vi "EC_Applied_Motion_SXSYSZ_20120115.vi"() -> ()   [LabVIEW 2010]
uses:
  <vilib>/Utility/file.llb/Read From Spreadsheet File (I64).vi
  <vilib>/Utility/file.llb/Read From Spreadsheet File (string).vi
  <vilib>/Instr/_visa.llb/VISA Configure Serial Port (Instr).vi
  <vilib>/Utility/file.llb/Write To Spreadsheet File (I64).vi
  <vilib>/Utility/file.llb/Write To Spreadsheet File (string).vi
panel:
  out "R Velocity MVdeg/sec":dbl format="%.3f"
  out "R Position MV deg":dbl
  out "Z Velocity MV mm/sec":dbl format="%.3f"
  out "Z Position MV mm":dbl
  out "Y Velocity MV mm/sec":dbl format="%.3f"
  out "Y Position MV mm":dbl
  out "X Velocity MV mm/sec":dbl format="%.3f"
  out "X Position MV mm":dbl
  out "Presets":i32[][](array[numeric])
  in  "stop":bool
  in  "Tab Control 3":enum32{"Status", "Reset"}(tab)
  out "Y in Range":bool
  out "Y Scan":bool
  out "Y in Motion":bool
  out "Y Backlash corr":bool
  out "X  in Range":bool
  out "X Scan":bool
  out "X  in Motion":bool
  out "X Backlash corr":bool
  out "Z in Range":bool
  out "Z Scan":bool
  out "Z in Motion":bool
  out "Z Backlash corr":bool
  out "R in Range":bool
  out "R Scan":bool
  out "R in Motion":bool
  out "R Backlash corr":bool
  out "X Ready":bool
  out "Y Ready":bool
  out "Z Ready":bool
  out "R Ready":bool
  in  "Reset Y Position mm":dbl
  out "Reset Y Motor Steps":i32
  in  "Reset X Position mm":dbl
  out "Reset X Motor Steps":i32
  in  "Reset Z Position mm":dbl
  out "Reset Z Motor Steps":i32
  in  "Reset R Position deg":dbl
  out "Reset R Motor Steps":i32
  in  "Reset":bool
  in  "Tab Control 2":enum32{"mm", "step"}(tab)
  in  "X Scan Length SP mm":dbl
  in  "X Scan Velocity SP mm/sec":dbl
  in  "X Scan set":bool
  in  "Y Scan Length SP mm":dbl
  in  "Y Scan Velocity SP mm/sec":dbl
  in  "Y Scan set":bool
  in  "Z Scan Length SP mm":dbl
  in  "Z Scan Velocity SP mm/sec":dbl
  in  "Z Scan set":bool
  in  "R Scan Length SP deg":dbl
  in  "R Scan Velocity SP deg/sec":dbl
  in  "R Scan set":bool
  in  "X Scan Velocity SP steps/sec":i32=1 min=1 max=102400 step=1
  in  "X Scan Length SP steps":i32 min=-500000 max=500000 step=100
  out "X Scan length MV mm":dbl
  out "X Scan velocity MV mm/sec":dbl format="%#_6f"
  in  "Y Scan Velocity SP steps/sec":i32=1 min=1 max=102400 step=1
  in  "Y Scan Length SP steps":i32 min=-1000000 max=0 step=100
  out "Y Scan length MV mm":dbl
  out "Y Scan velocity MV mm/sec":dbl format="%#_6f"
  in  "Z Scan Velocity SP steps/sec":i32=1 min=1 max=102400 step=1
  in  "Z Scan Length SP steps":i32 min=-204724 max=102195276 step=100
  out "Z Scan length MV mm":dbl
  out "Z Scan velocity MV mm/sec":dbl format="%#_6f"
  in  "R Scan Velocity SP steps/sec":i32=1 min=1 max=102400 step=1
  in  "R Scan Length SP steps":i32 min=-6144000 max=0 step=100
  out "R Scan length MV deg":dbl
  out "R Scan velocity MV deg/sec":dbl format="%#_6f"
  out "atan Y/Z":dbl
  in  "Tab Control":enum32{"mm", "preset", "step"}(tab)
  in  "X Position SP mm":dbl
  in  "X Velocity SP mm/sec":dbl
  in  "X Move Set":bool
  in  "Y Move Set":bool
  in  "Y Position SP mm":dbl
  in  "Y Velocity SP mm/sec":dbl
  in  "Z Position SP mm":dbl
  in  "Z Velocity SP mm/sec":dbl
  in  "Z Move Set":bool
  in  "R Position SP deg":dbl
  in  "R Velocity SP deg/sec":dbl
  in  "R Move Set":bool
  in  "Add Button":bool
  in  "String":string
  in  "Delete Button":bool
  in  "Preset positions":i32(ring) items=["ZERO", "Default", "CDOSE", "QMS", "test", "test2", "test3"]
  in  "Set Button":bool
  in  "X Velocity SP step/sec":i32 min=1 max=50000
  in  "Y Velocity SP step/sec":i32 min=1 max=50000
  in  "Z Velocity SP step/sec":i32 min=1 max=5000
  in  "R Velocity SP step/sec":i32 min=1 max=10000
  in  "Y Step SP":i32=-20000 min=-800000 max=800000 step=500
  in  "X Step SP":i32=-20000 min=-750000 max=750000 step=500
  in  "Z Step SP":i32=-20000 min=0 max=102400000 step=500
  in  "R Step SP":i32=-20000 min=-6144000 max=0 step=500
  out "X Step PV":i32 max=2000
  out "Y Step PV":i32 max=2000
  out "Z Step PV":i32 max=2000
  out "R Step PV":i32 max=2000
  out "X Scan Duration":dbl
  out "Y Scan Duration":dbl
  out "Z Scan Duration":dbl
  out "R Scan Duration":dbl
  out "R Backlash steps/sec":i32
  out "R Backlash":i32
  out "R Holding Current %":i32
  out "R Run Current %":i32
  out "R offset deg":dbl
  out "R deg/rev":dbl
  out "R steps/rev":u32
  out "R velocity PV step/sec":i32
  out "R MINPOS":i32=-94296
  out "R MAXPOS":i32=-34296
  out "R COM PORT":refnum<visa-resource-name>="COM5"
  in  "R Scan OK":bool
  in  "R Go":bool
  out "R Position deg PV":dbl
  out "Z COM PORT":refnum<visa-resource-name>="COM5"
  out "Z Backlash steps/sec":i32
  out "Z Backlash":i32
  out "Z Holding Current %":i32
  out "Z Run Current %":i32
  out "Z offset mm":dbl
  out "Z mm/rev":dbl
  out "Z steps/rev":u32
  out "Z  velocity PV step/sec":i32
  out "Z MINPOS":i32=-94296
  out "Z MAXPOS":i32=-34296
  in  "Z Scan OK":bool
  in  "Z Go":bool
  out "Z Position mm PV":dbl
  out "X Position mm PV":dbl
  out "X velocity PV step/sec":i32
  in  "X Scan OK":bool
  in  "X Go":bool
  out "X Backlash steps/sec":i32
  out "X Backlash":i32
  out "X Holding Current %":i32
  out "X Run Current %":i32
  out "X offset mm":dbl
  out "X mm/rev":dbl
  out "X steps/rev":u32
  out "X MAXPOS":i32=-34296
  out "X MINPOS":i32=-94296
  out "X COM PORT":refnum<visa-resource-name>="COM5"
  out "Y Backlash steps/sec":i32
  out "Y Backlash":i32
  out "Y Holding Current %":i32
  out "Y Run Current %":i32
  in  "Scan Cancel":bool
  out "Y Position mm PV":dbl
  out "Y offset mm":dbl
  out "Y mm/rev":dbl
  out "Y steps/rev":u32
  out "Y velocity PV step/sec":i32
  in  "Y Scan OK":bool
  in  "Scan Go":bool
  in  "Stop":bool
  in  "Y Go":bool
  out "Y MINPOS":i32=-94296
  out "Y MAXPOS":i32=-34296
  out "Y COM PORT":refnum<visa-resource-name>="COM5"
  # "Current position"
  # "Goto position"
  # "RX"
  # "RX"
  # "RY"
  # "RY"
  # "RZ"
  # "RZ"
  # "RR"
  # "L"
  # "M"
  # "B"
  # "S"
  # "R"
  # "Preset position"
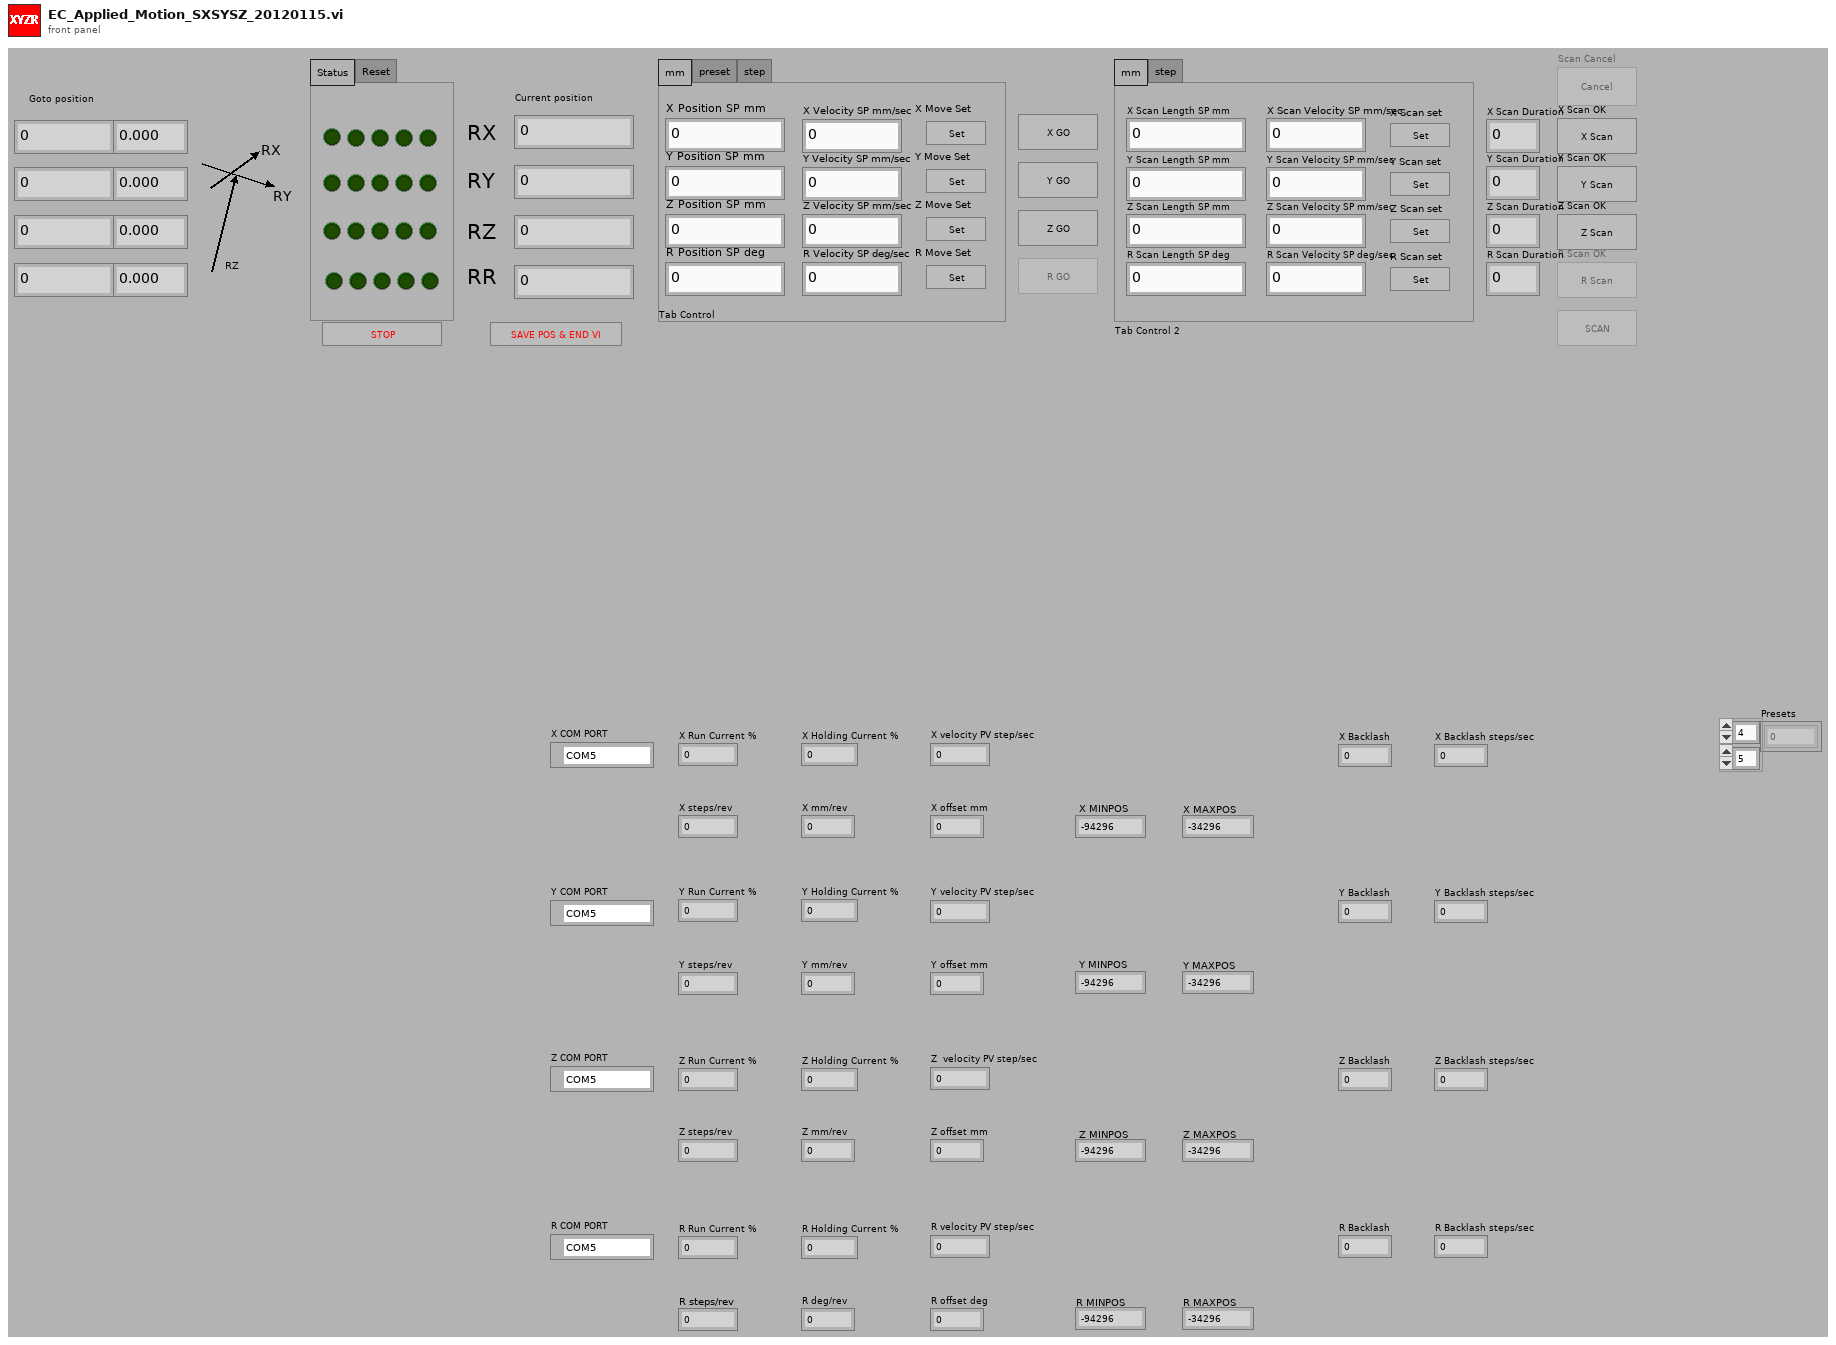
[diagram p1: front panel]
types:
  T1 = enum16{"Power-up Signature", "Accel Rate", "Accel Max", "Bit Rate", "Buffer Status", "Change Current", "Commence Jogging", "Change Jog Speed", "Continue", "Define Address", "Distance for FC,FM,FO,FY", "Decel Rate", "Distance or Position", "Define Limits", "Encoder Deadband", "Encoder Function", "Encoder Position", "Encoder Ratio", "Feed to Length with Speed Change", "Feed to Length", "Feed to Sensor with Mask Dist", "Feed to Length & Set Output", "Feed to Position", "Feed to Sensor", "Feed to Sensor w/safety", "Follow Handwheel", "Immediate Distance?", "Immediate Encoder?", "Immediate Low Output", "Immediate High Output", "Immediate Position?", "Input Status?", "Jog Accel/Decel", "Jog Disable", "Jog Enable", "Jog Speed", "Motor Disable", "Motor Enable", "Microstep Resolution", "Power up Current", "Power up Mode", "Pause", "Request Status", "Revision Level?", "Seek Home", "Stop Jogging", "Stop & Kill Buffer", "Set Output", "Set ABS Position", "Send String", "Stop", "Velocity for Speed Change", "Velocity Setting", "Wait for Input", "Wait Time"}
  T2 = enum8{"Enabled", "Disabled", "Disabled and Grayed Out"}
  T3 = cluster{"first row[0]":i64, "first row[1]":i64, "first row[2]":i64, "first row[3]":i64, "first row[4]":i64, "first row[5]":i64, "first row[6]":i64, "first row[7]":i64, "first row[8]":i64}
  T4 = cluster{"Value[0]":i32, "Value[1]":i32, "Value[2]":i32, "Value[3]":i32, "Value[4]":i32, "Value[5]":i32, "Value[6]":i32, "Value[7]":i32, "Value[8]":i32}
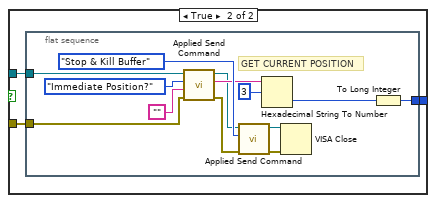
[diagram p2: hidden frame]
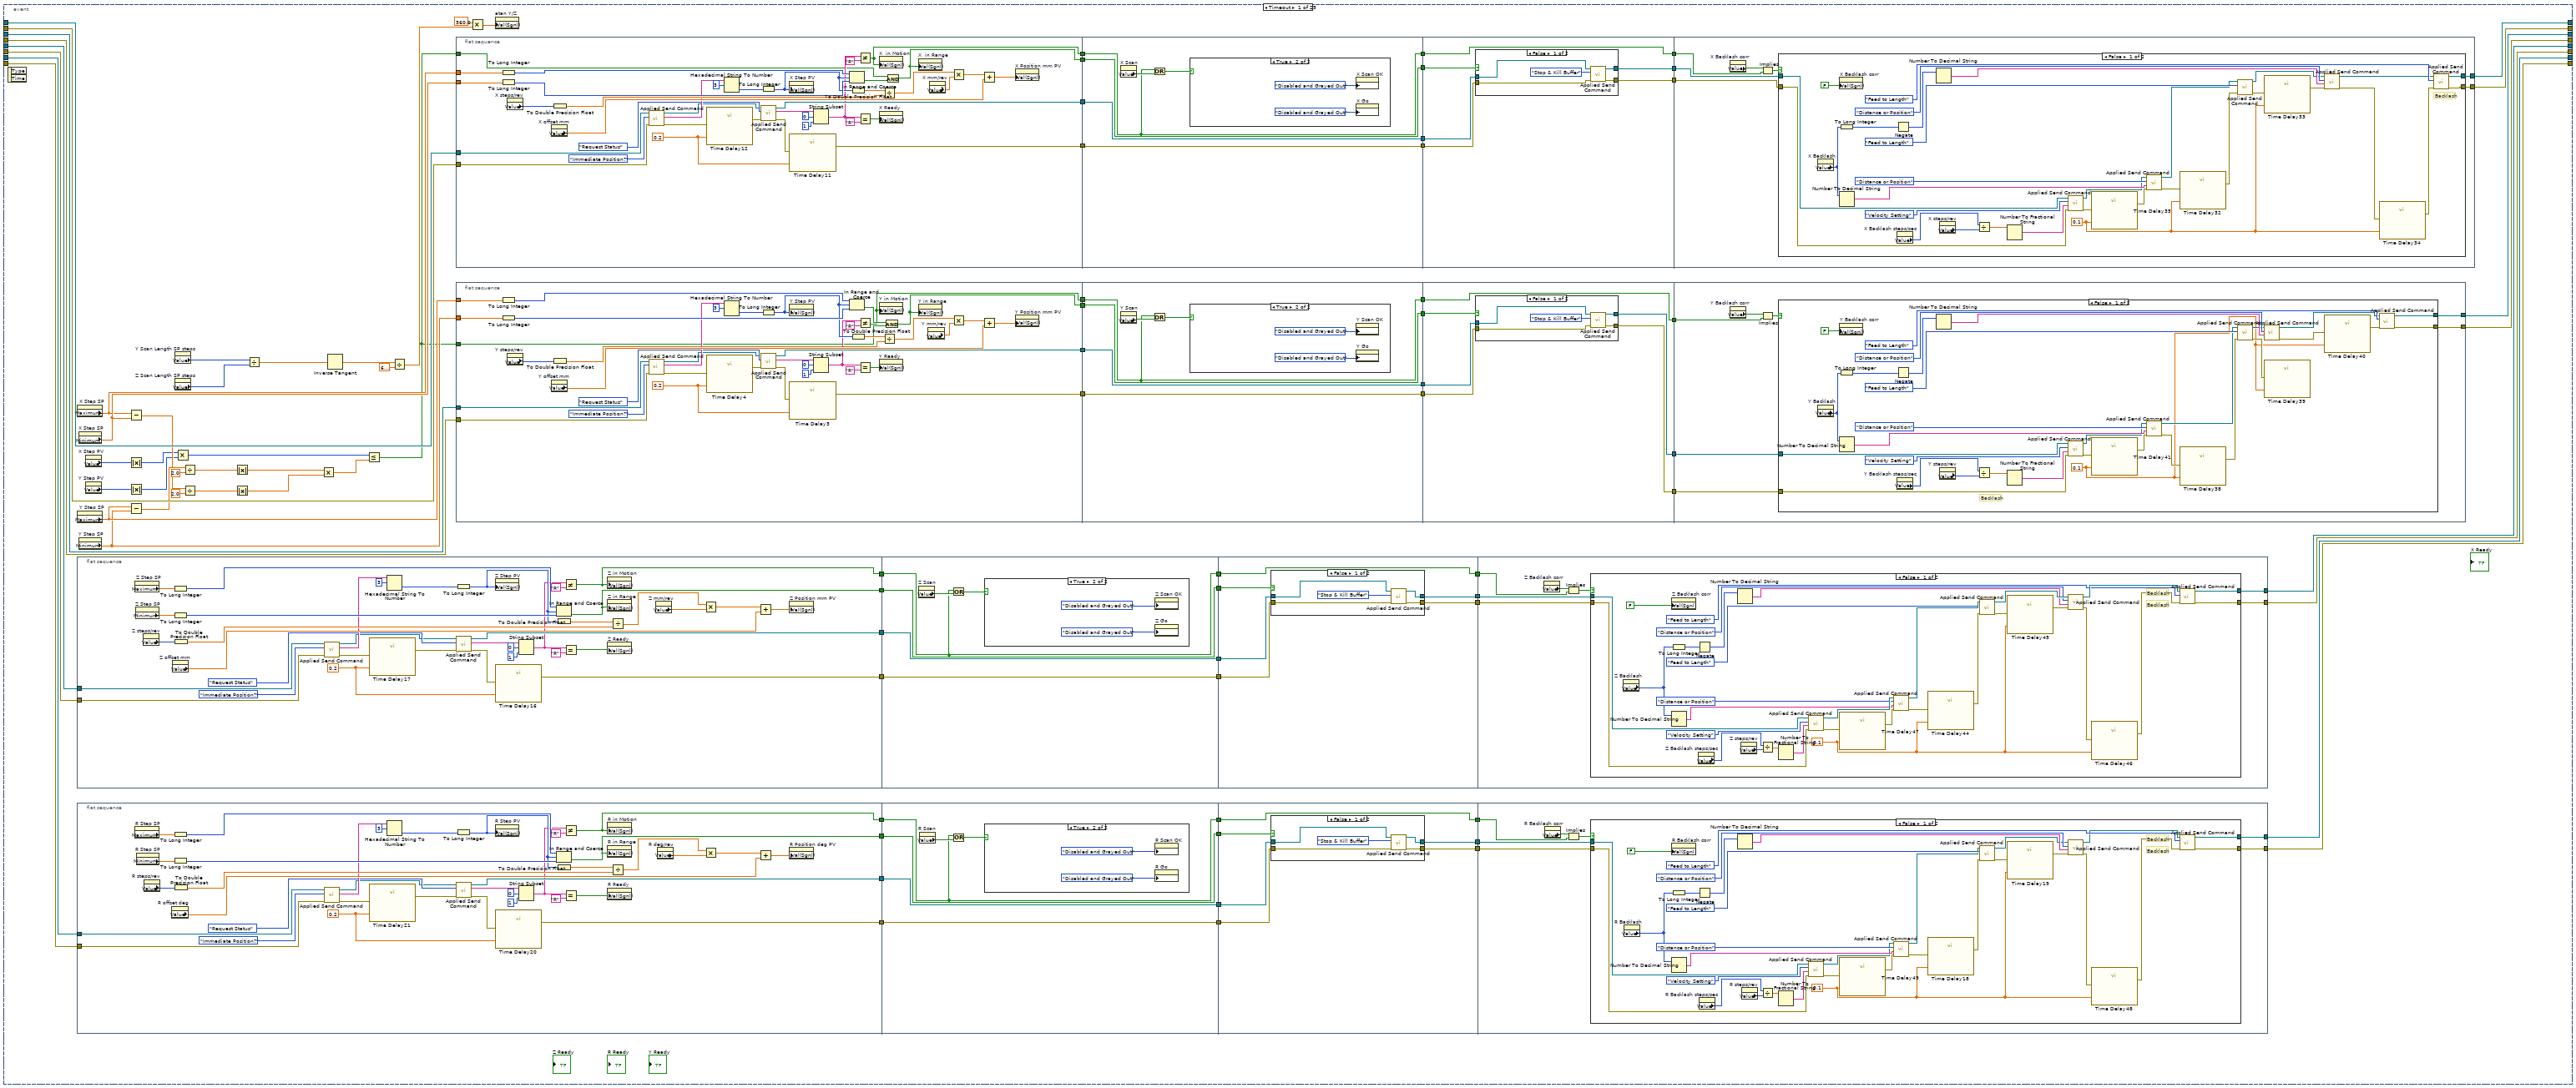
[diagram p6: hidden frame]
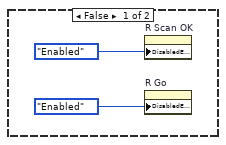
[diagram p7: hidden frame]
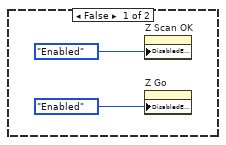
[diagram p10: hidden frame]
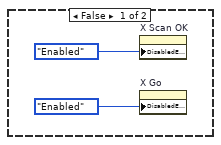
[diagram p13: hidden frame]
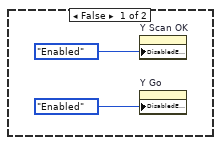
[diagram p16: hidden frame]
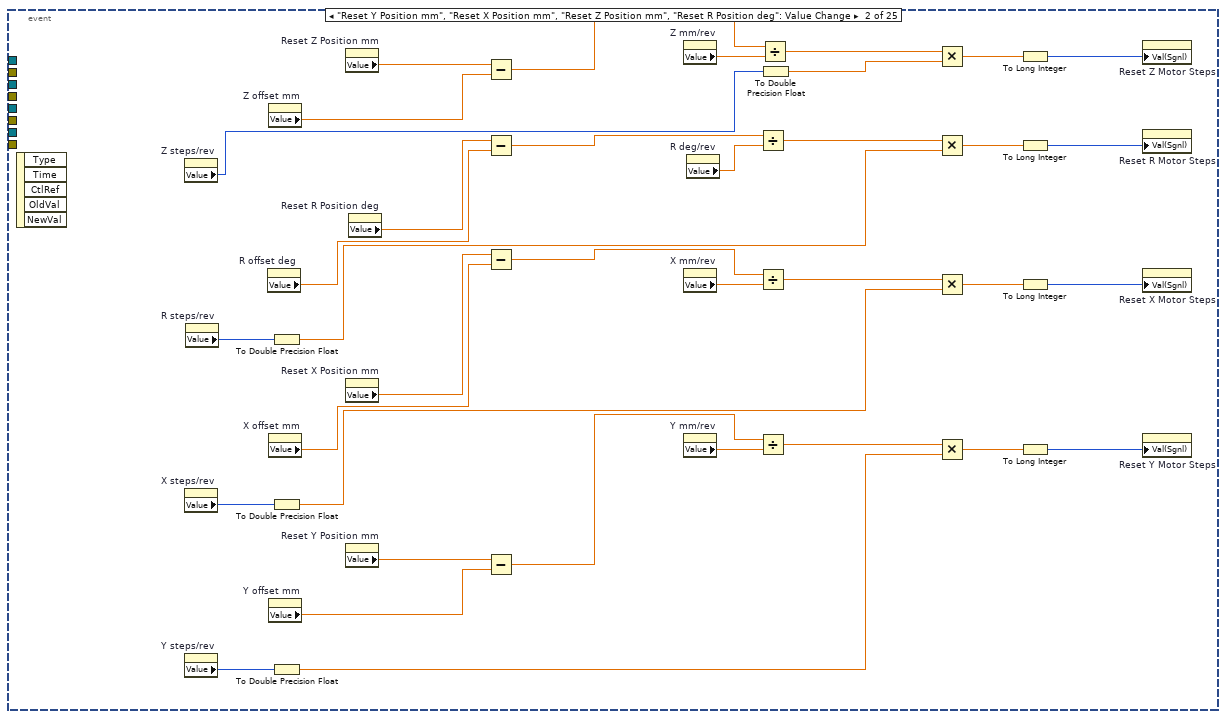
[diagram p19: hidden frame]
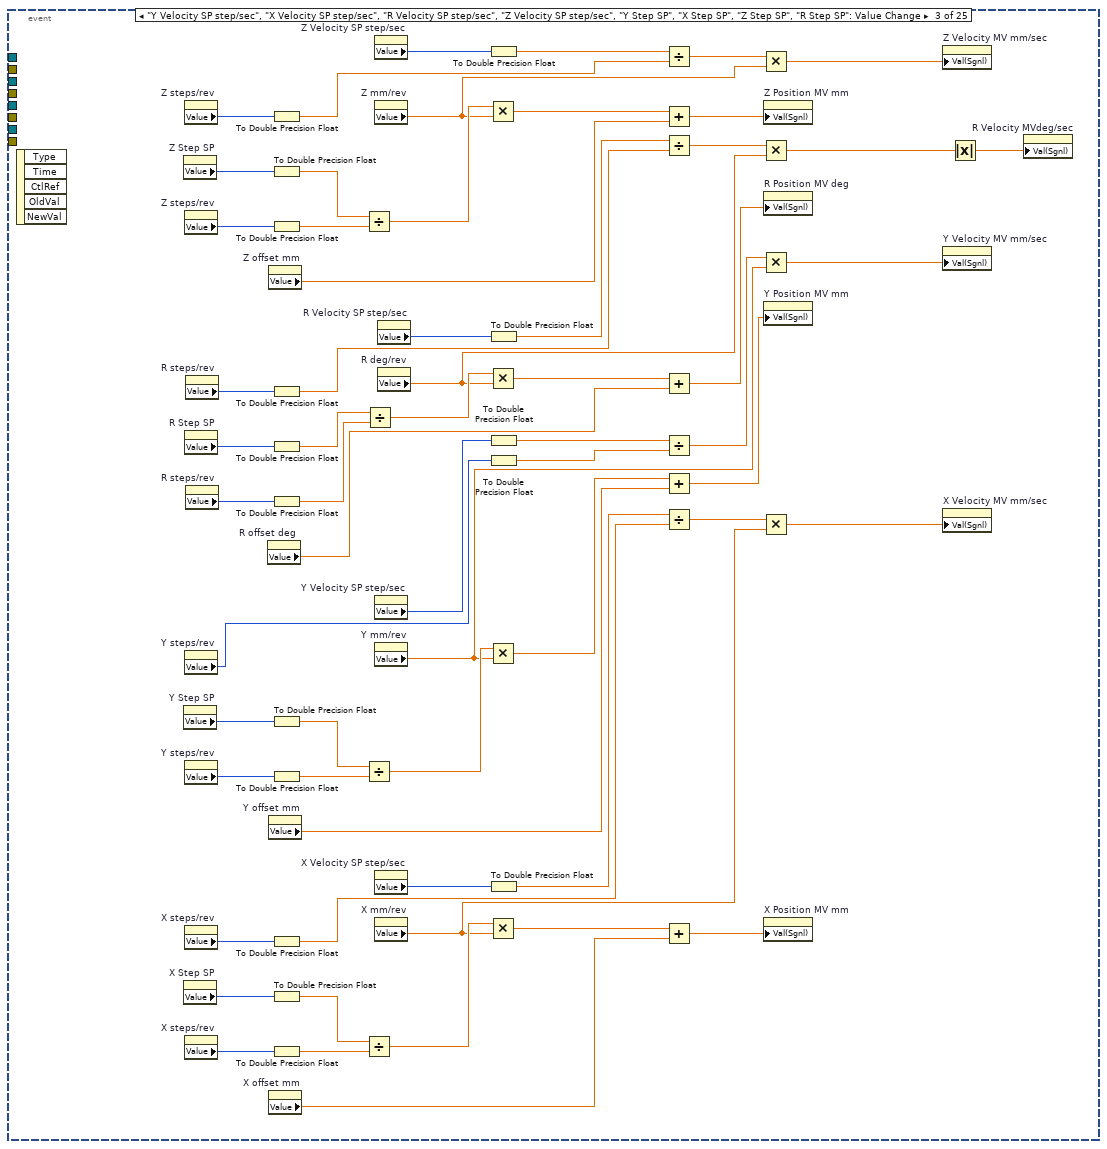
[diagram p20: hidden frame]
diagram:
  w25 = 0 ("dimension size")
  n1 = flat-sequence {
    tunnel: [w94] -> w11
    tunnel: [w93] -> w10
    tunnel: w11 -> [w108]
    tunnel: w10 -> [w107]
    tunnel: [w106] -> w9
    tunnel: [w105] -> w8
    tunnel: [w116] -> w65
    tunnel: [w115] -> w64
    tunnel: w9 -> [w118]
    tunnel: w8 -> [w117]
    tunnel: w65 -> [w133]
    tunnel: w64 -> [w132]
    tunnel: [w134] -> w63
    tunnel: [w135] -> w62
    tunnel: [w136] -> w7
    tunnel: [w147] -> w56
    tunnel: [w148] -> w57
    tunnel: w63 -> [w148]
    tunnel: w62 -> [w147]
    tunnel: w7 -> [w145]
    frame #0 {
      "Z Run Current %" <- 100 ("Z Run Current %")
      "Z Holding Current %" <- 50 ("Z Holding Current %")
    }
    frame #1 {
      "Z Backlash steps/sec" <- 1000 ("Z Backlash steps/sec")
      "Z Backlash" <- -5000 ("Z Backlash")
    }
    frame #2 {
      w84 = 2.54 ("Z mm/rev")
      w83 = u32 20000 ("step/rev")
      w85 = 5000 ("Value (Signaling)")
      n2 = property on="Z Scan Velocity SP mm/sec" class="DigNum (strict)"("Val(Sgnl)"=0.1 ("Value (Signaling)")) -> ()  [unwired: 2 in, 2 out]
      n3 = property on="Z Velocity SP step/sec" class="DigNum (strict)"("Val(Sgnl)"=w85) -> ()  [unwired: 2 in, 2 out]
      n4 = property on="Z Velocity SP step/sec" class="DigNum (strict)"("Minimum"=1.0 ("Data Entry Limits:Minimum")) -> ()  [unwired: 2 in, 2 out]
      n5 = To Double Precision Float(number=w85) -> (double precision float=w89:dbl)
      n6 = To Double Precision Float(number=w83) -> (double precision float=w88:dbl)
      n7 = property on="Z Velocity SP step/sec" class="DigNum (strict)"("Maximum"=w89) -> ()  [unwired: 2 in, 2 out]
      n8 = Divide(x=w89, y=w88) -> (x/y=w86:dbl)
      n9 = Multiply(x=w86, y=w84) -> (x*y=w87:dbl)
      n10 = property on="Z Velocity SP mm/sec" class="DigNum (strict)"("Val(Sgnl)"=w87) -> ()  [unwired: 2 in, 2 out]
      "Z mm/rev" <- w84
      "Z steps/rev" <- w83
    }
    frame #3 {
      w91 = 0 ("lower limit")
      w90 = 102400000 ("upper limit")
      n11 = property on="Z Step SP" class="DigNum (strict)"("Minimum"=w91) -> ()  [unwired: 2 in, 2 out]
      n12 = property on="Z Step SP" class="DigNum (strict)"("Maximum"=w90) -> ()  [unwired: 2 in, 2 out]
      "Z offset mm" <- 0.0 ("Z offset mm")
      "Z MINPOS" <- w91
      "Z MAXPOS" <- w90
    }
    frame #4 {
      w101 = refnum<visa-resource-name> "COM15" ("COM PORT")
      w99 = u16 0 items=["None", "XON/XOFF", "RTS/CTS", "XON/XOFF & RTS/CTS", "DTR/DSR", "XON/XOFF & DTR/DSR"] ("flow control (0:none)")
      w98 = u16 10 items=["1.0"=10, "1.5"=15, "2.0"=20] ("stop bits (10: 1 bit)")
      # "Stop bits"
      n13 = call-poly "VISA Configure Serial Port"("VISA resource name"=w101, "timeout (10sec)"=u32 10000, "baud rate (9600)"=u32 9600, "data bits (8)"=u16 8, "parity (0:none)"=enum16{"None", "Odd", "Even", "Mark", "Space"}."None", "stop bits (10: 1 bit)"=w98, "flow control (0:none)"=w99) -> ("VISA resource name out"=w94:refnum<visa-resource-name>, "error out"=w93:errorcluster)  [unwired: 7 in]
      "Z COM PORT" <- w101
    }
    frame #5 {
      # "Run Current %"
      n14 = property on="Z Run Current %" class="DigNum (strict)"() -> ("Value"=w109:i32)  [unwired: 2 in, 2 out]
      n15 = Divide(x=w109, y=100) -> (x/y=w110:dbl)
      n16 = Multiply(x=w110, y=3.5) -> (x*y=w104:dbl)
      n17 = Number To Fractional String(number=w104) -> (F-format string=w111:string)  [unwired: 3 in]
      n18 = call "Applied Send Command.vi"("error in (no error)"=w107, "Extra"=w111, "Command"=T1."Change Current", "VISA resource name"=w108) -> ("error out"=w105:errorcluster, "VISA resource name out"=w106:refnum<visa-resource-name>)  [unwired: 3 in, 1 out]
    }
    frame #6 {
      # "VELOCITY"
      n19 = property on="Z steps/rev" class="DigNum (strict)"() -> ("Value"=w114:u32)  [unwired: 2 in, 2 out]
      n20 = property on="Z Velocity SP step/sec" class="DigNum (strict)"() -> ("Value"=w113:i32)  [unwired: 2 in, 2 out]
      n21 = Divide(x=w113, y=w114) -> (x/y=w121:dbl)
      n22 = Number To Fractional String(number=w121) -> (F-format string=w123:string)  [unwired: 3 in]
      n23 = call "Applied Send Command.vi"("error in (no error)"=w117, "Extra"=w123, "Command"=T1."Velocity Setting", "VISA resource name"=w118) -> ("error out"=w124:errorcluster, "VISA resource name out"=w131:refnum<visa-resource-name>)  [unwired: 3 in, 1 out]
      n24 = call "Time Delay2"("error in (no error)"=w124, "Delay Time (s)"=0.1) -> ("error out"=w129:errorcluster)  [unwired: 9 in]
      n25 = call "Applied Send Command.vi"("error in (no error)"=w129, "Extra"="", "Command"=T1."Velocity Setting", "VISA resource name"=w131) -> ("error out"=w115:errorcluster, "read buffer"=w127:string, "VISA resource name out"=w116:refnum<visa-resource-name>)  [unwired: 3 in]
      n26 = Fract/Exp String To Number(string=w127, offset=3) -> (number=w122:dbl)  [unwired: 2 in, 1 out]
      n27 = Multiply(x=w122, y=w114) -> (x*y=w119:dbl)
      n28 = property on="Z  velocity PV step/sec" class="DigNum (strict)"("Val(Sgnl)"=w119) -> ()  [unwired: 2 in, 2 out]
    }
    frame #7 {
      # "GET CURRENT POSITION"
      n29 = call "Applied Send Command.vi"("error in (no error)"=w132, "Extra"="", "Command"=T1."Immediate Position?", "VISA resource name"=w133) -> ("error out"=w138:errorcluster, "read buffer"=w140:string, "VISA resource name out"=w134:refnum<visa-resource-name>)  [unwired: 3 in]
      n30 = call "Time Delay8"("error in (no error)"=w138, "Delay Time (s)"=0.1) -> ("error out"=w135:errorcluster)  [unwired: 9 in]
      n31 = Hexadecimal String To Number(string=w140, offset=3) -> (number=w136:u32)  [unwired: 1 in, 1 out]
    }
    frame #8 {
      n32 = property on="Z Step SP" class="DigNum (strict)"() -> ("Maximum"=w144:dbl)  [unwired: 2 in, 2 out]
      n33 = property on="Z Step SP" class="DigNum (strict)"("Val(Sgnl)"=w145) -> ()  [unwired: 2 in, 2 out]
      n34 = property on="Z Step SP" class="DigNum (strict)"() -> ("Minimum"=w143:dbl)  [unwired: 2 in, 2 out]
      n35 = In Range and Coerce(upper limit=w144, x=w145, lower limit=w143) -> (In Range?=w146:bool)  [unwired: 1 out]
      n36 = property on="Z in Range" class="Bool (strict)"("Val(Sgnl)"=w146) -> ()  [unwired: 2 in, 2 out]
    }
  }
  n37 = flat-sequence {
    tunnel: [w167] -> w4
    tunnel: [w166] -> w3
    tunnel: [w181] -> w6
    tunnel: [w180] -> w5
    tunnel: w4 -> [w179]
    tunnel: w3 -> [w178]
    tunnel: [w188] -> w61
    tunnel: [w189] -> w60
    tunnel: w6 -> [w186]
    tunnel: w5 -> [w187]
    tunnel: w61 -> [w206]
    tunnel: w60 -> [w205]
    tunnel: [w207] -> w59
    tunnel: [w209] -> w58
    tunnel: [w208] -> w2
    tunnel: [w220] -> w54
    tunnel: [w221] -> w55
    tunnel: w59 -> [w220]
    tunnel: w58 -> [w218]
    tunnel: w2 -> [w221]
    frame #0 {
      "R Run Current %" <- 100 ("R Run Current %")
      "R Holding Current %" <- 50 ("R Holding Current %")
    }
    frame #1 {
      "R Backlash" <- -12800 ("R Backlash")
      "R Backlash steps/sec" <- 6400 ("R Backlash steps/sec")
    }
    frame #2 {
      w157 = -3.0 ("R deg/rev")
      w159 = u32 20000 ("step/rev")
      w155 = 10000 ("Value (Signaling)")
      n38 = property on="R Velocity SP step/sec" class="DigNum (strict)"("Minimum"=1.0 ("Data Entry Limits:Minimum")) -> ()  [unwired: 2 in, 2 out]
      n39 = property on="R Velocity SP step/sec" class="DigNum (strict)"("Val(Sgnl)"=w155) -> ()  [unwired: 2 in, 2 out]
      n40 = property on="R Velocity SP deg/sec" class="DigNum (strict)"("Val(Sgnl)"=0.1 ("Value (Signaling)")) -> ()  [unwired: 2 in, 2 out]
      n41 = To Double Precision Float(number=w155) -> (double precision float=w153:dbl)
      n42 = To Double Precision Float(number=w159) -> (double precision float=w158:dbl)
      n43 = property on="R Velocity SP step/sec" class="DigNum (strict)"("Maximum"=w153) -> ()  [unwired: 2 in, 2 out]
      n44 = Divide(x=w153, y=w158) -> (x/y=w154:dbl)
      n45 = Multiply(x=w154, y=w157) -> (x*y=w156:dbl)
      n46 = Absolute Value(x=w156) -> (abs(x)=w161:dbl)
      n47 = property on="R Velocity SP deg/sec" class="DigNum (strict)"("Val(Sgnl)"=w161) -> ()  [unwired: 2 in, 2 out]
      "R deg/rev" <- w157
      "R steps/rev" <- w159
    }
    frame #3 {
      w164 = 0 ("upper limit")
      w165 = -6144000 ("lower limit")
      n48 = property on="R Step SP" class="DigNum (strict)"("Minimum"=w165) -> ()  [unwired: 2 in, 2 out]
      n49 = property on="R Step SP" class="DigNum (strict)"("Maximum"=w164) -> ()  [unwired: 2 in, 2 out]
      "R MINPOS" <- w164
      "R MAXPOS" <- w165
      "R offset deg" <- 0.0 ("R offset deg")
    }
    frame #4 {
      w174 = refnum<visa-resource-name> "COM19" ("COM PORT")
      w172 = u16 0 items=["None", "XON/XOFF", "RTS/CTS", "XON/XOFF & RTS/CTS", "DTR/DSR", "XON/XOFF & DTR/DSR"] ("flow control (0:none)")
      w171 = u16 10 items=["1.0"=10, "1.5"=15, "2.0"=20] ("stop bits (10: 1 bit)")
      # "Stop bits"
      n50 = call-poly "VISA Configure Serial Port"("VISA resource name"=w174, "timeout (10sec)"=u32 10000, "baud rate (9600)"=u32 9600, "data bits (8)"=u16 8, "parity (0:none)"=enum16{"None", "Odd", "Even", "Mark", "Space"}."None", "stop bits (10: 1 bit)"=w171, "flow control (0:none)"=w172) -> ("VISA resource name out"=w167:refnum<visa-resource-name>, "error out"=w166:errorcluster)  [unwired: 7 in]
      "R COM PORT" <- w174
    }
    frame #5 {
      # "Run Current %"
      n51 = property on="R Run Current %" class="DigNum (strict)"() -> ("Value"=w182:i32)  [unwired: 2 in, 2 out]
      n52 = Divide(x=w182, y=100) -> (x/y=w183:dbl)
      n53 = Multiply(x=w183, y=3.5) -> (x*y=w177:dbl)
      n54 = Number To Fractional String(number=w177) -> (F-format string=w184:string)  [unwired: 3 in]
      n55 = call "Applied Send Command.vi"("error in (no error)"=w178, "Extra"=w184, "Command"=T1."Change Current", "VISA resource name"=w179) -> ("error out"=w180:errorcluster, "VISA resource name out"=w181:refnum<visa-resource-name>)  [unwired: 3 in, 1 out]
    }
    frame #6 {
      # "VELOCITY"
      n56 = property on="R steps/rev" class="DigNum (strict)"() -> ("Value"=w192:u32)  [unwired: 2 in, 2 out]
      n57 = property on="R Velocity SP step/sec" class="DigNum (strict)"() -> ("Value"=w190:i32)  [unwired: 2 in, 2 out]
      n58 = Divide(x=w190, y=w192) -> (x/y=w194:dbl)
      n59 = Number To Fractional String(number=w194) -> (F-format string=w196:string)  [unwired: 3 in]
      n60 = call "Applied Send Command.vi"("error in (no error)"=w187, "Extra"=w196, "Command"=T1."Velocity Setting", "VISA resource name"=w186) -> ("error out"=w197:errorcluster, "VISA resource name out"=w204:refnum<visa-resource-name>)  [unwired: 3 in, 1 out]
      n61 = call "Time Delay43"("error in (no error)"=w197, "Delay Time (s)"=0.1) -> ("error out"=w202:errorcluster)  [unwired: 9 in]
      n62 = call "Applied Send Command.vi"("error in (no error)"=w202, "Extra"="", "Command"=T1."Velocity Setting", "VISA resource name"=w204) -> ("error out"=w189:errorcluster, "read buffer"=w200:string, "VISA resource name out"=w188:refnum<visa-resource-name>)  [unwired: 3 in]
      n63 = Fract/Exp String To Number(string=w200, offset=3) -> (number=w195:dbl)  [unwired: 2 in, 1 out]
      n64 = Multiply(x=w195, y=w192) -> (x*y=w191:dbl)
      n65 = property on="R velocity PV step/sec" class="DigNum (strict)"("Val(Sgnl)"=w191) -> ()  [unwired: 2 in, 2 out]
    }
    frame #7 {
      # "GET CURRENT POSITION"
      n66 = call "Applied Send Command.vi"("error in (no error)"=w205, "Extra"="", "Command"=T1."Immediate Position?", "VISA resource name"=w206) -> ("error out"=w211:errorcluster, "read buffer"=w213:string, "VISA resource name out"=w208:refnum<visa-resource-name>)  [unwired: 3 in]
      n67 = call "Time Delay42"("error in (no error)"=w211, "Delay Time (s)"=0.1) -> ("error out"=w207:errorcluster)  [unwired: 9 in]
      n68 = Hexadecimal String To Number(string=w213, offset=3) -> (number=w209:u32)  [unwired: 1 in, 1 out]
    }
    frame #8 {
      n69 = property on="R Step SP" class="DigNum (strict)"() -> ("Maximum"=w216:dbl)  [unwired: 2 in, 2 out]
      n70 = property on="R Step SP" class="DigNum (strict)"("Val(Sgnl)"=w218) -> ()  [unwired: 2 in, 2 out]
      n71 = property on="R Step SP" class="DigNum (strict)"() -> ("Minimum"=w217:dbl)  [unwired: 2 in, 2 out]
      n72 = In Range and Coerce(upper limit=w216, x=w218, lower limit=w217) -> (In Range?=w219:bool)  [unwired: 1 out]
      n73 = property on="R in Range" class="Bool (strict)"("Val(Sgnl)"=w219) -> ()  [unwired: 2 in, 2 out]
    }
  }
  n74 = flat-sequence {
    frame #0 {
      n75 = property on="X Scan" class="Bool (strict)"("Val(Sgnl)"=FALSE ("Value (Signaling)")) -> ()  [unwired: 2 in, 2 out]
      n76 = property on="Y Scan" class="Bool (strict)"("Val(Sgnl)"=FALSE ("Value (Signaling)")) -> ()  [unwired: 2 in, 2 out]
      n77 = property on="Z Scan" class="Bool (strict)"("Val(Sgnl)"=FALSE ("Value (Signaling)")) -> ()  [unwired: 2 in, 2 out]
      n78 = property on="R Scan" class="Bool (strict)"("Val(Sgnl)"=FALSE ("Value (Signaling)")) -> ()  [unwired: 2 in, 2 out]
      n79 = property on="Scan Go" class="Bool"("DisabledEnum"=T2."Disabled and Grayed Out" ("Disabled")) -> ()  [unwired: 2 in, 2 out]
      n80 = property on="Scan Cancel" class="Bool"("DisabledEnum"=T2."Disabled and Grayed Out" ("Disabled")) -> ()  [unwired: 2 in, 2 out]
    }
    frame #1 {
      n81 = property on="Y Backlash corr" class="Bool (strict)"("Val(Sgnl)"=FALSE ("Value (Signaling)")) -> ()  [unwired: 2 in, 2 out]
      n82 = property on="R Backlash corr" class="Bool (strict)"("Val(Sgnl)"=FALSE ("Value (Signaling)")) -> ()  [unwired: 2 in, 2 out]
      n83 = property on="X Backlash corr" class="Bool (strict)"("Val(Sgnl)"=FALSE ("Value (Signaling)")) -> ()  [unwired: 2 in, 2 out]
      n84 = property on="Z Backlash corr" class="Bool (strict)"("Val(Sgnl)"=FALSE ("Value (Signaling)")) -> ()  [unwired: 2 in, 2 out]
    }
  }
  n85 = flat-sequence {
    tunnel: [w249] -> w19
    tunnel: [w248] -> w18
    tunnel: w19 -> [w263]
    tunnel: w18 -> [w262]
    tunnel: [w261] -> w17
    tunnel: [w260] -> w16
    tunnel: w17 -> [w271]
    tunnel: w16 -> [w270]
    tunnel: [w269] -> w15
    tunnel: [w268] -> w14
    tunnel: [w288] -> w69
    tunnel: w15 -> [w291]
    tunnel: w14 -> [w290]
    tunnel: [w289] -> w13
    tunnel: [w287] -> w12
    tunnel: [w300] -> w75
    tunnel: [w303] -> w76
    tunnel: w69 -> [w300]
    tunnel: w13 -> [w303]
    tunnel: w12 -> [w301]
    frame #0 {
      "Y Run Current %" <- 100 ("Run Current %")
      "Y Holding Current %" <- 50 ("Holding Current %")
    }
    frame #1 {
      "Y Backlash" <- 5000 ("Backlash2")
      "Y Backlash steps/sec" <- 10000 ("Value (Signaling)")
    }
    frame #2 {
      w239 = 0.21167 ("MM/rev")
      w242 = u32 20000 ("step/rev")
      w237 = 50000 ("Value (Signaling)")
      n86 = property on="Y Velocity SP step/sec" class="DigNum (strict)"("Minimum"=1.0 ("Data Entry Limits:Minimum")) -> ()  [unwired: 2 in, 2 out]
      n87 = property on="Y Scan Velocity SP mm/sec" class="DigNum (strict)"("Val(Sgnl)"=0.1 ("Value (Signaling)")) -> ()  [unwired: 2 in, 2 out]
      n88 = property on="Y Velocity SP step/sec" class="DigNum (strict)"("Val(Sgnl)"=w237) -> ()  [unwired: 2 in, 2 out]
      n89 = To Double Precision Float(number=w237) -> (double precision float=w243:dbl)
      n90 = To Double Precision Float(number=w242) -> (double precision float=w241:dbl)
      n91 = property on="Y Velocity SP step/sec" class="DigNum (strict)"("Maximum"=w243) -> ()  [unwired: 2 in, 2 out]
      n92 = Divide(x=w243, y=w241) -> (x/y=w238:dbl)
      n93 = Multiply(x=w238, y=w239) -> (x*y=w240:dbl)
      n94 = property on="Y Velocity SP mm/sec" class="DigNum (strict)"("Val(Sgnl)"=w240) -> ()  [unwired: 2 in, 2 out]
      "Y steps/rev" <- w242
      "Y mm/rev" <- w239
    }
    frame #3 {
      w246 = -800000 ("lower limit")
      w247 = 800000 ("upper limit")
      n95 = property on="Y Step SP" class="DigNum (strict)"("Minimum"=w246) -> ()  [unwired: 2 in, 2 out]
      n96 = property on="Y Step SP" class="DigNum (strict)"("Maximum"=w247) -> ()  [unwired: 2 in, 2 out]
      "Y MAXPOS" <- w247
      "Y MINPOS" <- w246
      "Y offset mm" <- 0.0 ("offset")
    }
    frame #4 {
      w256 = refnum<visa-resource-name> "COM14" ("COM PORT")
      w254 = u16 0 items=["None", "XON/XOFF", "RTS/CTS", "XON/XOFF & RTS/CTS", "DTR/DSR", "XON/XOFF & DTR/DSR"] ("flow control (0:none)")
      w253 = u16 10 items=["1.0"=10, "1.5"=15, "2.0"=20] ("stop bits (10: 1 bit)")
      # "Stop bits"
      n97 = call-poly "VISA Configure Serial Port"("VISA resource name"=w256, "timeout (10sec)"=u32 10000, "baud rate (9600)"=u32 9600, "data bits (8)"=u16 8, "parity (0:none)"=enum16{"None", "Odd", "Even", "Mark", "Space"}."None", "stop bits (10: 1 bit)"=w253, "flow control (0:none)"=w254) -> ("VISA resource name out"=w249:refnum<visa-resource-name>, "error out"=w248:errorcluster)  [unwired: 7 in]
      "Y COM PORT" <- w256
    }
    frame #5 {
      n98 = property on="Y Run Current %" class="DigNum (strict)"() -> ("Value"=w264:i32)  [unwired: 2 in, 2 out]
      n99 = Divide(x=w264, y=100) -> (x/y=w265:dbl)
      n100 = Multiply(x=w265, y=3.5) -> (x*y=w259:dbl)
      n101 = Number To Fractional String(number=w259) -> (F-format string=w266:string)  [unwired: 3 in]
      n102 = call "Applied Send Command.vi"("error in (no error)"=w262, "Extra"=w266, "Command"=T1."Change Current", "VISA resource name"=w263) -> ("error out"=w260:errorcluster, "VISA resource name out"=w261:refnum<visa-resource-name>)  [unwired: 3 in, 1 out]
    }
    frame #6 {
      # "VELOCITY"
      n103 = property on="Y steps/rev" class="DigNum (strict)"() -> ("Value"=w275:u32)  [unwired: 2 in, 2 out]
      n104 = property on="Y Velocity SP step/sec" class="DigNum (strict)"() -> ("Value"=w272:i32)  [unwired: 2 in, 2 out]
      n105 = Divide(x=w272, y=w275) -> (x/y=w274:dbl)
      n106 = Number To Fractional String(number=w274) -> (F-format string=w278:string)  [unwired: 3 in]
      n107 = call "Applied Send Command.vi"("error in (no error)"=w270, "Extra"=w278, "Command"=T1."Velocity Setting", "VISA resource name"=w271) -> ("error out"=w279:errorcluster, "VISA resource name out"=w286:refnum<visa-resource-name>)  [unwired: 3 in, 1 out]
      n108 = call "Time Delay36"("error in (no error)"=w279, "Delay Time (s)"=0.1) -> ("error out"=w284:errorcluster)  [unwired: 9 in]
      n109 = call "Applied Send Command.vi"("error in (no error)"=w284, "Extra"="", "Command"=T1."Velocity Setting", "VISA resource name"=w286) -> ("error out"=w268:errorcluster, "read buffer"=w282:string, "VISA resource name out"=w269:refnum<visa-resource-name>)  [unwired: 3 in]
      n110 = Fract/Exp String To Number(string=w282, offset=3) -> (number=w277:dbl)  [unwired: 2 in, 1 out]
      n111 = Multiply(x=w277, y=w275) -> (x*y=w276:dbl)
      n112 = property on="Y velocity PV step/sec" class="DigNum (strict)"("Val(Sgnl)"=w276) -> ()  [unwired: 2 in, 2 out]
    }
    frame #7 {
      # "GET CURRENT POSITION"
      n113 = call "Applied Send Command.vi"("error in (no error)"=w290, "Extra"="", "Command"=T1."Immediate Position?", "VISA resource name"=w291) -> ("error out"=w293:errorcluster, "read buffer"=w295:string, "VISA resource name out"=w289:refnum<visa-resource-name>)  [unwired: 3 in]
      n114 = call "Time Delay37"("error in (no error)"=w293, "Delay Time (s)"=0.1) -> ("error out"=w288:errorcluster)  [unwired: 9 in]
      n115 = Hexadecimal String To Number(string=w295, offset=3) -> (number=w287:u32)  [unwired: 1 in, 1 out]
    }
    frame #8 {
      n116 = property on="Y Step SP" class="DigNum (strict)"() -> ("Maximum"=w299:dbl)  [unwired: 2 in, 2 out]
      n117 = property on="Y Step SP" class="DigNum (strict)"("Val(Sgnl)"=w301) -> ()  [unwired: 2 in, 2 out]
      n118 = property on="Y Step SP" class="DigNum (strict)"() -> ("Minimum"=w298:dbl)  [unwired: 2 in, 2 out]
      n119 = In Range and Coerce(upper limit=w299, x=w301, lower limit=w298) -> (In Range?=w302:bool)  [unwired: 1 out]
      n120 = property on="Y in Range" class="Bool (strict)"("Val(Sgnl)"=w302) -> ()  [unwired: 2 in, 2 out]
    }
  }
  n121 = flat-sequence {
    tunnel: [w321] -> w24
    tunnel: [w320] -> w23
    tunnel: w24 -> [w338]
    tunnel: w23 -> [w337]
    tunnel: [w336] -> w22
    tunnel: [w335] -> w21
    tunnel: [w341] -> w74
    tunnel: w22 -> [w349]
    tunnel: w21 -> [w348]
    tunnel: [w342] -> w20
    tunnel: w74 -> [w363]
    tunnel: [w362] -> w68
    tunnel: [w360] -> w67
    tunnel: [w365] -> w66
    tunnel: w20 -> [w364]
    tunnel: [w374] -> w72
    tunnel: [w375] -> w73
    tunnel: w68 -> [w375]
    tunnel: w67 -> [w374]
    tunnel: w66 -> [w370]
    frame #0 {
      "X Run Current %" <- 100 ("Run Current %")
      "X Holding Current %" <- 50 ("Holding Current %")
    }
    frame #1 {
      "X Backlash steps/sec" <- 10000 ("Value (Signaling)")
      "X Backlash" <- 5000 ("Backlash2")
    }
    frame #2 {
      w310 = 0.21167 ("MM/rev")
      w313 = u32 20000 ("step/rev")
      w308 = 50000 ("Value (Signaling)")
      n122 = property on="X Velocity SP step/sec" class="DigNum (strict)"("Minimum"=1.0 ("Data Entry Limits:Minimum")) -> ()  [unwired: 2 in, 2 out]
      n123 = property on="X Velocity SP step/sec" class="DigNum (strict)"("Val(Sgnl)"=w308) -> ()  [unwired: 2 in, 2 out]
      n124 = property on="X Scan Velocity SP mm/sec" class="DigNum (strict)"("Val(Sgnl)"=0.1 ("Value (Signaling)")) -> ()  [unwired: 2 in, 2 out]
      n125 = To Double Precision Float(number=w308) -> (double precision float=w314:dbl)
      n126 = To Double Precision Float(number=w313) -> (double precision float=w312:dbl)
      n127 = property on="X Velocity SP step/sec" class="DigNum (strict)"("Maximum"=w314) -> ()  [unwired: 2 in, 2 out]
      n128 = Divide(x=w314, y=w312) -> (x/y=w309:dbl)
      n129 = Multiply(x=w309, y=w310) -> (x*y=w311:dbl)
      n130 = property on="X Velocity SP mm/sec" class="DigNum (strict)"("Val(Sgnl)"=w311) -> ()  [unwired: 2 in, 2 out]
      "X steps/rev" <- w313
      "X mm/rev" <- w310
    }
    frame #3 {
      w319 = -750000 ("lower limit")
      w318 = 750000 ("upper limit")
      n131 = property on="X Step SP" class="DigNum (strict)"("Minimum"=w319) -> ()  [unwired: 2 in, 2 out]
      n132 = property on="X Step SP" class="DigNum (strict)"("Maximum"=w318) -> ()  [unwired: 2 in, 2 out]
      "X offset mm" <- 0.0 ("offset")
      "X MAXPOS" <- w318
      "X MINPOS" <- w319
    }
    frame #4 {
      w328 = refnum<visa-resource-name> "COM13" ("COM PORT")
      w326 = u16 0 items=["None", "XON/XOFF", "RTS/CTS", "XON/XOFF & RTS/CTS", "DTR/DSR", "XON/XOFF & DTR/DSR"] ("flow control (0:none)")
      w325 = u16 10 items=["1.0"=10, "1.5"=15, "2.0"=20] ("stop bits (10: 1 bit)")
      # "Stop bits"
      n133 = call-poly "VISA Configure Serial Port"("VISA resource name"=w328, "timeout (10sec)"=u32 10000, "baud rate (9600)"=u32 9600, "data bits (8)"=u16 8, "parity (0:none)"=enum16{"None", "Odd", "Even", "Mark", "Space"}."None", "stop bits (10: 1 bit)"=w325, "flow control (0:none)"=w326) -> ("VISA resource name out"=w321:refnum<visa-resource-name>, "error out"=w320:errorcluster)  [unwired: 7 in]
      "X COM PORT" <- w328
    }
    frame #5 {
      n134 = property on="X Run Current" class="DigNum (strict)"() -> ("Value"=w333:i32)  [unwired: 2 in, 2 out]
      n135 = Divide(x=w333, y=100) -> (x/y=w330:dbl)
      n136 = Multiply(x=3.5 ("y"), y=w330) -> (x*y=w332:dbl)
      n137 = Number To Fractional String(number=w332) -> (F-format string=w334:string)  [unwired: 3 in]
      n138 = call "Applied Send Command.vi"("error in (no error)"=w337, "Extra"=w334, "Command"=T1."Change Current", "VISA resource name"=w338) -> ("error out"=w336:errorcluster, "VISA resource name out"=w335:refnum<visa-resource-name>)  [unwired: 3 in, 1 out]
    }
    frame #6 {
      # "VELOCITY"
      n139 = property on="X steps/rev" class="DigNum (strict)"() -> ("Value"=w344:u32)  [unwired: 2 in, 2 out]
      n140 = property on="X Velocity SP step/sec" class="DigNum (strict)"() -> ("Value"=w345:i32)  [unwired: 2 in, 2 out]
      n141 = Divide(x=w345, y=w344) -> (x/y=w343:dbl)
      n142 = Number To Fractional String(number=w343) -> (F-format string=w350:string)  [unwired: 3 in]
      n143 = call "Applied Send Command.vi"("error in (no error)"=w349, "Extra"=w350, "Command"=T1."Velocity Setting", "VISA resource name"=w348) -> ("error out"=w351:errorcluster, "VISA resource name out"=w358:refnum<visa-resource-name>)  [unwired: 3 in, 1 out]
      n144 = call "Time Delay30"("error in (no error)"=w351, "Delay Time (s)"=0.1) -> ("error out"=w356:errorcluster)  [unwired: 9 in]
      n145 = call "Applied Send Command.vi"("error in (no error)"=w356, "Extra"="", "Command"=T1."Velocity Setting", "VISA resource name"=w358) -> ("error out"=w341:errorcluster, "read buffer"=w354:string, "VISA resource name out"=w342:refnum<visa-resource-name>)  [unwired: 3 in]
      n146 = Fract/Exp String To Number(string=w354, offset=3) -> (number=w347:dbl)  [unwired: 2 in, 1 out]
      n147 = Multiply(x=w347, y=w344) -> (x*y=w346:dbl)
      n148 = property on="X velocity PV step/sec" class="DigNum (strict)"("Val(Sgnl)"=w346) -> ()  [unwired: 2 in, 2 out]
    }
    frame #7 {
      # "GET CURRENT POSITION"
      n149 = call "Applied Send Command.vi"("error in (no error)"=w363, "Extra"="", "Command"=T1."Immediate Position?", "VISA resource name"=w364) -> ("error out"=w361:errorcluster, "read buffer"=w367:string, "VISA resource name out"=w362:refnum<visa-resource-name>)  [unwired: 3 in]
      n150 = call "Time Delay13"("error in (no error)"=w361, "Delay Time (s)"=0.1) -> ("error out"=w360:errorcluster)  [unwired: 9 in]
      n151 = Hexadecimal String To Number(string=w367, offset=3) -> (number=w365:u32)  [unwired: 1 in, 1 out]
    }
    frame #8 {
      n152 = property on="X Step SP" class="DigNum (strict)"() -> ("Maximum"=w373:dbl)  [unwired: 2 in, 2 out]
      n153 = property on="X Step SP" class="DigNum (strict)"("Val(Sgnl)"=w370) -> ()  [unwired: 2 in, 2 out]
      n154 = property on="X Step SP" class="DigNum (strict)"() -> ("Minimum"=w372:dbl)  [unwired: 2 in, 2 out]
      n155 = In Range and Coerce(upper limit=w373, x=w370, lower limit=w372) -> (In Range?=w371:bool)  [unwired: 1 out]
      n156 = property on="X  in Range" class="Bool (strict)"("Val(Sgnl)"=w371) -> ()  [unwired: 2 in, 2 out]
    }
  }
  n157 = call-poly <vilib>:"Read From Spreadsheet File.vi"("file path (dialog if empty)"=path "S:/LV codes/SCL2/POS.TXT") -> ("first row"=w43:i64[])  [unwired: 6 in, 4 out]
  n158 = call-poly <vilib>:"Read From Spreadsheet File.vi"("file path (dialog if empty)"=path "S:/LV codes/SCL2/PRESET.TXT") -> ("all rows"=w31:string[][])  [unwired: 6 in, 4 out]
  n159 = Array To Cluster(array=w43) -> (cluster=w42:T3)
  n160 = Transpose 2D Array(2D array=w31) -> (transposed array=w32:string[][])
  n161 = Unbundle(w42) -> ("first row[0]"=w40:i64, "first row[1]"=w39:i64, "first row[2]"=w38:i64, "first row[3]"=w37:i64)  [unwired: 5 out]
  n162 = Delete From Array(array=w32, index (row)=0) -> (deleted portion=w33:string[], array with subset deleted=w35:string[][])  [unwired: 2 in]
  n163 = property on="Reset X Motor Steps" class="DigNum (strict)"("Val(Sgnl)"=w40) -> ()  [unwired: 2 in, 2 out]
  n164 = property on="Reset Y Motor Steps" class="DigNum (strict)"("Val(Sgnl)"=w39) -> ()  [unwired: 2 in, 2 out]
  n165 = property on="Reset Z Motor Steps" class="DigNum (strict)"("Val(Sgnl)"=w38) -> ()  [unwired: 2 in, 2 out]
  n166 = property on="Reset R Motor Steps" class="DigNum (strict)"("Val(Sgnl)"=w37) -> ()  [unwired: 2 in, 2 out]
  n167 = Transpose 2D Array(2D array=w35) -> (transposed array=w36:string[][])
  n168 = property on="Preset positions" class="Ring (strict)"("Strings []"=w33) -> ()  [unwired: 2 in, 2 out]
  n169 = Decimal String To Number(string=w36) -> (number=w34:i32[][])  [unwired: 2 in, 1 out]
  n170 = Initialize Array(w25, w25, 4 ("dimension size")) -> (w28:i32[][])
  n171 = Build Array (concatenate)(w28, w34) -> (→"Presets":i32[][])
  n172 = while {
    tunnel: w76 -> [w394]
    tunnel: w75 -> [w397]
    tunnel: [w398] -> w50
    tunnel: [w396] -> w51
    tunnel: w73 -> [w393]
    tunnel: w72 -> [w392]
    tunnel: [w391] -> w71
    tunnel: [w390] -> w70
    tunnel: w57 -> [w389]
    tunnel: w56 -> [w388]
    tunnel: [w387] -> w53
    tunnel: [w386] -> w52
    tunnel: w55 -> [w385]
    tunnel: w54 -> [w384]
    tunnel: [w383] -> w49
    tunnel: [w382] -> w48
    stop <- "stop" stop-if-true
    n173 = flat-sequence {
      frame #0 {
      }
      frame #1 {
      }
    }
    n174 = flat-sequence {
      frame #0 {
      }
      frame #1 {
      }
    }
    n175 = property on="Preset positions" class="Ring (strict)"() -> ("Strings []"=w378:string[])  [unwired: 2 in, 2 out]
    n176 = event shown="[3] \"Y Scan Length SP steps\", \"Y Scan Velocity SP steps/sec \", \"X Scan Velocity SP steps/sec \", \"X Scan Length SP steps\", \"Z Scan Velocity SP steps/sec\", \"Z Scan Length SP steps\", \"R Scan Velocity SP steps/sec\", \"R Scan Length SP steps\": Value Change" {
      selector: _ -> [_ _ _ _ _ _ _ _ _ _ _ _ _ _ _ _ _ _ _ _ _ _ _ _ _]
      dyn-events: _ -> [_ _ _ _ _ _ _ _ _ _ _ _ _ _ _ _ _ _ _ _ _ _ _ _ _]
      timeout: 200 -> [_ _ _ _ _ _ _ _ _ _ _ _ _ _ _ _ _ _ _ _ _ _ _ _ _]
      tunnel: w397 -> [w508 _ _ _ _ _ _ _ _ _ _ _ w1238 _ _ _ _ w1531 _ _ w1635 w1651 w1695 w1783 w1928]
      tunnel: [w507 _ _ _ _ _ _ _ _ _ _ _ w1244 _ _ _ _ w1529 _ _ w1635 w1649 w1697 w1777 w1926] -> w398
      tunnel: w394 -> [w450 _ _ _ _ _ _ _ _ _ _ _ w1239 _ _ _ _ w1530 _ _ w1636 w1652 w1696 w1784 w1929]
      tunnel: [w506 _ _ _ _ _ _ _ _ _ _ _ w1245 _ _ _ _ w1526 _ _ w1636 w1650 w1698 w1778 w1927] -> w396
      tunnel: w393 -> [w449 _ _ _ _ _ _ _ _ _ _ _ _ _ _ w1432 w1492 _ _ _ _ w1646 w1688 w1786 w1925]
      tunnel: w392 -> [w483 _ _ _ _ _ _ _ _ _ _ _ _ _ _ w1431 w1491 _ _ _ _ w1645 w1687 w1785 w1924]
      tunnel: [w482 _ _ _ _ _ _ _ _ _ _ _ _ _ _ w1430 w1490 _ _ _ _ w1648 w1686 w1772 w1923] -> w391
      tunnel: [w481 _ _ _ _ _ _ _ _ _ _ _ _ _ _ w1429 w1489 _ _ _ _ w1647 w1685 w1771 w1922] -> w390
      tunnel: w389 -> [w455 _ _ _ _ _ _ _ _ _ _ _ _ w1301 _ _ _ _ w1564 _ _ w1644 w1682 w1782 w1921]
      tunnel: w388 -> [w458 _ _ _ _ _ _ _ _ _ _ _ _ w1300 _ _ _ _ w1563 _ _ w1643 w1681 w1781 w1920]
      tunnel: [w457 _ _ _ _ _ _ _ _ _ _ _ _ w1298 _ _ _ _ w1561 _ _ w1642 w1680 w1776 w1917] -> w387
      tunnel: [w456 _ _ _ _ _ _ _ _ _ _ _ _ w1299 _ _ _ _ w1562 _ _ w1641 w1679 w1775 w1916] -> w386
      tunnel: w385 -> [w454 _ _ _ _ _ _ _ _ _ _ _ _ _ w1365 _ _ _ _ w1601 _ w1640 w1676 w1780 w1919]
      tunnel: w384 -> [w453 _ _ _ _ _ _ _ _ _ _ _ _ _ w1364 _ _ _ _ w1600 _ w1639 w1675 w1779 w1918]
      tunnel: [w452 _ _ _ _ _ _ _ _ _ _ _ _ _ w1362 _ _ _ _ w1599 _ w1638 w1674 w1774 w1915] -> w383
      tunnel: [w451 _ _ _ _ _ _ _ _ _ _ _ _ _ w1363 _ _ _ _ w1598 _ w1637 w1673 w1773 w1914] -> w382
      event Timeout {
        n177 = event-data() -> ()  [unwired: 1 in, 2 out]
        n178 = property on="X Step SP" class="DigNum (strict)"() -> ("Maximum"=w433:dbl)  [unwired: 2 in, 2 out]
        n179 = property on="Y Step SP" class="DigNum (strict)"() -> ("Maximum"=w438:dbl)  [unwired: 2 in, 2 out]
        n180 = flat-sequence {
          tunnel: [w617] -> w480
          tunnel: [w630] -> w479
          tunnel: [w640] -> w478
          tunnel: [w610] -> w477
          tunnel: w455 -> [w625]
          tunnel: w458 -> [w626]
          tunnel: w480 -> [w650]
          tunnel: [w650] -> w476
          tunnel: w479 -> [w649]
          tunnel: [w649] -> w475
          tunnel: w478 -> [w648]
          tunnel: [w648] -> w474
          tunnel: w477 -> [w645]
          tunnel: [w645] -> w473
          tunnel: w476 -> [w657]
          tunnel: [w658] -> w472
          tunnel: w475 -> [w660]
          tunnel: [w659] -> w471
          tunnel: w474 -> [w656]
          tunnel: [w655] -> w470
          tunnel: w473 -> [w655]
          tunnel: w472 -> [w670]
          tunnel: w471 -> [w671]
          tunnel: w470 -> [w673]
          tunnel: [w669] -> w456
          tunnel: [w668] -> w457
          frame #0 {
            w629 = 0.2 ("Delay Time (s)")
            n181 = property on="Z Step SP" class="DigNum (strict)"() -> ("Maximum"=w642:dbl)  [unwired: 2 in, 2 out]
            n182 = property on="Z Step SP" class="DigNum (strict)"() -> ("Minimum"=w644:dbl)  [unwired: 2 in, 2 out]
            n183 = property on="Z steps/rev" class="DigNum (strict)"() -> ("Value"=w638:u32)  [unwired: 2 in, 2 out]
            n184 = property on="Z offset mm" class="DigNum (strict)"() -> ("Value"=w634:dbl)  [unwired: 2 in, 2 out]
            n185 = To Long Integer(number=w642) -> (32bit integer=w641:i32)
            n186 = To Long Integer(number=w644) -> (32bit integer=w643:i32)
            n187 = To Double Precision Float(number=w638) -> (double precision float=w639:dbl)
            n188 = call "Applied Send Command.vi"("error in (no error)"=w626, "Command"=T1."Immediate Position?", "VISA resource name"=w625) -> ("error out"=w624:errorcluster, "read buffer"=w621:string, "VISA resource name out"=w619:refnum<visa-resource-name>)  [unwired: 4 in]
            n189 = call "Time Delay17"("error in (no error)"=w624, "Delay Time (s)"=w629) -> ("error out"=w609:errorcluster)  [unwired: 9 in]
            n190 = Hexadecimal String To Number(string=w621, offset=3) -> (number=w622:u32)  [unwired: 1 in, 1 out]
            n191 = To Long Integer(number=w622) -> (32bit integer=w632:i32)
            n192 = call "Applied Send Command.vi"("error in (no error)"=w609, "Command"=T1."Request Status", "VISA resource name"=w619) -> ("error out"=w618:errorcluster, "read buffer"=w614:string, "VISA resource name out"=w617:refnum<visa-resource-name>)  [unwired: 4 in]
            n193 = property on="Z Step PV" class="DigNum (strict)"("Val(Sgnl)"=w632) -> ()  [unwired: 2 in, 2 out]
            n194 = call "Time Delay16"("error in (no error)"=w618, "Delay Time (s)"=w629) -> ("error out"=w630:errorcluster)  [unwired: 9 in]
            n195 = String Subset(string=w614, offset (0)=0, length (rest)=1 ("length (rest)")) -> (substring=w611:string)
            n196 = In Range and Coerce(upper limit=w641, x=w632, lower limit=w643) -> (In Range?=w640:bool)  [unwired: 1 out]
            n197 = To Double Precision Float(number=w632) -> (double precision float=w633:dbl)
            n198 = Not Equal?(x=w611, y="R") -> (x != y?=w610:bool)
            n199 = Equal?(x=w611, y="R") -> (x = y?=w628:bool)
            n200 = property on="Z in Motion" class="Bool (strict)"("Val(Sgnl)"=w610) -> ()  [unwired: 2 in, 2 out]
            n201 = property on="Z in Range" class="Bool (strict)"("Val(Sgnl)"=w640) -> ()  [unwired: 2 in, 2 out]
            n202 = property on="Z Ready" class="Bool (strict)"("Val(Sgnl)"=w628) -> ()  [unwired: 2 in, 2 out]
            n203 = Divide(x=w633, y=w639) -> (x/y=w637:dbl)
            n204 = property on="Z mm/rev" class="DigNum (strict)"() -> ("Value"=w636:dbl)  [unwired: 2 in, 2 out]
            n205 = Multiply(x=w637, y=w636) -> (x*y=w635:dbl)
            n206 = Add(x=w635, y=w634) -> (x+y=w631:dbl)
            n207 = property on="Z Position mm PV" class="DigNum (strict)"("Val(Sgnl)"=w631) -> ()  [unwired: 2 in, 2 out]
          }
          frame #1 {
            n208 = property on="Z Scan" class="Bool (strict)"() -> ("Value"=w646:bool)  [unwired: 2 in, 2 out]
            n209 = Or(x=w645, y=w646) -> (x .or. y?=w647:bool)
            n210 = case shown="True" w647 {
              frame False {
                n211 = property on="Z Scan OK" class="Bool"("DisabledEnum"=T2."Enabled" ("Disabled")) -> ()  [unwired: 2 in, 2 out]
                n212 = property on="Z Go" class="Bool"("DisabledEnum"=T2."Enabled" ("Disabled")) -> ()  [unwired: 2 in, 2 out]
              }
              frame True {
                n213 = property on="Z Scan OK" class="Bool"("DisabledEnum"=T2."Disabled and Grayed Out" ("Disabled")) -> ()  [unwired: 2 in, 2 out]
                n214 = property on="Z Go" class="Bool"("DisabledEnum"=T2."Disabled and Grayed Out" ("Disabled")) -> ()  [unwired: 2 in, 2 out]
              }
            }
          }
          frame #2 {
            n215 = case shown="False" w656 {
              tunnel: w657 -> [w664 w667]
              tunnel: [w662 w667] -> w658
              tunnel: [w661 w666] -> w659
              tunnel: w660 -> [w663 w666]
              frame False {
                n216 = call "Applied Send Command.vi"("error in (no error)"=w663, "Command"=T1."Stop & Kill Buffer", "VISA resource name"=w664) -> ("error out"=w661:errorcluster, "VISA resource name out"=w662:refnum<visa-resource-name>)  [unwired: 4 in, 1 out]
              }
              frame True {
              }
            }
          }
          frame #3 {
            n217 = property on="Z Backlash corr" class="Bool (strict)"() -> ("Value"=w674:bool)  [unwired: 2 in, 2 out]
            n218 = Implies(1:w673, 2:w674) -> (0:w672:bool)
            n219 = case shown="False" w672 {
              tunnel: w671 -> [w675 w707]
              tunnel: w670 -> [w676 w708]
              tunnel: [w677 w707] -> w669
              tunnel: [w678 w708] -> w668
              frame False {
                w704 = 0.1 ("Delay Time (s)")
                # "Backlash"
                # "Backlash"
                n220 = property on="Z Backlash" class="DigNum (strict)"() -> ("Value"=w682:i32)  [unwired: 2 in, 2 out]
                n221 = To Long Integer(number=w682) -> (32bit integer=w685:i32)
                n222 = property on="Z Backlash corr" class="Bool (strict)"("Val(Sgnl)"=FALSE ("Value (Signaling)")) -> ()  [unwired: 2 in, 2 out]
                n223 = Number To Decimal String(number=w682) -> (decimal integer string=w690:string)  [unwired: 1 in]
                n224 = Negate(x=w685) -> (-x=w684:i32)
                n225 = property on="Z Backlash steps/sec" class="DigNum (strict)"() -> ("Value"=w681:i32)  [unwired: 2 in, 2 out]
                n226 = Number To Decimal String(number=w684) -> (decimal integer string=w691:string)  [unwired: 1 in]
                n227 = property on="Z steps/rev" class="DigNum (strict)"() -> ("Value"=w680:u32)  [unwired: 2 in, 2 out]
                n228 = Divide(x=w681, y=w680) -> (x/y=w705:dbl)
                n229 = Number To Fractional String(number=w705) -> (F-format string=w706:string)  [unwired: 3 in]
                n230 = call "Applied Send Command.vi"("error in (no error)"=w675, "Extra"=w706, "Command"=T1."Velocity Setting", "VISA resource name"=w676) -> ("error out"=w702:errorcluster, "VISA resource name out"=w695:refnum<visa-resource-name>)  [unwired: 3 in, 1 out]
                n231 = call "Time Delay47"("error in (no error)"=w702, "Delay Time (s)"=w704) -> ("error out"=w703:errorcluster)  [unwired: 9 in]
                n232 = call "Applied Send Command.vi"("error in (no error)"=w703, "Extra"=w690, "Command"=T1."Distance or Position", "VISA resource name"=w695) -> ("error out"=w696:errorcluster, "VISA resource name out"=w689:refnum<visa-resource-name>)  [unwired: 3 in, 1 out]
                n233 = call "Time Delay44"("error in (no error)"=w696, "Delay Time (s)"=w704) -> ("error out"=w697:errorcluster)  [unwired: 9 in]
                n234 = call "Applied Send Command.vi"("error in (no error)"=w697, "Command"=T1."Feed to Length", "VISA resource name"=w689) -> ("error out"=w698:errorcluster, "VISA resource name out"=w692:refnum<visa-resource-name>)  [unwired: 4 in, 1 out]
                n235 = call "Time Delay45"("error in (no error)"=w698, "Delay Time (s)"=w704) -> ("error out"=w699:errorcluster)  [unwired: 9 in]
                n236 = call "Applied Send Command.vi"("error in (no error)"=w699, "Extra"=w691, "Command"=T1."Distance or Position", "VISA resource name"=w692) -> ("error out"=w700:errorcluster, "VISA resource name out"=w693:refnum<visa-resource-name>)  [unwired: 3 in, 1 out]
                n237 = call "Time Delay46"("error in (no error)"=w700, "Delay Time (s)"=w704) -> ("error out"=w701:errorcluster)  [unwired: 9 in]
                n238 = call "Applied Send Command.vi"("error in (no error)"=w701, "Command"=T1."Feed to Length", "VISA resource name"=w693) -> ("error out"=w677:errorcluster, "VISA resource name out"=w678:refnum<visa-resource-name>)  [unwired: 4 in, 1 out]
              }
              frame True {
              }
            }
          }
        }
        n239 = flat-sequence {
          tunnel: [w518] -> w469
          tunnel: [w530] -> w468
          tunnel: [w540] -> w467
          tunnel: [w509] -> w466
          tunnel: w454 -> [w527]
          tunnel: w453 -> [w526]
          tunnel: w469 -> [w550]
          tunnel: [w550] -> w465
          tunnel: w468 -> [w549]
          tunnel: [w549] -> w464
          tunnel: w467 -> [w548]
          tunnel: [w548] -> w463
          tunnel: w466 -> [w545]
          tunnel: [w545] -> w462
          tunnel: w465 -> [w557]
          tunnel: [w558] -> w461
          tunnel: w464 -> [w560]
          tunnel: [w559] -> w460
          tunnel: w463 -> [w556]
          tunnel: [w555] -> w459
          tunnel: w462 -> [w555]
          tunnel: w461 -> [w570]
          tunnel: w460 -> [w571]
          tunnel: w459 -> [w573]
          tunnel: [w569] -> w451
          tunnel: [w568] -> w452
          frame #0 {
            w529 = 0.2 ("Delay Time (s)")
            n240 = property on="R Step SP" class="DigNum (strict)"() -> ("Maximum"=w542:dbl)  [unwired: 2 in, 2 out]
            n241 = property on="R Step SP" class="DigNum (strict)"() -> ("Minimum"=w544:dbl)  [unwired: 2 in, 2 out]
            n242 = property on="R steps/rev" class="DigNum (strict)"() -> ("Value"=w538:u32)  [unwired: 2 in, 2 out]
            n243 = property on="R offset deg" class="DigNum (strict)"() -> ("Value"=w534:dbl)  [unwired: 2 in, 2 out]
            n244 = To Long Integer(number=w542) -> (32bit integer=w541:i32)
            n245 = To Long Integer(number=w544) -> (32bit integer=w543:i32)
            n246 = To Double Precision Float(number=w538) -> (double precision float=w539:dbl)
            n247 = call "Applied Send Command.vi"("error in (no error)"=w526, "Command"=T1."Immediate Position?", "VISA resource name"=w527) -> ("error out"=w522:errorcluster, "read buffer"=w523:string, "VISA resource name out"=w520:refnum<visa-resource-name>)  [unwired: 4 in]
            n248 = call "Time Delay21"("error in (no error)"=w522, "Delay Time (s)"=w529) -> ("error out"=w519:errorcluster)  [unwired: 9 in]
            n249 = Hexadecimal String To Number(string=w523, offset=3) -> (number=w524:u32)  [unwired: 1 in, 1 out]
            n250 = To Long Integer(number=w524) -> (32bit integer=w532:i32)
            n251 = call "Applied Send Command.vi"("error in (no error)"=w519, "Command"=T1."Request Status", "VISA resource name"=w520) -> ("error out"=w517:errorcluster, "read buffer"=w514:string, "VISA resource name out"=w518:refnum<visa-resource-name>)  [unwired: 4 in]
            n252 = property on="R Step PV" class="DigNum (strict)"("Val(Sgnl)"=w532) -> ()  [unwired: 2 in, 2 out]
            n253 = call "Time Delay20"("error in (no error)"=w517, "Delay Time (s)"=w529) -> ("error out"=w530:errorcluster)  [unwired: 9 in]
            n254 = String Subset(string=w514, offset (0)=0, length (rest)=1 ("length (rest)")) -> (substring=w510:string)
            n255 = In Range and Coerce(upper limit=w541, x=w532, lower limit=w543) -> (In Range?=w540:bool)  [unwired: 1 out]
            n256 = To Double Precision Float(number=w532) -> (double precision float=w533:dbl)
            n257 = Not Equal?(x=w510, y="R") -> (x != y?=w509:bool)
            n258 = Equal?(x=w510, y="R") -> (x = y?=w511:bool)
            n259 = property on="R in Motion" class="Bool (strict)"("Val(Sgnl)"=w509) -> ()  [unwired: 2 in, 2 out]
            n260 = property on="R in Range" class="Bool (strict)"("Val(Sgnl)"=w540) -> ()  [unwired: 2 in, 2 out]
            n261 = property on="R Ready" class="Bool (strict)"("Val(Sgnl)"=w511) -> ()  [unwired: 2 in, 2 out]
            n262 = Divide(x=w533, y=w539) -> (x/y=w537:dbl)
            n263 = property on="R deg/rev" class="DigNum (strict)"() -> ("Value"=w536:dbl)  [unwired: 2 in, 2 out]
            n264 = Multiply(x=w537, y=w536) -> (x*y=w535:dbl)
            n265 = Add(x=w535, y=w534) -> (x+y=w531:dbl)
            n266 = property on="R Position deg PV" class="DigNum (strict)"("Val(Sgnl)"=w531) -> ()  [unwired: 2 in, 2 out]
          }
          frame #1 {
            n267 = property on="R Scan" class="Bool (strict)"() -> ("Value"=w546:bool)  [unwired: 2 in, 2 out]
            n268 = Or(x=w545, y=w546) -> (x .or. y?=w547:bool)
            n269 = case shown="True" w547 {
              frame False {
                n270 = property on="R Scan OK" class="Bool"("DisabledEnum"=T2."Enabled" ("Disabled")) -> ()  [unwired: 2 in, 2 out]
                n271 = property on="R Go" class="Bool"("DisabledEnum"=T2."Enabled" ("Disabled")) -> ()  [unwired: 2 in, 2 out]
              }
              frame True {
                n272 = property on="R Scan OK" class="Bool"("DisabledEnum"=T2."Disabled and Grayed Out" ("Disabled")) -> ()  [unwired: 2 in, 2 out]
                n273 = property on="R Go" class="Bool"("DisabledEnum"=T2."Disabled and Grayed Out" ("Disabled")) -> ()  [unwired: 2 in, 2 out]
              }
            }
          }
          frame #2 {
            n274 = case shown="False" w556 {
              tunnel: w557 -> [w564 w567]
              tunnel: [w562 w567] -> w558
              tunnel: [w561 w566] -> w559
              tunnel: w560 -> [w563 w566]
              frame False {
                n275 = call "Applied Send Command.vi"("error in (no error)"=w563, "Command"=T1."Stop & Kill Buffer", "VISA resource name"=w564) -> ("error out"=w561:errorcluster, "VISA resource name out"=w562:refnum<visa-resource-name>)  [unwired: 4 in, 1 out]
              }
              frame True {
              }
            }
          }
          frame #3 {
            n276 = property on="R Backlash corr" class="Bool (strict)"() -> ("Value"=w574:bool)  [unwired: 2 in, 2 out]
            n277 = Implies(1:w573, 2:w574) -> (0:w572:bool)
            n278 = case shown="False" w572 {
              tunnel: w571 -> [w578 w607]
              tunnel: w570 -> [w577 w608]
              tunnel: [w575 w607] -> w569
              tunnel: [w576 w608] -> w568
              frame False {
                w585 = 0.1 ("Delay Time (s)")
                # "Backlash"
                # "Backlash"
                n279 = property on="R Backlash" class="DigNum (strict)"() -> ("Value"=w579:i32)  [unwired: 2 in, 2 out]
                n280 = To Long Integer(number=w579) -> (32bit integer=w604:i32)
                n281 = property on="R Backlash corr" class="Bool (strict)"("Val(Sgnl)"=FALSE ("Value (Signaling)")) -> ()  [unwired: 2 in, 2 out]
                n282 = Number To Decimal String(number=w579) -> (decimal integer string=w599:string)  [unwired: 1 in]
                n283 = Negate(x=w604) -> (-x=w605:i32)
                n284 = property on="R Backlash steps/sec" class="DigNum (strict)"() -> ("Value"=w582:i32)  [unwired: 2 in, 2 out]
                n285 = Number To Decimal String(number=w605) -> (decimal integer string=w598:string)  [unwired: 1 in]
                n286 = property on="R steps/rev" class="DigNum (strict)"() -> ("Value"=w580:u32)  [unwired: 2 in, 2 out]
                n287 = Divide(x=w582, y=w580) -> (x/y=w581:dbl)
                n288 = Number To Fractional String(number=w581) -> (F-format string=w584:string)  [unwired: 3 in]
                n289 = call "Applied Send Command.vi"("error in (no error)"=w578, "Extra"=w584, "Command"=T1."Velocity Setting", "VISA resource name"=w577) -> ("error out"=w587:errorcluster, "VISA resource name out"=w594:refnum<visa-resource-name>)  [unwired: 3 in, 1 out]
                n290 = call "Time Delay49"("error in (no error)"=w587, "Delay Time (s)"=w585) -> ("error out"=w586:errorcluster)  [unwired: 9 in]
                n291 = call "Applied Send Command.vi"("error in (no error)"=w586, "Extra"=w599, "Command"=T1."Distance or Position", "VISA resource name"=w594) -> ("error out"=w593:errorcluster, "VISA resource name out"=w600:refnum<visa-resource-name>)  [unwired: 3 in, 1 out]
                n292 = call "Time Delay18"("error in (no error)"=w593, "Delay Time (s)"=w585) -> ("error out"=w592:errorcluster)  [unwired: 9 in]
                n293 = call "Applied Send Command.vi"("error in (no error)"=w592, "Command"=T1."Feed to Length", "VISA resource name"=w600) -> ("error out"=w591:errorcluster, "VISA resource name out"=w597:refnum<visa-resource-name>)  [unwired: 4 in, 1 out]
                n294 = call "Time Delay19"("error in (no error)"=w591, "Delay Time (s)"=w585) -> ("error out"=w590:errorcluster)  [unwired: 9 in]
                n295 = call "Applied Send Command.vi"("error in (no error)"=w590, "Extra"=w598, "Command"=T1."Distance or Position", "VISA resource name"=w597) -> ("error out"=w589:errorcluster, "VISA resource name out"=w596:refnum<visa-resource-name>)  [unwired: 3 in, 1 out]
                n296 = call "Time Delay48"("error in (no error)"=w589, "Delay Time (s)"=w585) -> ("error out"=w588:errorcluster)  [unwired: 9 in]
                n297 = call "Applied Send Command.vi"("error in (no error)"=w588, "Command"=T1."Feed to Length", "VISA resource name"=w596) -> ("error out"=w575:errorcluster, "VISA resource name out"=w576:refnum<visa-resource-name>)  [unwired: 4 in, 1 out]
              }
              frame True {
              }
            }
          }
        }
        n298 = property on="X Step SP" class="DigNum (strict)"() -> ("Minimum"=w434:dbl)  [unwired: 2 in, 2 out]
        n299 = property on="Y Step SP" class="DigNum (strict)"() -> ("Minimum"=w437:dbl)  [unwired: 2 in, 2 out]
        n300 = property on="X Step PV" class="DigNum (strict)"() -> ("Value"=w432:i32)  [unwired: 2 in, 2 out]
        n301 = property on="Y Step PV" class="DigNum (strict)"() -> ("Value"=w431:i32)  [unwired: 2 in, 2 out]
        n302 = Subtract(x=w433, y=w434) -> (x-y=w435:dbl)
        n303 = Absolute Value(x=w432) -> (abs(x)=w429:i32)
        n304 = Absolute Value(x=w431) -> (abs(x)=w430:i32)
        n305 = Subtract(x=w438, y=w437) -> (x-y=w439:dbl)
        n306 = property on="Y Scan Length SP steps" class="DigNum (strict)"() -> ("Value"=w441:i32)  [unwired: 2 in, 2 out]
        n307 = property on="Z Scan Length SP steps" class="DigNum (strict)"() -> ("Value"=w442:i32)  [unwired: 2 in, 2 out]
        n308 = Multiply(x=w429, y=w430) -> (x*y=w424:i32)
        n309 = Divide(x=w439, y=2.0) -> (x/y=w427:dbl)
        n310 = Divide(x=w435, y=2.0) -> (x/y=w428:dbl)
        n311 = Absolute Value(x=w427) -> (abs(x)=w425:dbl)
        n312 = Absolute Value(x=w428) -> (abs(x)=w426:dbl)
        n313 = Divide(x=w441, y=w442) -> (x/y=w443:dbl)
        n314 = Multiply(x=w425, y=w426) -> (x*y=w423:dbl)
        n315 = Inverse Tangent(1:w443) -> (0:w444:dbl)
        n316 = Less Or Equal?(x=w424, y=w423) -> (x <= y?=w422:bool)
        n317 = Divide(x=w444, y=6.283185307179586) -> (x/y=w445:dbl)
        n318 = flat-sequence {
          tunnel: [w721] -> w494
          tunnel: [w732] -> w493
          tunnel: [w710] -> w492
          tunnel: [w717] -> w491
          tunnel: w449 -> [w728]
          tunnel: w483 -> [w716]
          tunnel: w433 -> [w712]
          tunnel: w434 -> [w711]
          tunnel: w422 -> [w709]
          tunnel: w494 -> [w752]
          tunnel: [w752] -> w490
          tunnel: w493 -> [w751]
          tunnel: [w751] -> w489
          tunnel: w492 -> [w750]
          tunnel: [w750] -> w488
          tunnel: w491 -> [w747]
          tunnel: [w747] -> w487
          tunnel: w490 -> [w761]
          tunnel: [w758] -> w486
          tunnel: w489 -> [w760]
          tunnel: [w759] -> w485
          tunnel: w488 -> [w757]
          tunnel: [w762] -> w484
          tunnel: w487 -> [w762]
          tunnel: w486 -> [w773]
          tunnel: w485 -> [w774]
          tunnel: w484 -> [w775]
          tunnel: [w772] -> w481
          tunnel: [w771] -> w482
          frame #0 {
            w731 = 0.2 ("Delay Time (s)")
            n319 = To Long Integer(number=w712) -> (32bit integer=w744:i32)
            n320 = To Long Integer(number=w711) -> (32bit integer=w745:i32)
            n321 = property on="X steps/rev" class="DigNum (strict)"() -> ("Value"=w741:u32)  [unwired: 2 in, 2 out]
            n322 = property on="X offset mm" class="DigNum (strict)"() -> ("Value"=w737:dbl)  [unwired: 2 in, 2 out]
            n323 = To Double Precision Float(number=w741) -> (double precision float=w742:dbl)
            n324 = call "Applied Send Command.vi"("error in (no error)"=w716, "Command"=T1."Immediate Position?", "VISA resource name"=w728) -> ("error out"=w726:errorcluster, "read buffer"=w727:string, "VISA resource name out"=w722:refnum<visa-resource-name>)  [unwired: 4 in]
            n325 = call "Time Delay12"("error in (no error)"=w726, "Delay Time (s)"=w731) -> ("error out"=w719:errorcluster)  [unwired: 9 in]
            n326 = Hexadecimal String To Number(string=w727, offset=3) -> (number=w733:u32)  [unwired: 1 in, 1 out]
            n327 = To Long Integer(number=w733) -> (32bit integer=w735:i32)
            n328 = call "Applied Send Command.vi"("error in (no error)"=w719, "Command"=T1."Request Status", "VISA resource name"=w722) -> ("error out"=w720:errorcluster, "read buffer"=w724:string, "VISA resource name out"=w721:refnum<visa-resource-name>)  [unwired: 4 in]
            n329 = property on="X Step PV" class="DigNum (strict)"("Val(Sgnl)"=w735) -> ()  [unwired: 2 in, 2 out]
            n330 = call "Time Delay11"("error in (no error)"=w720, "Delay Time (s)"=w731) -> ("error out"=w732:errorcluster)  [unwired: 9 in]
            n331 = String Subset(string=w724, offset (0)=0, length (rest)=1 ("length (rest)")) -> (substring=w713:string)
            n332 = In Range and Coerce(upper limit=w744, x=w735, lower limit=w745) -> (In Range?=w743:bool)  [unwired: 1 out]
            n333 = To Double Precision Float(number=w735) -> (double precision float=w736:dbl)
            n334 = Not Equal?(x=w713, y="R") -> (x != y?=w717:bool)
            n335 = Equal?(x=w713, y="R") -> (x = y?=w730:bool)
            n336 = property on="X  in Motion" class="Bool (strict)"("Val(Sgnl)"=w717) -> ()  [unwired: 2 in, 2 out]
            n337 = property on="X Ready" class="Bool (strict)"("Val(Sgnl)"=w730) -> ()  [unwired: 2 in, 2 out]
            n338 = Divide(x=w736, y=w742) -> (x/y=w740:dbl)
            n339 = And(x=w709, y=w743) -> (x .and. y?=w710:bool)
            n340 = property on="X  in Range" class="Bool (strict)"("Val(Sgnl)"=w710) -> ()  [unwired: 2 in, 2 out]
            n341 = property on="X mm/rev" class="DigNum (strict)"() -> ("Value"=w739:dbl)  [unwired: 2 in, 2 out]
            n342 = Multiply(x=w740, y=w739) -> (x*y=w738:dbl)
            n343 = Add(x=w738, y=w737) -> (x+y=w734:dbl)
            n344 = property on="X Position mm PV" class="DigNum (strict)"("Val(Sgnl)"=w734) -> ()  [unwired: 2 in, 2 out]
          }
          frame #1 {
            n345 = property on="X Scan" class="Bool (strict)"() -> ("Value"=w748:bool)  [unwired: 2 in, 2 out]
            n346 = Or(x=w747, y=w748) -> (x .or. y?=w749:bool)
            n347 = case shown="True" w749 {
              frame False {
                n348 = property on="X Scan OK" class="Bool"("DisabledEnum"=T2."Enabled" ("Disabled")) -> ()  [unwired: 2 in, 2 out]
                n349 = property on="X Go" class="Bool"("DisabledEnum"=T2."Enabled" ("Disabled")) -> ()  [unwired: 2 in, 2 out]
              }
              frame True {
                n350 = property on="X Scan OK" class="Bool"("DisabledEnum"=T2."Disabled and Grayed Out" ("Disabled")) -> ()  [unwired: 2 in, 2 out]
                n351 = property on="X Go" class="Bool"("DisabledEnum"=T2."Disabled and Grayed Out" ("Disabled")) -> ()  [unwired: 2 in, 2 out]
              }
            }
          }
          frame #2 {
            n352 = case shown="False" w757 {
              tunnel: w761 -> [w764 w769]
              tunnel: [w766 w769] -> w758
              tunnel: [w767 w768] -> w759
              tunnel: w760 -> [w763 w768]
              frame False {
                n353 = call "Applied Send Command.vi"("error in (no error)"=w763, "Command"=T1."Stop & Kill Buffer", "VISA resource name"=w764) -> ("error out"=w767:errorcluster, "VISA resource name out"=w766:refnum<visa-resource-name>)  [unwired: 4 in, 1 out]
              }
              frame True {
              }
            }
          }
          frame #3 {
            n354 = property on="X Backlash corr" class="Bool (strict)"() -> ("Value"=w776:bool)  [unwired: 2 in, 2 out]
            n355 = Implies(1:w775, 2:w776) -> (0:w770:bool)
            n356 = case shown="False" w770 {
              tunnel: w774 -> [w790 w809]
              tunnel: w773 -> [w791 w810]
              tunnel: [w793 w809] -> w772
              tunnel: [w792 w810] -> w771
              frame False {
                w781 = 0.1 ("Delay Time (s)")
                # "Backlash"
                n357 = property on="X Backlash" class="DigNum (strict)"() -> ("Value"=w796:i32)  [unwired: 2 in, 2 out]
                n358 = To Long Integer(number=w796) -> (32bit integer=w805:i32)
                n359 = property on="X Backlash corr" class="Bool (strict)"("Val(Sgnl)"=FALSE ("Value (Signaling)")) -> ()  [unwired: 2 in, 2 out]
                n360 = Number To Decimal String(number=w796) -> (decimal integer string=w800:string)  [unwired: 1 in]
                n361 = Negate(x=w805) -> (-x=w806:i32)
                n362 = property on="X Backlash steps/sec" class="DigNum (strict)"() -> ("Value"=w780:i32)  [unwired: 2 in, 2 out]
                n363 = Number To Decimal String(number=w806) -> (decimal integer string=w799:string)  [unwired: 1 in]
                n364 = property on="X steps/rev" class="DigNum (strict)"() -> ("Value"=w779:u32)  [unwired: 2 in, 2 out]
                n365 = Divide(x=w780, y=w779) -> (x/y=w778:dbl)
                n366 = Number To Fractional String(number=w778) -> (F-format string=w777:string)  [unwired: 3 in]
                n367 = call "Applied Send Command.vi"("error in (no error)"=w790, "Extra"=w777, "Command"=T1."Velocity Setting", "VISA resource name"=w791) -> ("error out"=w783:errorcluster, "VISA resource name out"=w794:refnum<visa-resource-name>)  [unwired: 3 in, 1 out]
                n368 = call "Time Delay35"("error in (no error)"=w783, "Delay Time (s)"=w781) -> ("error out"=w782:errorcluster)  [unwired: 9 in]
                n369 = call "Applied Send Command.vi"("error in (no error)"=w782, "Extra"=w800, "Command"=T1."Distance or Position", "VISA resource name"=w794) -> ("error out"=w789:errorcluster, "VISA resource name out"=w801:refnum<visa-resource-name>)  [unwired: 3 in, 1 out]
                n370 = call "Time Delay32"("error in (no error)"=w789, "Delay Time (s)"=w781) -> ("error out"=w788:errorcluster)  [unwired: 9 in]
                n371 = call "Applied Send Command.vi"("error in (no error)"=w788, "Command"=T1."Feed to Length", "VISA resource name"=w801) -> ("error out"=w787:errorcluster, "VISA resource name out"=w798:refnum<visa-resource-name>)  [unwired: 4 in, 1 out]
                n372 = call "Time Delay33"("error in (no error)"=w787, "Delay Time (s)"=w781) -> ("error out"=w786:errorcluster)  [unwired: 9 in]
                n373 = call "Applied Send Command.vi"("error in (no error)"=w786, "Extra"=w799, "Command"=T1."Distance or Position", "VISA resource name"=w798) -> ("error out"=w785:errorcluster, "VISA resource name out"=w797:refnum<visa-resource-name>)  [unwired: 3 in, 1 out]
                n374 = call "Time Delay34"("error in (no error)"=w785, "Delay Time (s)"=w781) -> ("error out"=w784:errorcluster)  [unwired: 9 in]
                n375 = call "Applied Send Command.vi"("error in (no error)"=w784, "Command"=T1."Feed to Length", "VISA resource name"=w797) -> ("error out"=w793:errorcluster, "VISA resource name out"=w792:refnum<visa-resource-name>)  [unwired: 4 in, 1 out]
              }
              frame True {
              }
            }
          }
        }
        n376 = flat-sequence {
          tunnel: w508 -> [w827]
          tunnel: w450 -> [w828]
          tunnel: [w824] -> w505
          tunnel: [w834] -> w503
          tunnel: [w813] -> w501
          tunnel: [w815] -> w499
          tunnel: w438 -> [w814]
          tunnel: w437 -> [w811]
          tunnel: w422 -> [w812]
          tunnel: w505 -> [w854]
          tunnel: [w854] -> w504
          tunnel: w503 -> [w853]
          tunnel: [w853] -> w502
          tunnel: w501 -> [w852]
          tunnel: [w852] -> w500
          tunnel: w499 -> [w849]
          tunnel: [w849] -> w495
          tunnel: w504 -> [w861]
          tunnel: [w862] -> w498
          tunnel: w502 -> [w864]
          tunnel: [w863] -> w497
          tunnel: w500 -> [w860]
          tunnel: [w859] -> w496
          tunnel: w495 -> [w859]
          tunnel: w498 -> [w874]
          tunnel: w497 -> [w875]
          tunnel: w496 -> [w877]
          tunnel: [w873] -> w507
          tunnel: [w872] -> w506
          frame #0 {
            w833 = 0.2 ("Delay Time (s)")
            n377 = To Long Integer(number=w814) -> (32bit integer=w846:i32)
            n378 = To Long Integer(number=w811) -> (32bit integer=w847:i32)
            n379 = property on="Y steps/rev" class="DigNum (strict)"() -> ("Value"=w843:u32)  [unwired: 2 in, 2 out]
            n380 = property on="Y offset mm" class="DigNum (strict)"() -> ("Value"=w839:dbl)  [unwired: 2 in, 2 out]
            n381 = To Double Precision Float(number=w843) -> (double precision float=w844:dbl)
            n382 = call "Applied Send Command.vi"("error in (no error)"=w827, "Command"=T1."Immediate Position?", "VISA resource name"=w828) -> ("error out"=w830:errorcluster, "read buffer"=w831:string, "VISA resource name out"=w825:refnum<visa-resource-name>)  [unwired: 4 in]
            n383 = call "Time Delay4"("error in (no error)"=w830, "Delay Time (s)"=w833) -> ("error out"=w823:errorcluster)  [unwired: 9 in]
            n384 = Hexadecimal String To Number(string=w831, offset=3) -> (number=w835:u32)  [unwired: 1 in, 1 out]
            n385 = To Long Integer(number=w835) -> (32bit integer=w837:i32)
            n386 = call "Applied Send Command.vi"("error in (no error)"=w823, "Command"=T1."Request Status", "VISA resource name"=w825) -> ("error out"=w822:errorcluster, "read buffer"=w819:string, "VISA resource name out"=w824:refnum<visa-resource-name>)  [unwired: 4 in]
            n387 = property on="Y Step PV" class="DigNum (strict)"("Val(Sgnl)"=w837) -> ()  [unwired: 2 in, 2 out]
            n388 = call "Time Delay3"("error in (no error)"=w822, "Delay Time (s)"=w833) -> ("error out"=w834:errorcluster)  [unwired: 9 in]
            n389 = String Subset(string=w819, offset (0)=0, length (rest)=1 ("length (rest)")) -> (substring=w817:string)
            n390 = In Range and Coerce(upper limit=w846, x=w837, lower limit=w847) -> (In Range?=w845:bool)  [unwired: 1 out]
            n391 = To Double Precision Float(number=w837) -> (double precision float=w838:dbl)
            n392 = Not Equal?(x=w817, y="R") -> (x != y?=w815:bool)
            n393 = Equal?(x=w817, y="R") -> (x = y?=w832:bool)
            n394 = property on="Y in Motion" class="Bool (strict)"("Val(Sgnl)"=w815) -> ()  [unwired: 2 in, 2 out]
            n395 = property on="Y Ready" class="Bool (strict)"("Val(Sgnl)"=w832) -> ()  [unwired: 2 in, 2 out]
            n396 = Divide(x=w838, y=w844) -> (x/y=w842:dbl)
            n397 = And(x=w845, y=w812) -> (x .and. y?=w813:bool)
            n398 = property on="Y in Range" class="Bool (strict)"("Val(Sgnl)"=w813) -> ()  [unwired: 2 in, 2 out]
            n399 = property on="Y mm/rev" class="DigNum (strict)"() -> ("Value"=w841:dbl)  [unwired: 2 in, 2 out]
            n400 = Multiply(x=w842, y=w841) -> (x*y=w840:dbl)
            n401 = Add(x=w840, y=w839) -> (x+y=w836:dbl)
            n402 = property on="Y Position mm PV" class="DigNum (strict)"("Val(Sgnl)"=w836) -> ()  [unwired: 2 in, 2 out]
          }
          frame #1 {
            n403 = property on="Y Scan" class="Bool (strict)"() -> ("Value"=w850:bool)  [unwired: 2 in, 2 out]
            n404 = Or(x=w849, y=w850) -> (x .or. y?=w851:bool)
            n405 = case shown="True" w851 {
              frame False {
                n406 = property on="Y Scan OK" class="Bool"("DisabledEnum"=T2."Enabled" ("Disabled")) -> ()  [unwired: 2 in, 2 out]
                n407 = property on="Y Go" class="Bool"("DisabledEnum"=T2."Enabled" ("Disabled")) -> ()  [unwired: 2 in, 2 out]
              }
              frame True {
                n408 = property on="Y Scan OK" class="Bool"("DisabledEnum"=T2."Disabled and Grayed Out" ("Disabled")) -> ()  [unwired: 2 in, 2 out]
                n409 = property on="Y Go" class="Bool"("DisabledEnum"=T2."Disabled and Grayed Out" ("Disabled")) -> ()  [unwired: 2 in, 2 out]
              }
            }
          }
          frame #2 {
            n410 = case shown="False" w860 {
              tunnel: w861 -> [w866 w871]
              tunnel: [w868 w871] -> w862
              tunnel: [w867 w870] -> w863
              tunnel: w864 -> [w865 w870]
              frame False {
                n411 = call "Applied Send Command.vi"("error in (no error)"=w865, "Command"=T1."Stop & Kill Buffer", "VISA resource name"=w866) -> ("error out"=w867:errorcluster, "VISA resource name out"=w868:refnum<visa-resource-name>)  [unwired: 4 in, 1 out]
              }
              frame True {
              }
            }
          }
          frame #3 {
            n412 = property on="Y Backlash corr" class="Bool (strict)"() -> ("Value"=w878:bool)  [unwired: 2 in, 2 out]
            n413 = Implies(1:w877, 2:w878) -> (0:w876:bool)
            n414 = case shown="False" w876 {
              tunnel: w875 -> [w881 w910]
              tunnel: w874 -> [w882 w911]
              tunnel: [w879 w910] -> w873
              tunnel: [w880 w911] -> w872
              frame False {
                w888 = 0.1 ("Delay Time (s)")
                # "Backlash"
                n415 = property on="Y Backlash" class="DigNum (strict)"() -> ("Value"=w883:i32)  [unwired: 2 in, 2 out]
                n416 = To Long Integer(number=w883) -> (32bit integer=w906:i32)
                n417 = property on="Y Backlash corr" class="Bool (strict)"("Val(Sgnl)"=FALSE ("Value (Signaling)")) -> ()  [unwired: 2 in, 2 out]
                n418 = Number To Decimal String(number=w883) -> (decimal integer string=w901:string)  [unwired: 1 in]
                n419 = Negate(x=w906) -> (-x=w907:i32)
                n420 = property on="Y Backlash steps/sec" class="DigNum (strict)"() -> ("Value"=w884:i32)  [unwired: 2 in, 2 out]
                n421 = Number To Decimal String(number=w907) -> (decimal integer string=w900:string)  [unwired: 1 in]
                n422 = property on="Y steps/rev" class="DigNum (strict)"() -> ("Value"=w887:u32)  [unwired: 2 in, 2 out]
                n423 = Divide(x=w884, y=w887) -> (x/y=w886:dbl)
                n424 = Number To Fractional String(number=w886) -> (F-format string=w885:string)  [unwired: 3 in]
                n425 = call "Applied Send Command.vi"("error in (no error)"=w881, "Extra"=w885, "Command"=T1."Velocity Setting", "VISA resource name"=w882) -> ("error out"=w890:errorcluster, "VISA resource name out"=w896:refnum<visa-resource-name>)  [unwired: 3 in, 1 out]
                n426 = call "Time Delay41"("error in (no error)"=w890, "Delay Time (s)"=w888) -> ("error out"=w889:errorcluster)  [unwired: 9 in]
                n427 = call "Applied Send Command.vi"("error in (no error)"=w889, "Extra"=w901, "Command"=T1."Distance or Position", "VISA resource name"=w896) -> ("error out"=w895:errorcluster, "VISA resource name out"=w902:refnum<visa-resource-name>)  [unwired: 3 in, 1 out]
                n428 = call "Time Delay38"("error in (no error)"=w895, "Delay Time (s)"=w888) -> ("error out"=w894:errorcluster)  [unwired: 9 in]
                n429 = call "Applied Send Command.vi"("error in (no error)"=w894, "Command"=T1."Feed to Length", "VISA resource name"=w902) -> ("error out"=w893:errorcluster, "VISA resource name out"=w899:refnum<visa-resource-name>)  [unwired: 4 in, 1 out]
                n430 = call "Applied Send Command.vi"("Extra"=w900, "Command"=T1."Distance or Position", "VISA resource name"=w899) -> ("error out"=w892:errorcluster, "VISA resource name out"=w898:refnum<visa-resource-name>)  [unwired: 4 in, 1 out]
                n431 = call "Time Delay39"("error in (no error)"=w893, "Delay Time (s)"=w888) -> ()  [unwired: 9 in, 1 out]
                n432 = call "Time Delay40"("error in (no error)"=w892, "Delay Time (s)"=w888) -> ("error out"=w891:errorcluster)  [unwired: 9 in]
                n433 = call "Applied Send Command.vi"("error in (no error)"=w891, "Command"=T1."Feed to Length", "VISA resource name"=w898) -> ("error out"=w879:errorcluster, "VISA resource name out"=w880:refnum<visa-resource-name>)  [unwired: 4 in, 1 out]
              }
              frame True {
              }
            }
          }
        }
        n434 = Multiply(x=360.0, y=w445) -> (x*y=w448:dbl)
        n435 = property on="atan Y/Z" class="DigNum (strict)"("Val(Sgnl)"=w448) -> ()  [unwired: 2 in, 2 out]
      }
      event "Reset Y Position mm", "Reset X Position mm", "Reset Z Position mm", "Reset R Position deg": Value Change {
        n436 = event-data() -> ()  [unwired: 1 in, 5 out]
        n437 = property on="Z steps/rev" class="DigNum (strict)"() -> ("Value"=w923:u32)  [unwired: 2 in, 2 out]
        n438 = property on="X steps/rev" class="DigNum (strict)"() -> ("Value"=w932:u32)  [unwired: 2 in, 2 out]
        n439 = property on="Y steps/rev" class="DigNum (strict)"() -> ("Value"=w941:u32)  [unwired: 2 in, 2 out]
        n440 = property on="R steps/rev" class="DigNum (strict)"() -> ("Value"=w914:u32)  [unwired: 2 in, 2 out]
        n441 = property on="R offset deg" class="DigNum (strict)"() -> ("Value"=w912:dbl)  [unwired: 2 in, 2 out]
        n442 = property on="Z offset mm" class="DigNum (strict)"() -> ("Value"=w921:dbl)  [unwired: 2 in, 2 out]
        n443 = property on="X offset mm" class="DigNum (strict)"() -> ("Value"=w930:dbl)  [unwired: 2 in, 2 out]
        n444 = property on="Y offset mm" class="DigNum (strict)"() -> ("Value"=w939:dbl)  [unwired: 2 in, 2 out]
        n445 = To Double Precision Float(number=w914) -> (double precision float=w917:dbl)
        n446 = To Double Precision Float(number=w932) -> (double precision float=w935:dbl)
        n447 = To Double Precision Float(number=w941) -> (double precision float=w944:dbl)
        n448 = property on="Reset Z Position mm" class="DigNum (strict)"() -> ("Value"=w929:dbl)  [unwired: 2 in, 2 out]
        n449 = property on="Reset X Position mm" class="DigNum (strict)"() -> ("Value"=w938:dbl)  [unwired: 2 in, 2 out]
        n450 = property on="Reset Y Position mm" class="DigNum (strict)"() -> ("Value"=w947:dbl)  [unwired: 2 in, 2 out]
        n451 = property on="Reset R Position deg" class="DigNum (strict)"() -> ("Value"=w920:dbl)  [unwired: 2 in, 2 out]
        n452 = Subtract(x=w929, y=w921) -> (x-y=w928:dbl)
        n453 = Subtract(x=w920, y=w912) -> (x-y=w919:dbl)
        n454 = Subtract(x=w938, y=w930) -> (x-y=w937:dbl)
        n455 = Subtract(x=w947, y=w939) -> (x-y=w946:dbl)
        n456 = property on="Z mm/rev" class="DigNum (strict)"() -> ("Value"=w922:dbl)  [unwired: 2 in, 2 out]
        n457 = property on="X mm/rev" class="DigNum (strict)"() -> ("Value"=w931:dbl)  [unwired: 2 in, 2 out]
        n458 = property on="Y mm/rev" class="DigNum (strict)"() -> ("Value"=w940:dbl)  [unwired: 2 in, 2 out]
        n459 = property on="R deg/rev" class="DigNum (strict)"() -> ("Value"=w913:dbl)  [unwired: 2 in, 2 out]
        n460 = Divide(x=w919, y=w913) -> (x/y=w918:dbl)
        n461 = Divide(x=w937, y=w931) -> (x/y=w936:dbl)
        n462 = Divide(x=w946, y=w940) -> (x/y=w945:dbl)
        n463 = Divide(x=w928, y=w922) -> (x/y=w927:dbl)
        n464 = To Double Precision Float(number=w923) -> (double precision float=w926:dbl)
        n465 = Multiply(x=w927, y=w926) -> (x*y=w925:dbl)
        n466 = Multiply(x=w918, y=w917) -> (x*y=w916:dbl)
        n467 = Multiply(x=w936, y=w935) -> (x*y=w934:dbl)
        n468 = Multiply(x=w945, y=w944) -> (x*y=w943:dbl)
        n469 = To Long Integer(number=w925) -> (32bit integer=w924:i32)
        n470 = To Long Integer(number=w916) -> (32bit integer=w915:i32)
        n471 = To Long Integer(number=w934) -> (32bit integer=w933:i32)
        n472 = To Long Integer(number=w943) -> (32bit integer=w942:i32)
        n473 = property on="Reset Z Motor Steps" class="DigNum (strict)"("Val(Sgnl)"=w924) -> ()  [unwired: 2 in, 2 out]
        n474 = property on="Reset R Motor Steps" class="DigNum (strict)"("Val(Sgnl)"=w915) -> ()  [unwired: 2 in, 2 out]
        n475 = property on="Reset X Motor Steps" class="DigNum (strict)"("Val(Sgnl)"=w933) -> ()  [unwired: 2 in, 2 out]
        n476 = property on="Reset Y Motor Steps" class="DigNum (strict)"("Val(Sgnl)"=w942) -> ()  [unwired: 2 in, 2 out]
      }
      event "Y Velocity SP step/sec", "X Velocity SP step/sec", "R Velocity SP step/sec", "Z Velocity SP step/sec", "Y Step SP", "X Step SP", "Z Step SP", "R Step SP": Value Change {
        n477 = event-data() -> ()  [unwired: 1 in, 5 out]
        n478 = property on="Z Step SP" class="DigNum (strict)"() -> ("Value"=w964:i32)  [unwired: 2 in, 2 out]
        n479 = property on="Y Step SP" class="DigNum (strict)"() -> ("Value"=w980:i32)  [unwired: 2 in, 2 out]
        n480 = property on="X Step SP" class="DigNum (strict)"() -> ("Value"=w972:i32)  [unwired: 2 in, 2 out]
        n481 = property on="Z steps/rev" class="DigNum (strict)"() -> ("Value"=w991:u32)  [unwired: 2 in, 2 out]
        n482 = property on="Z steps/rev" class="DigNum (strict)"() -> ("Value"=w962:u32)  [unwired: 2 in, 2 out]
        n483 = property on="R Step SP" class="DigNum (strict)"() -> ("Value"=w956:i32)  [unwired: 2 in, 2 out]
        n484 = property on="Y steps/rev" class="DigNum (strict)"() -> ("Value"=w1003:u32)  [unwired: 2 in, 2 out]
        n485 = property on="Y steps/rev" class="DigNum (strict)"() -> ("Value"=w978:u32)  [unwired: 2 in, 2 out]
        n486 = property on="X steps/rev" class="DigNum (strict)"() -> ("Value"=w997:u32)  [unwired: 2 in, 2 out]
        n487 = property on="X steps/rev" class="DigNum (strict)"() -> ("Value"=w970:u32)  [unwired: 2 in, 2 out]
        n488 = property on="R steps/rev" class="DigNum (strict)"() -> ("Value"=w985:u32)  [unwired: 2 in, 2 out]
        n489 = property on="R steps/rev" class="DigNum (strict)"() -> ("Value"=w954:u32)  [unwired: 2 in, 2 out]
        n490 = property on="R offset deg" class="DigNum (strict)"() -> ("Value"=w953:dbl)  [unwired: 2 in, 2 out]
        n491 = property on="Z offset mm" class="DigNum (strict)"() -> ("Value"=w961:dbl)  [unwired: 2 in, 2 out]
        n492 = property on="Y offset mm" class="DigNum (strict)"() -> ("Value"=w977:dbl)  [unwired: 2 in, 2 out]
        n493 = property on="X offset mm" class="DigNum (strict)"() -> ("Value"=w969:dbl)  [unwired: 2 in, 2 out]
        n494 = To Double Precision Float(number=w991) -> (double precision float=w996:dbl)
        n495 = To Double Precision Float(number=w964) -> (double precision float=w965:dbl)
        n496 = To Double Precision Float(number=w962) -> (double precision float=w968:dbl)
        n497 = To Double Precision Float(number=w985) -> (double precision float=w990:dbl)
        n498 = To Double Precision Float(number=w956) -> (double precision float=w957:dbl)
        n499 = To Double Precision Float(number=w954) -> (double precision float=w960:dbl)
        n500 = To Double Precision Float(number=w980) -> (double precision float=w981:dbl)
        n501 = To Double Precision Float(number=w978) -> (double precision float=w984:dbl)
        n502 = To Double Precision Float(number=w997) -> (double precision float=w1002:dbl)
        n503 = To Double Precision Float(number=w972) -> (double precision float=w973:dbl)
        n504 = To Double Precision Float(number=w970) -> (double precision float=w976:dbl)
        n505 = Divide(x=w965, y=w968) -> (x/y=w967:dbl)
        n506 = Divide(x=w981, y=w984) -> (x/y=w983:dbl)
        n507 = Divide(x=w973, y=w976) -> (x/y=w975:dbl)
        n508 = Divide(x=w957, y=w960) -> (x/y=w959:dbl)
        n509 = property on="Z Velocity SP step/sec" class="DigNum (strict)"() -> ("Value"=w993:i32)  [unwired: 2 in, 2 out]
        n510 = property on="Z mm/rev" class="DigNum (strict)"() -> ("Value"=w951:dbl)  [unwired: 2 in, 2 out]
        n511 = property on="Y Velocity SP step/sec" class="DigNum (strict)"() -> ("Value"=w1005:i32)  [unwired: 2 in, 2 out]
        n512 = property on="Y mm/rev" class="DigNum (strict)"() -> ("Value"=w949:dbl)  [unwired: 2 in, 2 out]
        n513 = property on="X Velocity SP step/sec" class="DigNum (strict)"() -> ("Value"=w999:i32)  [unwired: 2 in, 2 out]
        n514 = property on="X mm/rev" class="DigNum (strict)"() -> ("Value"=w950:dbl)  [unwired: 2 in, 2 out]
        n515 = property on="R Velocity SP step/sec" class="DigNum (strict)"() -> ("Value"=w987:i32)  [unwired: 2 in, 2 out]
        n516 = property on="R deg/rev" class="DigNum (strict)"() -> ("Value"=w952:dbl)  [unwired: 2 in, 2 out]
        n517 = Multiply(x=w967, y=w951) -> (x*y=w966:dbl)
        n518 = Multiply(x=w959, y=w952) -> (x*y=w958:dbl)
        n519 = Multiply(x=w983, y=w949) -> (x*y=w982:dbl)
        n520 = Multiply(x=w975, y=w950) -> (x*y=w974:dbl)
        n521 = To Double Precision Float(number=w993) -> (double precision float=w994:dbl)
        n522 = To Double Precision Float(number=w987) -> (double precision float=w988:dbl)
        n523 = To Double Precision Float(number=w1005) -> (double precision float=w1006:dbl)
        n524 = To Double Precision Float(number=w1003) -> (double precision float=w1008:dbl)
        n525 = To Double Precision Float(number=w999) -> (double precision float=w1000:dbl)
        n526 = Divide(x=w994, y=w996) -> (x/y=w995:dbl)
        n527 = Add(x=w966, y=w961) -> (x+y=w963:dbl)
        n528 = Divide(x=w988, y=w990) -> (x/y=w989:dbl)
        n529 = Add(x=w958, y=w953) -> (x+y=w955:dbl)
        n530 = Divide(x=w1006, y=w1008) -> (x/y=w1007:dbl)
        n531 = Add(x=w982, y=w977) -> (x+y=w979:dbl)
        n532 = Divide(x=w1000, y=w1002) -> (x/y=w1001:dbl)
        n533 = Add(x=w974, y=w969) -> (x+y=w971:dbl)
        n534 = Multiply(x=w995, y=w951) -> (x*y=w992:dbl)
        n535 = Multiply(x=w989, y=w952) -> (x*y=w986:dbl)
        n536 = Multiply(x=w1007, y=w949) -> (x*y=w1004:dbl)
        n537 = Multiply(x=w1001, y=w950) -> (x*y=w998:dbl)
        n538 = property on="Z Position MV mm" class="DigNum (strict)"("Val(Sgnl)"=w963) -> ()  [unwired: 2 in, 2 out]
        n539 = property on="R Position MV deg" class="DigNum (strict)"("Val(Sgnl)"=w955) -> ()  [unwired: 2 in, 2 out]
        n540 = property on="Y Position MV mm" class="DigNum (strict)"("Val(Sgnl)"=w979) -> ()  [unwired: 2 in, 2 out]
        n541 = property on="X Position MV mm" class="DigNum (strict)"("Val(Sgnl)"=w971) -> ()  [unwired: 2 in, 2 out]
        n542 = property on="Z Velocity MV mm/sec" class="DigNum (strict)"("Val(Sgnl)"=w992) -> ()  [unwired: 2 in, 2 out]
        n543 = property on="Y Velocity MV mm/sec" class="DigNum (strict)"("Val(Sgnl)"=w1004) -> ()  [unwired: 2 in, 2 out]
        n544 = property on="X Velocity MV mm/sec" class="DigNum (strict)"("Val(Sgnl)"=w998) -> ()  [unwired: 2 in, 2 out]
        n545 = Absolute Value(x=w986) -> (abs(x)=w948:dbl)
        n546 = property on="R Velocity MVdeg/sec" class="DigNum (strict)"("Val(Sgnl)"=w948) -> ()  [unwired: 2 in, 2 out]
      }
      event "Y Scan Length SP steps", "Y Scan Velocity SP steps/sec", "X Scan Velocity SP steps/sec", "X Scan Length SP steps", "Z Scan Velocity SP steps/sec", "Z Scan Length SP steps", "R Scan Velocity SP steps/sec", "R Scan Length SP steps": Value Change {
        n547 = event-data() -> ()  [unwired: 1 in, 5 out]
        n548 = property on="R Step PV" class="DigNum (strict)"() -> ("Value"=w1036:i32)  [unwired: 2 in, 2 out]
        n549 = property on="Z steps/rev" class="DigNum (strict)"() -> ("Value"=w1052:u32)  [unwired: 2 in, 2 out]
        n550 = property on="X steps/rev" class="DigNum (strict)"() -> ("Value"=w1079:u32)  [unwired: 2 in, 2 out]
        n551 = property on="Y steps/rev" class="DigNum (strict)"() -> ("Value"=w1065:u32)  [unwired: 2 in, 2 out]
        n552 = property on="X Step PV" class="DigNum (strict)"() -> ("Value"=w1077:i32)  [unwired: 2 in, 2 out]
        n553 = property on="Y Step PV" class="DigNum (strict)"() -> ("Value"=w1063:i32)  [unwired: 2 in, 2 out]
        n554 = property on="Z Step PV" class="DigNum (strict)"() -> ("Value"=w1050:i32)  [unwired: 2 in, 2 out]
        n555 = property on="R steps/rev" class="DigNum (strict)"() -> ("Value"=w1038:u32)  [unwired: 2 in, 2 out]
        n556 = To Double Precision Float(number=w1077) -> (double precision float=w1030:dbl)
        n557 = To Double Precision Float(number=w1063) -> (double precision float=w1029:dbl)
        n558 = To Double Precision Float(number=w1050) -> (double precision float=w1028:dbl)
        n559 = To Double Precision Float(number=w1036) -> (double precision float=w1027:dbl)
        n560 = To Double Precision Float(number=w1052) -> (double precision float=w1049:dbl)
        n561 = To Double Precision Float(number=w1038) -> (double precision float=w1035:dbl)
        n562 = To Double Precision Float(number=w1079) -> (double precision float=w1076:dbl)
        n563 = To Double Precision Float(number=w1065) -> (double precision float=w1020:dbl)
        n564 = property on="X Step SP" class="DigNum (strict)"() -> ("Maximum"=w1083:dbl)  [unwired: 2 in, 2 out]
        n565 = property on="Y Step SP" class="DigNum (strict)"() -> ("Maximum"=w1069:dbl)  [unwired: 2 in, 2 out]
        n566 = property on="Z Step SP" class="DigNum (strict)"() -> ("Maximum"=w1056:dbl)  [unwired: 2 in, 2 out]
        n567 = property on="R Step SP" class="DigNum (strict)"() -> ("Maximum"=w1044:dbl)  [unwired: 2 in, 2 out]
        n568 = property on="Z Scan Length SP steps" class="DigNum (strict)"() -> ("Value"=w1053:i32)  [unwired: 2 in, 2 out]
        n569 = property on="X Scan Length SP steps" class="DigNum (strict)"() -> ("Value"=w1075:i32)  [unwired: 2 in, 2 out]
        n570 = property on="Y Scan Length SP steps" class="DigNum (strict)"() -> ("Value"=w1066:i32)  [unwired: 2 in, 2 out]
        n571 = property on="R Scan Length SP steps" class="DigNum (strict)"() -> ("Value"=w1039:i32)  [unwired: 2 in, 2 out]
        n572 = property on="X Step SP" class="DigNum (strict)"() -> ("Minimum"=w1084:dbl)  [unwired: 2 in, 2 out]
        n573 = property on="Y Step SP" class="DigNum (strict)"() -> ("Minimum"=w1070:dbl)  [unwired: 2 in, 2 out]
        n574 = property on="Z Step SP" class="DigNum (strict)"() -> ("Minimum"=w1057:dbl)  [unwired: 2 in, 2 out]
        n575 = property on="R Step SP" class="DigNum (strict)"() -> ("Minimum"=w1041:dbl)  [unwired: 2 in, 2 out]
        n576 = property on="Z Scan Velocity SP steps/sec" class="DigNum (strict)"() -> ("Value"=w1048:i32)  [unwired: 2 in, 2 out]
        n577 = property on="R Scan Velocity SP steps/sec" class="DigNum (strict)"() -> ("Value"=w1034:i32)  [unwired: 2 in, 2 out]
        n578 = property on="X Scan Velocity SP steps/sec" class="DigNum (strict)"() -> ("Value"=w1080:i32)  [unwired: 2 in, 2 out]
        n579 = property on="Y Scan Velocity SP steps/sec" class="DigNum (strict)"() -> ("Value"=w1062:i32)  [unwired: 2 in, 2 out]
        n580 = Subtract(x=w1084, y=w1030) -> (x-y=w1085:dbl)
        n581 = Subtract(x=w1083, y=w1030) -> (x-y=w1082:dbl)
        n582 = Subtract(x=w1070, y=w1029) -> (x-y=w1071:dbl)
        n583 = Subtract(x=w1069, y=w1029) -> (x-y=w1068:dbl)
        n584 = Subtract(x=w1057, y=w1028) -> (x-y=w1058:dbl)
        n585 = Subtract(x=w1056, y=w1028) -> (x-y=w1055:dbl)
        n586 = Subtract(x=w1041, y=w1027) -> (x-y=w1042:dbl)
        n587 = Subtract(x=w1044, y=w1027) -> (x-y=w1043:dbl)
        n588 = To Double Precision Float(number=w1053) -> (double precision float=w1026:dbl)
        n589 = To Double Precision Float(number=w1039) -> (double precision float=w1024:dbl)
        n590 = To Double Precision Float(number=w1075) -> (double precision float=w1015:dbl)
        n591 = To Double Precision Float(number=w1066) -> (double precision float=w1019:dbl)
        n592 = property on="X Scan Length SP steps" class="DigNum (strict)"("Minimum"=w1085) -> ()  [unwired: 2 in, 2 out]
        n593 = property on="X Scan Length SP steps" class="DigNum (strict)"("Maximum"=w1082) -> ()  [unwired: 2 in, 2 out]
        n594 = property on="Y Scan Length SP steps" class="DigNum (strict)"("Minimum"=w1071) -> ()  [unwired: 2 in, 2 out]
        n595 = property on="Y Scan Length SP steps" class="DigNum (strict)"("Maximum"=w1068) -> ()  [unwired: 2 in, 2 out]
        n596 = property on="Z Scan Length SP steps" class="DigNum (strict)"("Minimum"=w1058) -> ()  [unwired: 2 in, 2 out]
        n597 = property on="Z Scan Length SP steps" class="DigNum (strict)"("Maximum"=w1055) -> ()  [unwired: 2 in, 2 out]
        n598 = property on="R Scan Length SP steps" class="DigNum (strict)"("Minimum"=w1042) -> ()  [unwired: 2 in, 2 out]
        n599 = property on="R Scan Length SP steps" class="DigNum (strict)"("Maximum"=w1043) -> ()  [unwired: 2 in, 2 out]
        n600 = Divide(x=w1026, y=w1049) -> (x/y=w1054:dbl)
        n601 = Divide(x=w1015, y=w1076) -> (x/y=w1074:dbl)
        n602 = Divide(x=w1019, y=w1020) -> (x/y=w1067:dbl)
        n603 = Divide(x=w1024, y=w1035) -> (x/y=w1040:dbl)
        n604 = To Double Precision Float(number=w1048) -> (double precision float=w1025:dbl)
        n605 = To Double Precision Float(number=w1080) -> (double precision float=w1014:dbl)
        n606 = To Double Precision Float(number=w1062) -> (double precision float=w1018:dbl)
        n607 = To Double Precision Float(number=w1034) -> (double precision float=w1023:dbl)
        n608 = property on="Z mm/rev" class="DigNum (strict)"() -> ("Value"=w1051:dbl)  [unwired: 2 in, 2 out]
        n609 = property on="X mm/rev" class="DigNum (strict)"() -> ("Value"=w1078:dbl)  [unwired: 2 in, 2 out]
        n610 = property on="Y mm/rev" class="DigNum (strict)"() -> ("Value"=w1064:dbl)  [unwired: 2 in, 2 out]
        n611 = property on="R deg/rev" class="DigNum (strict)"() -> ("Value"=w1037:dbl)  [unwired: 2 in, 2 out]
        n612 = Multiply(x=w1054, y=w1051) -> (x*y=w1046:dbl)
        n613 = Divide(x=w1026, y=w1025) -> (x/y=w1021:dbl)
        n614 = Divide(x=w1025, y=w1049) -> (x/y=w1047:dbl)
        n615 = Multiply(x=w1040, y=w1037) -> (x*y=w1032:dbl)
        n616 = Divide(x=w1024, y=w1023) -> (x/y=w1022:dbl)
        n617 = Divide(x=w1023, y=w1035) -> (x/y=w1033:dbl)
        n618 = Multiply(x=w1078, y=w1074) -> (x*y=w1072:dbl)
        n619 = Divide(x=w1015, y=w1014) -> (x/y=w1016:dbl)
        n620 = Divide(x=w1014, y=w1076) -> (x/y=w1081:dbl)
        n621 = Multiply(x=w1067, y=w1064) -> (x*y=w1060:dbl)
        n622 = Divide(x=w1019, y=w1018) -> (x/y=w1017:dbl)
        n623 = Divide(x=w1018, y=w1020) -> (x/y=w1061:dbl)
        n624 = Multiply(x=w1051, y=w1047) -> (x*y=w1045:dbl)
        n625 = Multiply(x=w1037, y=w1033) -> (x*y=w1031:dbl)
        n626 = Multiply(x=w1081, y=w1078) -> (x*y=w1073:dbl)
        n627 = Multiply(x=w1064, y=w1061) -> (x*y=w1059:dbl)
        n628 = Absolute Value(x=w1021) -> (abs(x)=→"Z Scan Duration":dbl)
        n629 = Absolute Value(x=w1022) -> (abs(x)=→"R Scan Duration":dbl)
        n630 = Absolute Value(x=w1016) -> (abs(x)=→"X Scan Duration":dbl)
        n631 = Absolute Value(x=w1017) -> (abs(x)=→"Y Scan Duration":dbl)
        n632 = property on="Z Scan length MV mm" class="DigNum (strict)"("Value"=w1046) -> ()  [unwired: 2 in, 2 out]
        n633 = property on="R Scan length MV deg" class="DigNum (strict)"("Value"=w1032) -> ()  [unwired: 2 in, 2 out]
        n634 = property on="X Scan length MV mm" class="DigNum (strict)"("Val(Sgnl)"=w1072) -> ()  [unwired: 2 in, 2 out]
        n635 = property on="Y Scan length MV mm" class="DigNum (strict)"("Value"=w1060) -> ()  [unwired: 2 in, 2 out]
        n636 = Absolute Value(x=w1031) -> (abs(x)=w1013:dbl)
        n637 = property on="Z Scan velocity MV mm/sec" class="DigNum (strict)"("Val(Sgnl)"=w1045) -> ()  [unwired: 2 in, 2 out]
        n638 = property on="X Scan velocity MV mm/sec" class="DigNum (strict)"("Value"=w1073) -> ()  [unwired: 2 in, 2 out]
        n639 = property on="Y Scan velocity MV mm/sec" class="DigNum (strict)"("Val(Sgnl)"=w1059) -> ()  [unwired: 2 in, 2 out]
        n640 = property on="R Scan Velocity SP deg/sec" class="DigNum (strict)"("Val(Sgnl)"=w1013) -> ()  [unwired: 2 in, 2 out]
      }
      event "Y Move Set": Mouse Down {
        n641 = event-data() -> ()  [unwired: 1 in, 7 out]
        n642 = property on="Y steps/rev" class="DigNum (strict)"() -> ("Value"=w1102:u32)  [unwired: 2 in, 2 out]
        n643 = property on="Y offset mm" class="DigNum (strict)"() -> ("Value"=w1100:dbl)  [unwired: 2 in, 2 out]
        n644 = property on="Y Position SP mm" class="DigNum (strict)"() -> ("Value"=w1099:dbl)  [unwired: 2 in, 2 out]
        n645 = property on="Y Velocity SP step/sec" class="DigNum (strict)"() -> ("Maximum"=w1089:dbl)  [unwired: 2 in, 2 out]
        n646 = property on="Y Velocity SP step/sec" class="DigNum (strict)"() -> ("Minimum"=w1088:dbl)  [unwired: 2 in, 2 out]
        n647 = Subtract(x=w1099, y=w1100) -> (x-y=w1103:dbl)
        n648 = property on="Y Velocity SP mm/sec" class="DigNum (strict)"() -> ("Value"=w1093:dbl)  [unwired: 2 in, 2 out]
        n649 = property on="Y mm/rev" class="DigNum (strict)"() -> ("Value"=w1086:dbl)  [unwired: 2 in, 2 out]
        n650 = Divide(x=w1103, y=w1086) -> (x/y=w1104:dbl)
        n651 = Divide(x=w1093, y=w1086) -> (x/y=w1094:dbl)
        n652 = To Double Precision Float(number=w1102) -> (double precision float=w1087:dbl)
        n653 = Multiply(x=w1104, y=w1087) -> (x*y=w1098:dbl)
        n654 = Multiply(x=w1094, y=w1087) -> (x*y=w1091:dbl)
        n655 = property on="Y Step SP" class="DigNum (strict)"() -> ("Maximum"=w1096:dbl)  [unwired: 2 in, 2 out]
        n656 = property on="Y Step SP" class="DigNum (strict)"() -> ("Minimum"=w1095:dbl)  [unwired: 2 in, 2 out]
        n657 = In Range and Coerce(upper limit=w1089, x=w1091, lower limit=w1088) -> (coerced(x)=w1090:dbl)  [unwired: 1 out]
        n658 = To Long Integer(number=w1090) -> (32bit integer=w1092:i32)
        n659 = In Range and Coerce(upper limit=w1096, x=w1098, lower limit=w1095) -> (coerced(x)=w1097:dbl)  [unwired: 1 out]
        n660 = To Long Integer(number=w1097) -> (32bit integer=w1101:i32)
        n661 = property on="Y Velocity SP step/sec" class="DigNum (strict)"("Val(Sgnl)"=w1092) -> ()  [unwired: 2 in, 2 out]
        n662 = property on="Y Step SP" class="DigNum (strict)"("Val(Sgnl)"=w1101) -> ()  [unwired: 2 in, 2 out]
      }
      event "X Move Set": Mouse Down {
        n663 = event-data() -> ()  [unwired: 1 in, 7 out]
        n664 = property on="X steps/rev" class="DigNum (strict)"() -> ("Value"=w1121:u32)  [unwired: 2 in, 2 out]
        n665 = property on="X offset mm" class="DigNum (strict)"() -> ("Value"=w1119:dbl)  [unwired: 2 in, 2 out]
        n666 = property on="X Position SP mm" class="DigNum (strict)"() -> ("Value"=w1118:dbl)  [unwired: 2 in, 2 out]
        n667 = property on="X Velocity SP step/sec" class="DigNum (strict)"() -> ("Maximum"=w1108:dbl)  [unwired: 2 in, 2 out]
        n668 = property on="X Velocity SP step/sec" class="DigNum (strict)"() -> ("Minimum"=w1107:dbl)  [unwired: 2 in, 2 out]
        n669 = Subtract(x=w1118, y=w1119) -> (x-y=w1122:dbl)
        n670 = property on="X Velocity SP mm/sec" class="DigNum (strict)"() -> ("Value"=w1112:dbl)  [unwired: 2 in, 2 out]
        n671 = property on="X mm/rev" class="DigNum (strict)"() -> ("Value"=w1105:dbl)  [unwired: 2 in, 2 out]
        n672 = Divide(x=w1122, y=w1105) -> (x/y=w1123:dbl)
        n673 = Divide(x=w1112, y=w1105) -> (x/y=w1113:dbl)
        n674 = To Double Precision Float(number=w1121) -> (double precision float=w1106:dbl)
        n675 = Multiply(x=w1123, y=w1106) -> (x*y=w1117:dbl)
        n676 = Multiply(x=w1113, y=w1106) -> (x*y=w1110:dbl)
        n677 = property on="X Step SP" class="DigNum (strict)"() -> ("Maximum"=w1115:dbl)  [unwired: 2 in, 2 out]
        n678 = property on="X Step SP" class="DigNum (strict)"() -> ("Minimum"=w1114:dbl)  [unwired: 2 in, 2 out]
        n679 = In Range and Coerce(upper limit=w1108, x=w1110, lower limit=w1107) -> (coerced(x)=w1109:dbl)  [unwired: 1 out]
        n680 = To Long Integer(number=w1109) -> (32bit integer=w1111:i32)
        n681 = In Range and Coerce(upper limit=w1115, x=w1117, lower limit=w1114) -> (coerced(x)=w1116:dbl)  [unwired: 1 out]
        n682 = To Long Integer(number=w1116) -> (32bit integer=w1120:i32)
        n683 = property on="X Velocity SP step/sec" class="DigNum (strict)"("Val(Sgnl)"=w1111) -> ()  [unwired: 2 in, 2 out]
        n684 = property on="X Step SP" class="DigNum (strict)"("Val(Sgnl)"=w1120) -> ()  [unwired: 2 in, 2 out]
      }
      event "Z Move Set": Mouse Down {
        n685 = event-data() -> ()  [unwired: 1 in, 7 out]
        n686 = property on="Z steps/rev" class="DigNum (strict)"() -> ("Value"=w1138:u32)  [unwired: 2 in, 2 out]
        n687 = property on="Z offset mm" class="DigNum (strict)"() -> ("Value"=w1136:dbl)  [unwired: 2 in, 2 out]
        n688 = property on="Z Position SP mm" class="DigNum (strict)"() -> ("Value"=w1135:dbl)  [unwired: 2 in, 2 out]
        n689 = property on="Z Velocity SP step/sec" class="DigNum (strict)"() -> ("Maximum"=w1125:dbl)  [unwired: 2 in, 2 out]
        n690 = property on="Z Velocity SP step/sec" class="DigNum (strict)"() -> ("Minimum"=w1124:dbl)  [unwired: 2 in, 2 out]
        n691 = Subtract(x=w1135, y=w1136) -> (x-y=w1139:dbl)
        n692 = property on="Z Velocity SP mm/sec" class="DigNum (strict)"() -> ("Value"=w1129:dbl)  [unwired: 2 in, 2 out]
        n693 = property on="Z mm/rev" class="DigNum (strict)"() -> ("Value"=w1141:dbl)  [unwired: 2 in, 2 out]
        n694 = Divide(x=w1139, y=w1141) -> (x/y=w1140:dbl)
        n695 = Divide(x=w1129, y=w1141) -> (x/y=w1130:dbl)
        n696 = To Double Precision Float(number=w1138) -> (double precision float=w1142:dbl)
        n697 = Multiply(x=w1140, y=w1142) -> (x*y=w1134:dbl)
        n698 = Multiply(x=w1130, y=w1142) -> (x*y=w1127:dbl)
        n699 = property on="Z Step SP" class="DigNum (strict)"() -> ("Maximum"=w1132:dbl)  [unwired: 2 in, 2 out]
        n700 = property on="Z Step SP" class="DigNum (strict)"() -> ("Minimum"=w1131:dbl)  [unwired: 2 in, 2 out]
        n701 = In Range and Coerce(upper limit=w1125, x=w1127, lower limit=w1124) -> (coerced(x)=w1126:dbl)  [unwired: 1 out]
        n702 = To Long Integer(number=w1126) -> (32bit integer=w1128:i32)
        n703 = In Range and Coerce(upper limit=w1132, x=w1134, lower limit=w1131) -> (coerced(x)=w1133:dbl)  [unwired: 1 out]
        n704 = To Long Integer(number=w1133) -> (32bit integer=w1137:i32)
        n705 = property on="Z Velocity SP step/sec" class="DigNum (strict)"("Val(Sgnl)"=w1128) -> ()  [unwired: 2 in, 2 out]
        n706 = property on="Z Step SP" class="DigNum (strict)"("Val(Sgnl)"=w1137) -> ()  [unwired: 2 in, 2 out]
      }
      event "R Move Set": Mouse Down {
        n707 = event-data() -> ()  [unwired: 1 in, 7 out]
        n708 = property on="R steps/rev" class="DigNum (strict)"() -> ("Value"=w1160:u32)  [unwired: 2 in, 2 out]
        n709 = property on="R offset deg" class="DigNum (strict)"() -> ("Value"=w1158:dbl)  [unwired: 2 in, 2 out]
        n710 = property on="R Position SP deg" class="DigNum (strict)"() -> ("Value"=w1157:dbl)  [unwired: 2 in, 2 out]
        n711 = property on="R Velocity SP step/sec" class="DigNum (strict)"() -> ("Maximum"=w1147:dbl)  [unwired: 2 in, 2 out]
        n712 = property on="R Velocity SP step/sec" class="DigNum (strict)"() -> ("Minimum"=w1146:dbl)  [unwired: 2 in, 2 out]
        n713 = Subtract(x=w1157, y=w1158) -> (x-y=w1161:dbl)
        n714 = property on="R Velocity SP deg/sec" class="DigNum (strict)"() -> ("Value"=w1151:dbl)  [unwired: 2 in, 2 out]
        n715 = property on="R deg/rev" class="DigNum (strict)"() -> ("Value"=w1144:dbl)  [unwired: 2 in, 2 out]
        n716 = Divide(x=w1161, y=w1144) -> (x/y=w1162:dbl)
        n717 = Divide(x=w1151, y=w1144) -> (x/y=w1152:dbl)
        n718 = To Double Precision Float(number=w1160) -> (double precision float=w1145:dbl)
        n719 = Multiply(x=w1162, y=w1145) -> (x*y=w1156:dbl)
        n720 = Multiply(x=w1152, y=w1145) -> (x*y=w1149:dbl)
        n721 = property on="R Step SP" class="DigNum (strict)"() -> ("Maximum"=w1154:dbl)  [unwired: 2 in, 2 out]
        n722 = property on="R Step SP" class="DigNum (strict)"() -> ("Minimum"=w1153:dbl)  [unwired: 2 in, 2 out]
        n723 = Absolute Value(x=w1149) -> (abs(x)=w1143:dbl)
        n724 = In Range and Coerce(upper limit=w1154, x=w1156, lower limit=w1153) -> (coerced(x)=w1155:dbl)  [unwired: 1 out]
        n725 = In Range and Coerce(upper limit=w1147, x=w1143, lower limit=w1146) -> (coerced(x)=w1148:dbl)  [unwired: 1 out]
        n726 = To Long Integer(number=w1155) -> (32bit integer=w1159:i32)
        n727 = To Long Integer(number=w1148) -> (32bit integer=w1150:i32)
        n728 = property on="R Step SP" class="DigNum (strict)"("Val(Sgnl)"=w1159) -> ()  [unwired: 2 in, 2 out]
        n729 = property on="R Velocity SP step/sec" class="DigNum (strict)"("Val(Sgnl)"=w1150) -> ()  [unwired: 2 in, 2 out]
      }
      event "Y Scan set": Mouse Down {
        n730 = event-data() -> ()  [unwired: 1 in, 7 out]
        n731 = property on="Y steps/rev" class="DigNum (strict)"() -> ("Value"=w1178:u32)  [unwired: 2 in, 2 out]
        n732 = To Double Precision Float(number=w1178) -> (double precision float=w1164:dbl)
        n733 = property on="Y mm/rev" class="DigNum (strict)"() -> ("Value"=w1163:dbl)  [unwired: 2 in, 2 out]
        n734 = property on="Y Scan Length SP mm" class="DigNum (strict)"() -> ("Value"=w1176:dbl)  [unwired: 2 in, 2 out]
        n735 = property on="Y Scan Velocity SP mm/sec" class="DigNum (strict)"() -> ("Value"=w1170:dbl)  [unwired: 2 in, 2 out]
        n736 = property on="Y Scan Velocity SP steps/sec" class="DigNum (strict)"() -> ("Maximum"=w1166:dbl)  [unwired: 2 in, 2 out]
        n737 = property on="Y Scan Velocity SP steps/sec" class="DigNum (strict)"() -> ("Minimum"=w1165:dbl)  [unwired: 2 in, 2 out]
        n738 = Divide(x=w1176, y=w1163) -> (x/y=w1179:dbl)
        n739 = Divide(x=w1170, y=w1163) -> (x/y=w1171:dbl)
        n740 = Multiply(x=w1179, y=w1164) -> (x*y=w1175:dbl)
        n741 = Multiply(x=w1171, y=w1164) -> (x*y=w1168:dbl)
        n742 = property on="Y Step SP" class="DigNum (strict)"() -> ("Maximum"=w1172:dbl)  [unwired: 2 in, 2 out]
        n743 = property on="Y Step SP" class="DigNum (strict)"() -> ("Minimum"=w1173:dbl)  [unwired: 2 in, 2 out]
        n744 = In Range and Coerce(upper limit=w1166, x=w1168, lower limit=w1165) -> (coerced(x)=w1167:dbl)  [unwired: 1 out]
        n745 = To Long Integer(number=w1167) -> (32bit integer=w1169:i32)
        n746 = In Range and Coerce(upper limit=w1172, x=w1175, lower limit=w1173) -> (coerced(x)=w1174:dbl)  [unwired: 1 out]
        n747 = To Long Integer(number=w1174) -> (32bit integer=w1177:i32)
        n748 = property on="Y Scan Velocity SP steps/sec" class="DigNum (strict)"("Val(Sgnl)"=w1169) -> ()  [unwired: 2 in, 2 out]
        n749 = property on="Y Scan Length SP steps" class="DigNum (strict)"("Val(Sgnl)"=w1177) -> ()  [unwired: 2 in, 2 out]
      }
      event "X Scan set": Mouse Down {
        n750 = event-data() -> ()  [unwired: 1 in, 7 out]
        n751 = property on="X steps/rev" class="DigNum (strict)"() -> ("Value"=w1195:u32)  [unwired: 2 in, 2 out]
        n752 = To Double Precision Float(number=w1195) -> (double precision float=w1181:dbl)
        n753 = property on="X mm/rev" class="DigNum (strict)"() -> ("Value"=w1180:dbl)  [unwired: 2 in, 2 out]
        n754 = property on="X Scan Length SP mm" class="DigNum (strict)"() -> ("Value"=w1193:dbl)  [unwired: 2 in, 2 out]
        n755 = property on="X Scan Velocity SP mm/sec" class="DigNum (strict)"() -> ("Value"=w1187:dbl)  [unwired: 2 in, 2 out]
        n756 = property on="X Scan Velocity SP steps/sec" class="DigNum (strict)"() -> ("Maximum"=w1183:dbl)  [unwired: 2 in, 2 out]
        n757 = property on="X Scan Velocity SP steps/sec" class="DigNum (strict)"() -> ("Minimum"=w1182:dbl)  [unwired: 2 in, 2 out]
        n758 = Divide(x=w1193, y=w1180) -> (x/y=w1196:dbl)
        n759 = Divide(x=w1187, y=w1180) -> (x/y=w1188:dbl)
        n760 = Multiply(x=w1196, y=w1181) -> (x*y=w1192:dbl)
        n761 = Multiply(x=w1188, y=w1181) -> (x*y=w1185:dbl)
        n762 = property on="X Step SP" class="DigNum (strict)"() -> ("Maximum"=w1189:dbl)  [unwired: 2 in, 2 out]
        n763 = property on="X Step SP" class="DigNum (strict)"() -> ("Minimum"=w1190:dbl)  [unwired: 2 in, 2 out]
        n764 = In Range and Coerce(upper limit=w1183, x=w1185, lower limit=w1182) -> (coerced(x)=w1184:dbl)  [unwired: 1 out]
        n765 = To Long Integer(number=w1184) -> (32bit integer=w1186:i32)
        n766 = In Range and Coerce(upper limit=w1189, x=w1192, lower limit=w1190) -> (coerced(x)=w1191:dbl)  [unwired: 1 out]
        n767 = To Long Integer(number=w1191) -> (32bit integer=w1194:i32)
        n768 = property on="X Scan Velocity SP steps/sec" class="DigNum (strict)"("Val(Sgnl)"=w1186) -> ()  [unwired: 2 in, 2 out]
        n769 = property on="X Scan Length SP steps" class="DigNum (strict)"("Val(Sgnl)"=w1194) -> ()  [unwired: 2 in, 2 out]
      }
      event "Z Scan set": Mouse Down {
        n770 = event-data() -> ()  [unwired: 1 in, 7 out]
        n771 = property on="Z steps/rev" class="DigNum (strict)"() -> ("Value"=w1212:u32)  [unwired: 2 in, 2 out]
        n772 = To Double Precision Float(number=w1212) -> (double precision float=w1198:dbl)
        n773 = property on="Z mm/rev" class="DigNum (strict)"() -> ("Value"=w1197:dbl)  [unwired: 2 in, 2 out]
        n774 = property on="Z Scan Length SP mm" class="DigNum (strict)"() -> ("Value"=w1210:dbl)  [unwired: 2 in, 2 out]
        n775 = property on="Z Scan Velocity SP mm/sec" class="DigNum (strict)"() -> ("Value"=w1204:dbl)  [unwired: 2 in, 2 out]
        n776 = property on="Z Scan Velocity SP steps/sec" class="DigNum (strict)"() -> ("Maximum"=w1200:dbl)  [unwired: 2 in, 2 out]
        n777 = property on="Z Scan Velocity SP steps/sec" class="DigNum (strict)"() -> ("Minimum"=w1199:dbl)  [unwired: 2 in, 2 out]
        n778 = Divide(x=w1210, y=w1197) -> (x/y=w1213:dbl)
        n779 = Divide(x=w1204, y=w1197) -> (x/y=w1205:dbl)
        n780 = Multiply(x=w1213, y=w1198) -> (x*y=w1209:dbl)
        n781 = Multiply(x=w1205, y=w1198) -> (x*y=w1202:dbl)
        n782 = property on="Z Step SP" class="DigNum (strict)"() -> ("Maximum"=w1206:dbl)  [unwired: 2 in, 2 out]
        n783 = property on="Z Step SP" class="DigNum (strict)"() -> ("Minimum"=w1207:dbl)  [unwired: 2 in, 2 out]
        n784 = In Range and Coerce(upper limit=w1200, x=w1202, lower limit=w1199) -> (coerced(x)=w1201:dbl)  [unwired: 1 out]
        n785 = To Long Integer(number=w1201) -> (32bit integer=w1203:i32)
        n786 = In Range and Coerce(upper limit=w1206, x=w1209, lower limit=w1207) -> (coerced(x)=w1208:dbl)  [unwired: 1 out]
        n787 = To Long Integer(number=w1208) -> (32bit integer=w1211:i32)
        n788 = property on="Z Scan Velocity SP steps/sec" class="DigNum (strict)"("Val(Sgnl)"=w1203) -> ()  [unwired: 2 in, 2 out]
        n789 = property on="Z Scan Length SP steps" class="DigNum (strict)"("Val(Sgnl)"=w1211) -> ()  [unwired: 2 in, 2 out]
      }
      event "R Scan set": Mouse Down {
        n790 = event-data() -> ()  [unwired: 1 in, 7 out]
        n791 = property on="R steps/rev" class="DigNum (strict)"() -> ("Value"=w1230:u32)  [unwired: 2 in, 2 out]
        n792 = To Double Precision Float(number=w1230) -> (double precision float=w1216:dbl)
        n793 = property on="R Velocity SP step/sec" class="DigNum (strict)"() -> ("Maximum"=w1218:dbl)  [unwired: 2 in, 2 out]
        n794 = property on="R Scan Length SP deg" class="DigNum (strict)"() -> ("Value"=w1228:dbl)  [unwired: 2 in, 2 out]
        n795 = property on="R deg/rev" class="DigNum (strict)"() -> ("Value"=w1215:dbl)  [unwired: 2 in, 2 out]
        n796 = property on="R Scan Velocity SP steps/sec" class="DigNum (strict)"() -> ("Minimum"=w1217:dbl)  [unwired: 2 in, 2 out]
        n797 = property on="R Scan Velocity SP deg/sec" class="DigNum (strict)"() -> ("Value"=w1222:dbl)  [unwired: 2 in, 2 out]
        n798 = Divide(x=w1228, y=w1215) -> (x/y=w1231:dbl)
        n799 = Multiply(x=w1231, y=w1216) -> (x*y=w1227:dbl)
        n800 = Divide(x=w1222, y=w1215) -> (x/y=w1223:dbl)
        n801 = property on="R Step SP" class="DigNum (strict)"() -> ("Maximum"=w1224:dbl)  [unwired: 2 in, 2 out]
        n802 = property on="R Step SP" class="DigNum (strict)"() -> ("Minimum"=w1225:dbl)  [unwired: 2 in, 2 out]
        n803 = Multiply(x=w1223, y=w1216) -> (x*y=w1220:dbl)
        n804 = Absolute Value(x=w1220) -> (abs(x)=w1214:dbl)
        n805 = In Range and Coerce(upper limit=w1224, x=w1227, lower limit=w1225) -> (coerced(x)=w1226:dbl)  [unwired: 1 out]
        n806 = To Long Integer(number=w1226) -> (32bit integer=w1229:i32)
        n807 = In Range and Coerce(upper limit=w1218, x=w1214, lower limit=w1217) -> (coerced(x)=w1219:dbl)  [unwired: 1 out]
        n808 = To Long Integer(number=w1219) -> (32bit integer=w1221:i32)
        n809 = property on="R Scan Length SP steps" class="DigNum (strict)"("Val(Sgnl)"=w1229) -> ()  [unwired: 2 in, 2 out]
        n810 = property on="R Scan Velocity SP steps/sec" class="DigNum (strict)"("Val(Sgnl)"=w1221) -> ()  [unwired: 2 in, 2 out]
      }
      event "Y Go": Mouse Up {
        n811 = event-data() -> ()  [unwired: 1 in, 7 out]
        n812 = flat-sequence {
          tunnel: w1238 -> [w1248]
          tunnel: w1239 -> [w1249]
          tunnel: [w1249] -> w1235
          tunnel: [w1248] -> w1234
          tunnel: [w1252] -> w1237
          tunnel: [w1251] -> w1236
          tunnel: w1235 -> [w1254]
          tunnel: w1234 -> [w1253]
          tunnel: [w1275] -> w1241
          tunnel: [w1270] -> w1240
          tunnel: w1237 -> [w1274]
          tunnel: w1236 -> [w1273]
          tunnel: [w1269] -> w1233
          tunnel: [w1286] -> w1243
          tunnel: [w1281] -> w1242
          tunnel: w1241 -> [w1284]
          tunnel: w1240 -> [w1285]
          tunnel: w1233 -> [w1282]
          tunnel: [w1282] -> w1232
          tunnel: [w1289] -> w1244
          tunnel: [w1292] -> w1245
          tunnel: w1243 -> [w1291]
          tunnel: w1242 -> [w1290]
          tunnel: w1232 -> [w1293]
          frame #0 {
            n813 = property on="Scan Go" class="Bool"("DisabledEnum"=T2."Disabled and Grayed Out" ("Disabled")) -> ()  [unwired: 2 in, 2 out]
            n814 = property on="Y Go" class="Bool"("DisabledEnum"=T2."Disabled and Grayed Out" ("Disabled")) -> ()  [unwired: 2 in, 2 out]
          }
          frame #1 {
            n815 = property on="Y Step SP" class="DigNum (strict)"() -> ("Value"=w1262:i32)  [unwired: 2 in, 2 out]
            n816 = property on="Y Step PV" class="DigNum (strict)"() -> ("Value"=w1261:i32)  [unwired: 2 in, 2 out]
            n817 = property on="Y Backlash" class="DigNum (strict)"() -> ("Value"=w1250:i32)  [unwired: 2 in, 2 out]
            n818 = Subtract(x=w1262, y=w1261) -> (x-y=w1260:i32)
            n819 = Sign(1:w1250) -> (0:w1258:i32)
            n820 = Sign(1:w1260) -> (0:w1259:i32)
            n821 = Multiply(x=w1259, y=w1258) -> (x*y=w1257:i32)
            n822 = Equal?(x=w1257, y=1) -> (x = y?=w1255:bool)
            n823 = case shown="False" w1255 {
              tunnel: w1254 -> [w1265 w1267]
              tunnel: w1253 -> [w1264 w1266]
              tunnel: [w1264 w1266] -> w1252
              tunnel: [w1265 w1267] -> w1251
              frame False {
                n824 = property on="Y Backlash corr" class="Bool (strict)"("Val(Sgnl)"=FALSE ("Value (Signaling)")) -> ()  [unwired: 2 in, 2 out]
              }
              frame True {
                n825 = property on="Y Backlash corr" class="Bool (strict)"("Val(Sgnl)"=TRUE ("Value (Signaling)")) -> ()  [unwired: 2 in, 2 out]
              }
            }
          }
          frame #2 {
            w1269 = 0.1 ("Delay Time (s)")
            # "Velocity Setting"
            n826 = property on="Y Velocity SP step/sec" class="DigNum (strict)"() -> ("Value"=w1278:i32)  [unwired: 2 in, 2 out]
            n827 = Number To Decimal String(number=w1278) -> ()  [unwired: 1 in, 1 out]
            n828 = property on="Y steps/rev" class="DigNum (strict)"() -> ("Value"=w1277:u32)  [unwired: 2 in, 2 out]
            n829 = Divide(x=w1278, y=w1277) -> (x/y=w1279:dbl)
            n830 = Number To Fractional String(number=w1279) -> (F-format string=w1272:string)  [unwired: 3 in]
            n831 = call "Applied Send Command.vi"("error in (no error)"=w1274, "Extra"=w1272, "Command"=T1."Velocity Setting", "VISA resource name"=w1273) -> ("error out"=w1271:errorcluster, "VISA resource name out"=w1275:refnum<visa-resource-name>)  [unwired: 3 in, 1 out]
            n832 = call "Time Delay22"("error in (no error)"=w1271, "Delay Time (s)"=w1269) -> ("error out"=w1270:errorcluster)  [unwired: 9 in]
          }
          frame #3 {
            # "Move to Abs Position"
            n833 = property on="Y Step SP" class="DigNum (strict)"() -> ("Value"=w1288:i32)  [unwired: 2 in, 2 out]
            n834 = Number To Decimal String(number=w1288) -> (decimal integer string=w1283:string)  [unwired: 1 in]
            n835 = call "Applied Send Command.vi"("error in (no error)"=w1285, "Extra"=w1283, "Command"=T1."Distance or Position", "VISA resource name"=w1284) -> ("error out"=w1280:errorcluster, "VISA resource name out"=w1286:refnum<visa-resource-name>)  [unwired: 3 in, 1 out]
            n836 = call "Time Delay"("error in (no error)"=w1280, "Delay Time (s)"=w1282) -> ("error out"=w1281:errorcluster)  [unwired: 9 in]
          }
          frame #4 {
            n837 = call "Applied Send Command.vi"("error in (no error)"=w1290, "Command"=T1."Feed to Position", "VISA resource name"=w1291) -> ("error out"=w1294:errorcluster, "VISA resource name out"=w1292:refnum<visa-resource-name>)  [unwired: 4 in, 1 out]
            n838 = call "Time Delay23"("error in (no error)"=w1294, "Delay Time (s)"=w1293) -> ("error out"=w1289:errorcluster)  [unwired: 9 in]
          }
        }
      }
      event "Z Go": Mouse Up {
        n839 = event-data() -> ()  [unwired: 1 in, 7 out]
        n840 = flat-sequence {
          tunnel: w1300 -> [w1312]
          tunnel: w1301 -> [w1313]
          tunnel: [w1313] -> w1303
          tunnel: [w1312] -> w1302
          tunnel: [w1316] -> w1305
          tunnel: [w1315] -> w1304
          tunnel: w1303 -> [w1318]
          tunnel: w1302 -> [w1317]
          tunnel: [w1336] -> w1307
          tunnel: [w1334] -> w1306
          tunnel: w1305 -> [w1337]
          tunnel: w1304 -> [w1338]
          tunnel: [w1333] -> w1297
          tunnel: [w1347] -> w1309
          tunnel: [w1346] -> w1308
          tunnel: w1307 -> [w1348]
          tunnel: w1306 -> [w1350]
          tunnel: w1297 -> [w1344]
          tunnel: [w1344] -> w1296
          tunnel: [w1359] -> w1299
          tunnel: [w1355] -> w1298
          tunnel: w1309 -> [w1356]
          tunnel: w1308 -> [w1353]
          tunnel: w1296 -> [w1358]
          frame #0 {
            n841 = property on="Scan Go" class="Bool"("DisabledEnum"=T2."Disabled and Grayed Out" ("Disabled")) -> ()  [unwired: 2 in, 2 out]
            n842 = property on="Z Go" class="Bool"("DisabledEnum"=T2."Disabled and Grayed Out" ("Disabled")) -> ()  [unwired: 2 in, 2 out]
          }
          frame #1 {
            n843 = property on="Z Step SP" class="DigNum (strict)"() -> ("Value"=w1326:i32)  [unwired: 2 in, 2 out]
            n844 = property on="Z Step PV" class="DigNum (strict)"() -> ("Value"=w1325:i32)  [unwired: 2 in, 2 out]
            n845 = property on="Z Backlash" class="DigNum (strict)"() -> ("Value"=w1314:i32)  [unwired: 2 in, 2 out]
            n846 = Subtract(x=w1326, y=w1325) -> (x-y=w1324:i32)
            n847 = Sign(1:w1314) -> (0:w1322:i32)
            n848 = Sign(1:w1324) -> (0:w1323:i32)
            n849 = Multiply(x=w1323, y=w1322) -> (x*y=w1321:i32)
            n850 = Equal?(x=w1321, y=1) -> (x = y?=w1319:bool)
            n851 = case shown="True" w1319 {
              tunnel: w1318 -> [w1329 w1331]
              tunnel: w1317 -> [w1328 w1330]
              tunnel: [w1328 w1330] -> w1316
              tunnel: [w1329 w1331] -> w1315
              frame False {
                n852 = property on="Z Backlash corr" class="Bool (strict)"("Val(Sgnl)"=FALSE ("Value (Signaling)")) -> ()  [unwired: 2 in, 2 out]
              }
              frame True {
                n853 = property on="Z Backlash corr" class="Bool (strict)"("Val(Sgnl)"=TRUE ("Value (Signaling)")) -> ()  [unwired: 2 in, 2 out]
              }
            }
          }
          frame #2 {
            w1333 = 0.1 ("Delay Time (s)")
            n854 = property on="Z Velocity SP step/sec" class="DigNum (strict)"() -> ("Value"=w1340:i32)  [unwired: 2 in, 2 out]
            n855 = property on="Z steps/rev" class="DigNum (strict)"() -> ("Value"=w1339:u32)  [unwired: 2 in, 2 out]
            n856 = Divide(x=w1340, y=w1339) -> (x/y=w1341:dbl)
            n857 = Number To Fractional String(number=w1341) -> (F-format string=w1342:string)  [unwired: 3 in]
            n858 = call "Applied Send Command.vi"("error in (no error)"=w1337, "Extra"=w1342, "Command"=T1."Velocity Setting", "VISA resource name"=w1338) -> ("error out"=w1335:errorcluster, "VISA resource name out"=w1336:refnum<visa-resource-name>)  [unwired: 3 in, 1 out]
            n859 = call "Time Delay52"("error in (no error)"=w1335, "Delay Time (s)"=w1333) -> ("error out"=w1334:errorcluster)  [unwired: 9 in]
          }
          frame #3 {
            # "Move to Abs Position"
            n860 = property on="Z Step SP" class="DigNum (strict)"() -> ("Value"=w1352:i32)  [unwired: 2 in, 2 out]
            n861 = Number To Decimal String(number=w1352) -> (decimal integer string=w1349:string)  [unwired: 1 in]
            n862 = call "Applied Send Command.vi"("error in (no error)"=w1350, "Extra"=w1349, "Command"=T1."Distance or Position", "VISA resource name"=w1348) -> ("error out"=w1345:errorcluster, "VISA resource name out"=w1347:refnum<visa-resource-name>)  [unwired: 3 in, 1 out]
            n863 = call "Time Delay51"("error in (no error)"=w1345, "Delay Time (s)"=w1344) -> ("error out"=w1346:errorcluster)  [unwired: 9 in]
          }
          frame #4 {
            n864 = call "Applied Send Command.vi"("error in (no error)"=w1353, "Command"=T1."Feed to Position", "VISA resource name"=w1356) -> ("error out"=w1354:errorcluster, "VISA resource name out"=w1355:refnum<visa-resource-name>)  [unwired: 4 in, 1 out]
            n865 = call "Time Delay28"("error in (no error)"=w1354, "Delay Time (s)"=w1358) -> ("error out"=w1359:errorcluster)  [unwired: 9 in]
          }
        }
      }
      event "R Go": Mouse Up {
        n866 = event-data() -> ()  [unwired: 1 in, 7 out]
        n867 = flat-sequence {
          tunnel: w1364 -> [w1376]
          tunnel: w1365 -> [w1377]
          tunnel: [w1377] -> w1367
          tunnel: [w1376] -> w1366
          tunnel: [w1380] -> w1369
          tunnel: [w1379] -> w1368
          tunnel: w1367 -> [w1382]
          tunnel: w1366 -> [w1381]
          tunnel: [w1398] -> w1371
          tunnel: [w1399] -> w1370
          tunnel: w1369 -> [w1400]
          tunnel: w1368 -> [w1401]
          tunnel: [w1397] -> w1361
          tunnel: [w1411] -> w1373
          tunnel: [w1409] -> w1372
          tunnel: w1371 -> [w1410]
          tunnel: w1370 -> [w1412]
          tunnel: w1361 -> [w1407]
          tunnel: [w1407] -> w1360
          tunnel: [w1422] -> w1363
          tunnel: [w1418] -> w1362
          tunnel: w1373 -> [w1419]
          tunnel: w1372 -> [w1416]
          tunnel: w1360 -> [w1421]
          frame #0 {
            n868 = property on="Scan Go" class="Bool"("DisabledEnum"=T2."Disabled and Grayed Out" ("Disabled")) -> ()  [unwired: 2 in, 2 out]
            n869 = property on="R Go" class="Bool"("DisabledEnum"=T2."Disabled and Grayed Out" ("Disabled")) -> ()  [unwired: 2 in, 2 out]
          }
          frame #1 {
            n870 = property on="R Step SP" class="DigNum (strict)"() -> ("Value"=w1390:i32)  [unwired: 2 in, 2 out]
            n871 = property on="R Step PV" class="DigNum (strict)"() -> ("Value"=w1389:i32)  [unwired: 2 in, 2 out]
            n872 = property on="R Backlash" class="DigNum (strict)"() -> ("Value"=w1378:i32)  [unwired: 2 in, 2 out]
            n873 = Subtract(x=w1390, y=w1389) -> (x-y=w1388:i32)
            n874 = Sign(1:w1378) -> (0:w1386:i32)
            n875 = Sign(1:w1388) -> (0:w1387:i32)
            n876 = Multiply(x=w1387, y=w1386) -> (x*y=w1385:i32)
            n877 = Equal?(x=w1385, y=1) -> (x = y?=w1383:bool)
            n878 = case shown="True" w1383 {
              tunnel: w1382 -> [w1393 w1395]
              tunnel: w1381 -> [w1392 w1394]
              tunnel: [w1392 w1394] -> w1380
              tunnel: [w1393 w1395] -> w1379
              frame False {
                n879 = property on="R Backlash corr" class="Bool (strict)"("Val(Sgnl)"=FALSE ("Value (Signaling)")) -> ()  [unwired: 2 in, 2 out]
              }
              frame True {
                n880 = property on="R Backlash corr" class="Bool (strict)"("Val(Sgnl)"=TRUE ("Value (Signaling)")) -> ()  [unwired: 2 in, 2 out]
              }
            }
          }
          frame #2 {
            w1397 = 0.1 ("Delay Time (s)")
            # "Velocity Setting"
            n881 = property on="R Velocity SP step/sec" class="DigNum (strict)"() -> ("Value"=w1403:i32)  [unwired: 2 in, 2 out]
            n882 = property on="R steps/rev" class="DigNum (strict)"() -> ("Value"=w1402:u32)  [unwired: 2 in, 2 out]
            n883 = Divide(x=w1403, y=w1402) -> (x/y=w1404:dbl)
            n884 = Number To Fractional String(number=w1404) -> (F-format string=w1405:string)  [unwired: 3 in]
            n885 = call "Applied Send Command.vi"("error in (no error)"=w1400, "Extra"=w1405, "VISA resource name"=w1401) -> ("error out"=w1406:errorcluster, "VISA resource name out"=w1398:refnum<visa-resource-name>)  [unwired: 4 in, 1 out]
            n886 = call "Time Delay54"("error in (no error)"=w1406, "Delay Time (s)"=w1397) -> ("error out"=w1399:errorcluster)  [unwired: 9 in]
          }
          frame #3 {
            # "Distance/Position"
            n887 = property on="R Step SP" class="DigNum (strict)"() -> ("Value"=w1413:i32)  [unwired: 2 in, 2 out]
            n888 = Number To Decimal String(number=w1413) -> (decimal integer string=w1414:string)  [unwired: 1 in]
            n889 = call "Applied Send Command.vi"("error in (no error)"=w1412, "Extra"=w1414, "Command"=T1."Distance or Position", "VISA resource name"=w1410) -> ("error out"=w1408:errorcluster, "VISA resource name out"=w1411:refnum<visa-resource-name>)  [unwired: 3 in, 1 out]
            n890 = call "Time Delay53"("error in (no error)"=w1408, "Delay Time (s)"=w1407) -> ("error out"=w1409:errorcluster)  [unwired: 9 in]
          }
          frame #4 {
            # "Feed to Position"
            n891 = call "Applied Send Command.vi"("error in (no error)"=w1416, "Command"=T1."Feed to Position", "VISA resource name"=w1419) -> ("error out"=w1417:errorcluster, "VISA resource name out"=w1418:refnum<visa-resource-name>)  [unwired: 4 in, 1 out]
            n892 = call "Time Delay29"("error in (no error)"=w1417, "Delay Time (s)"=w1421) -> ("error out"=w1422:errorcluster)  [unwired: 9 in]
          }
        }
      }
      event "X Go": Mouse Up {
        n893 = event-data() -> ()  [unwired: 1 in, 7 out]
        n894 = flat-sequence {
          tunnel: [w1438] -> w1434
          tunnel: [w1437] -> w1433
          tunnel: w1432 -> [w1438]
          tunnel: w1431 -> [w1437]
          tunnel: [w1443] -> w1436
          tunnel: [w1442] -> w1435
          tunnel: w1434 -> [w1445]
          tunnel: w1433 -> [w1444]
          tunnel: [w1464] -> w1428
          tunnel: [w1461] -> w1426
          tunnel: w1436 -> [w1465]
          tunnel: w1435 -> [w1466]
          tunnel: [w1460] -> w1424
          tunnel: w1428 -> [w1473]
          tunnel: [w1472] -> w1427
          tunnel: w1426 -> [w1474]
          tunnel: [w1475] -> w1425
          tunnel: w1424 -> [w1471]
          tunnel: [w1471] -> w1423
          tunnel: w1427 -> [w1485]
          tunnel: w1425 -> [w1484]
          tunnel: [w1483] -> w1430
          tunnel: [w1482] -> w1429
          tunnel: w1423 -> [w1480]
          frame #0 {
            n895 = property on="Scan Go" class="Bool"("DisabledEnum"=T2."Disabled and Grayed Out" ("Disabled")) -> ()  [unwired: 2 in, 2 out]
            n896 = property on="X Go" class="Bool"("DisabledEnum"=T2."Disabled and Grayed Out" ("Disabled")) -> ()  [unwired: 2 in, 2 out]
          }
          frame #1 {
            n897 = property on="X Step SP" class="DigNum (strict)"() -> ("Value"=w1453:i32)  [unwired: 2 in, 2 out]
            n898 = property on="X Step PV" class="DigNum (strict)"() -> ("Value"=w1452:i32)  [unwired: 2 in, 2 out]
            n899 = property on="X Backlash" class="DigNum (strict)"() -> ("Value"=w1441:i32)  [unwired: 2 in, 2 out]
            n900 = Subtract(x=w1453, y=w1452) -> (x-y=w1451:i32)
            n901 = Sign(1:w1441) -> (0:w1449:i32)
            n902 = Sign(1:w1451) -> (0:w1450:i32)
            n903 = Multiply(x=w1450, y=w1449) -> (x*y=w1448:i32)
            n904 = Equal?(x=w1448, y=1) -> (x = y?=w1446:bool)
            n905 = case shown="True" w1446 {
              tunnel: w1445 -> [w1456 w1458]
              tunnel: w1444 -> [w1455 w1457]
              tunnel: [w1455 w1457] -> w1443
              tunnel: [w1456 w1458] -> w1442
              frame False {
                n906 = property on="X Backlash corr" class="Bool (strict)"("Val(Sgnl)"=FALSE ("Value (Signaling)")) -> ()  [unwired: 2 in, 2 out]
              }
              frame True {
                n907 = property on="X Backlash corr" class="Bool (strict)"("Val(Sgnl)"=TRUE ("Value (Signaling)")) -> ()  [unwired: 2 in, 2 out]
              }
            }
          }
          frame #2 {
            w1460 = 0.1 ("Delay Time (s)")
            n908 = property on="X Velocity SP step/sec" class="DigNum (strict)"() -> ("Value"=w1463:i32)  [unwired: 2 in, 2 out]
            n909 = property on="X steps/rev" class="DigNum (strict)"() -> ("Value"=w1467:u32)  [unwired: 2 in, 2 out]
            n910 = Divide(x=w1463, y=w1467) -> (x/y=w1468:dbl)
            n911 = Number To Fractional String(number=w1468) -> (F-format string=w1469:string)  [unwired: 3 in]
            n912 = call "Applied Send Command.vi"("error in (no error)"=w1465, "Extra"=w1469, "Command"=T1."Velocity Setting", "VISA resource name"=w1466) -> ("error out"=w1462:errorcluster, "VISA resource name out"=w1464:refnum<visa-resource-name>)  [unwired: 3 in, 1 out]
            n913 = call "Time Delay14"("error in (no error)"=w1462, "Delay Time (s)"=w1460) -> ("error out"=w1461:errorcluster)  [unwired: 9 in]
          }
          frame #3 {
            # "Distance/Position"
            n914 = property on="X Step SP" class="DigNum (strict)"() -> ("Value"=w1476:i32)  [unwired: 2 in, 2 out]
            n915 = Number To Decimal String(number=w1476) -> (decimal integer string=w1478:string)  [unwired: 1 in]
            n916 = call "Applied Send Command.vi"("error in (no error)"=w1474, "Extra"=w1478, "Command"=T1."Distance or Position", "VISA resource name"=w1473) -> ("error out"=w1477:errorcluster, "VISA resource name out"=w1472:refnum<visa-resource-name>)  [unwired: 3 in, 1 out]
            n917 = call "Time Delay31"("error in (no error)"=w1477, "Delay Time (s)"=w1471) -> ("error out"=w1475:errorcluster)  [unwired: 9 in]
          }
          frame #4 {
            # "Feed to Position"
            n918 = call "Applied Send Command.vi"("error in (no error)"=w1484, "Command"=T1."Feed to Position", "VISA resource name"=w1485) -> ("error out"=w1481:errorcluster, "VISA resource name out"=w1483:refnum<visa-resource-name>)  [unwired: 4 in, 1 out]
            n919 = call "Time Delay15"("error in (no error)"=w1481, "Delay Time (s)"=w1480) -> ("error out"=w1482:errorcluster)  [unwired: 9 in]
          }
        }
      }
      event "X Scan OK": Mouse Up {
        n920 = event-data() -> ()  [unwired: 1 in, 7 out]
        n921 = flat-sequence {
          tunnel: [w1502] -> w1494
          tunnel: [w1513] -> w1493
          tunnel: w1492 -> [w1510]
          tunnel: w1491 -> [w1509]
          tunnel: w1494 -> [w1520]
          tunnel: w1493 -> [w1519]
          tunnel: [w1520] -> w1488
          tunnel: [w1519] -> w1487
          tunnel: [w1522] -> w1489
          tunnel: [w1523] -> w1490
          tunnel: w1488 -> [w1523]
          tunnel: w1487 -> [w1522]
          frame #0 {
            # "VELOCITY"
            n922 = property on="X steps/rev" class="DigNum (strict)"() -> ("Value"=w1495:u32)  [unwired: 2 in, 2 out]
            n923 = property on="X Scan Velocity SP steps/sec" class="DigNum (strict)"() -> ("Value"=w1496:i32)  [unwired: 2 in, 2 out]
            n924 = Divide(x=w1496, y=w1495) -> (x/y=w1497:dbl)
            n925 = Number To Fractional String(number=w1497) -> (F-format string=w1511:string)  [unwired: 3 in]
            n926 = call "Applied Send Command.vi"("error in (no error)"=w1509, "Extra"=w1511, "Command"=T1."Velocity Setting", "VISA resource name"=w1510) -> ("error out"=w1498:errorcluster, "VISA resource name out"=w1499:refnum<visa-resource-name>)  [unwired: 3 in, 1 out]
            n927 = call "Time Delay9"("error in (no error)"=w1498) -> ("error out"=w1500:errorcluster)  [unwired: 10 in]
            n928 = call "Applied Send Command.vi"("error in (no error)"=w1500, "Extra"="", "Command"=T1."Velocity Setting", "VISA resource name"=w1499) -> ("error out"=w1501:errorcluster, "read buffer"=w1506:string, "VISA resource name out"=w1502:refnum<visa-resource-name>)  [unwired: 3 in]
            n929 = call "Time Delay10"("error in (no error)"=w1501) -> ("error out"=w1513:errorcluster)  [unwired: 10 in]
            n930 = Fract/Exp String To Number(string=w1506, offset=3) -> (number=w1504:dbl)  [unwired: 2 in, 1 out]
            n931 = Multiply(x=w1504, y=w1495) -> (x*y=w1503:dbl)
            n932 = property on="X velocity PV step/sec" class="DigNum (strict)"("Val(Sgnl)"=w1503) -> ()  [unwired: 2 in, 2 out]
          }
          frame #1 {
            n933 = property on="X Scan" class="Bool (strict)"("Val(Sgnl)"=TRUE ("Slew Ready 2")) -> ()  [unwired: 2 in, 2 out]
            n934 = property on="Scan Cancel" class="Bool"("DisabledEnum"=T2."Enabled" ("Disabled")) -> ()  [unwired: 2 in, 2 out]
            n935 = property on="Scan Go" class="Bool"("DisabledEnum"=T2."Enabled" ("Disabled")) -> ()  [unwired: 2 in, 2 out]
            n936 = property on="X Scan Length SP steps" class="DigNum (strict)"("DisabledEnum"=T2."Disabled and Grayed Out" ("Disabled")) -> ()  [unwired: 2 in, 2 out]
            n937 = property on="X Scan Velocity SP steps/sec" class="DigNum (strict)"("DisabledEnum"=T2."Disabled and Grayed Out" ("Disabled")) -> ()  [unwired: 2 in, 2 out]
          }
          frame #2 {
            n938 = property on="X Go" class="Bool"("DisabledEnum"=T2."Disabled and Grayed Out" ("Disabled")) -> ()  [unwired: 2 in, 2 out]
          }
        }
      }
      event "Y Scan OK": Mouse Up {
        n939 = event-data() -> ()  [unwired: 1 in, 7 out]
        n940 = flat-sequence {
          tunnel: w1531 -> [w1543]
          tunnel: w1530 -> [w1544]
          tunnel: [w1534] -> w1528
          tunnel: [w1550] -> w1527
          tunnel: w1528 -> [w1557]
          tunnel: w1527 -> [w1556]
          tunnel: [w1557] -> w1525
          tunnel: [w1556] -> w1524
          tunnel: [w1559] -> w1529
          tunnel: [w1560] -> w1526
          tunnel: w1525 -> [w1560]
          tunnel: w1524 -> [w1559]
          frame #0 {
            # "VELOCITY"
            n941 = property on="Y Scan Velocity SP steps/sec" class="DigNum (strict)"() -> ("Value"=w1546:i32)  [unwired: 2 in, 2 out]
            n942 = property on="Y steps/rev" class="DigNum (strict)"() -> ("Value"=w1537:u32)  [unwired: 2 in, 2 out]
            n943 = Divide(x=w1546, y=w1537) -> (x/y=w1547:dbl)
            n944 = Number To Fractional String(number=w1547) -> (F-format string=w1548:string)  [unwired: 3 in]
            n945 = call "Applied Send Command.vi"("error in (no error)"=w1543, "Extra"=w1548, "Command"=T1."Velocity Setting", "VISA resource name"=w1544) -> ("error out"=w1545:errorcluster, "VISA resource name out"=w1535:refnum<visa-resource-name>)  [unwired: 3 in, 1 out]
            n946 = call "Time Delay5"("error in (no error)"=w1545) -> ("error out"=w1536:errorcluster)  [unwired: 10 in]
            n947 = call "Applied Send Command.vi"("error in (no error)"=w1536, "Extra"="", "Command"=T1."Velocity Setting", "VISA resource name"=w1535) -> ("error out"=w1533:errorcluster, "read buffer"=w1540:string, "VISA resource name out"=w1534:refnum<visa-resource-name>)  [unwired: 3 in]
            n948 = Fract/Exp String To Number(string=w1540, offset=3) -> (number=w1539:dbl)  [unwired: 2 in, 1 out]
            n949 = call "Time Delay6"("error in (no error)"=w1533) -> ("error out"=w1550:errorcluster)  [unwired: 10 in]
            n950 = Multiply(x=w1539, y=w1537) -> (x*y=w1538:dbl)
            n951 = property on="Y velocity PV step/sec" class="DigNum (strict)"("Val(Sgnl)"=w1538) -> ()  [unwired: 2 in, 2 out]
          }
          frame #1 {
            n952 = property on="Y Scan" class="Bool (strict)"("Val(Sgnl)"=TRUE ("Slew Ready 2")) -> ()  [unwired: 2 in, 2 out]
            n953 = property on="Scan Cancel" class="Bool"("DisabledEnum"=T2."Enabled" ("Disabled")) -> ()  [unwired: 2 in, 2 out]
            n954 = property on="Scan Go" class="Bool"("DisabledEnum"=T2."Enabled" ("Disabled")) -> ()  [unwired: 2 in, 2 out]
            n955 = property on="Y Scan Length SP steps" class="DigNum (strict)"("DisabledEnum"=T2."Disabled and Grayed Out" ("Disabled")) -> ()  [unwired: 2 in, 2 out]
            n956 = property on="Y Scan Velocity SP steps/sec" class="DigNum (strict)"("DisabledEnum"=T2."Disabled and Grayed Out" ("Disabled")) -> ()  [unwired: 2 in, 2 out]
          }
          frame #2 {
            n957 = property on="Y Go" class="Bool"("DisabledEnum"=T2."Disabled and Grayed Out" ("Disabled")) -> ()  [unwired: 2 in, 2 out]
          }
        }
      }
      event "Z Scan OK": Mouse Up {
        n958 = event-data() -> ()  [unwired: 1 in, 7 out]
        n959 = flat-sequence {
          tunnel: [w1573] -> w1568
          tunnel: [w1587] -> w1567
          tunnel: w1564 -> [w1569]
          tunnel: w1563 -> [w1570]
          tunnel: w1568 -> [w1594]
          tunnel: w1567 -> [w1593]
          tunnel: [w1594] -> w1566
          tunnel: [w1593] -> w1565
          tunnel: [w1596] -> w1562
          tunnel: [w1597] -> w1561
          tunnel: w1566 -> [w1597]
          tunnel: w1565 -> [w1596]
          frame #0 {
            # "VELOCITY"
            n960 = property on="Z Scan Velocity SP steps/sec" class="DigNum (strict)"() -> ("Value"=w1583:i32)  [unwired: 2 in, 2 out]
            n961 = property on="Z steps/rev" class="DigNum (strict)"() -> ("Value"=w1576:u32)  [unwired: 2 in, 2 out]
            n962 = Divide(x=w1583, y=w1576) -> (x/y=w1584:dbl)
            n963 = Number To Fractional String(number=w1584) -> (F-format string=w1585:string)  [unwired: 3 in]
            n964 = call "Applied Send Command.vi"("error in (no error)"=w1570, "Extra"=w1585, "Command"=T1."Velocity Setting", "VISA resource name"=w1569) -> ("error out"=w1582:errorcluster, "VISA resource name out"=w1572:refnum<visa-resource-name>)  [unwired: 3 in, 1 out]
            n965 = call "Time Delay24"("error in (no error)"=w1582) -> ("error out"=w1571:errorcluster)  [unwired: 10 in]
            n966 = call "Applied Send Command.vi"("error in (no error)"=w1571, "Extra"="", "Command"=T1."Velocity Setting", "VISA resource name"=w1572) -> ("error out"=w1574:errorcluster, "read buffer"=w1579:string, "VISA resource name out"=w1573:refnum<visa-resource-name>)  [unwired: 3 in]
            n967 = call "Time Delay25"("error in (no error)"=w1574) -> ("error out"=w1587:errorcluster)  [unwired: 10 in]
            n968 = Fract/Exp String To Number(string=w1579, offset=3) -> (number=w1578:dbl)  [unwired: 2 in, 1 out]
            n969 = Multiply(x=w1578, y=w1576) -> (x*y=w1575:dbl)
            n970 = property on="Z  velocity PV step/sec" class="DigNum (strict)"("Val(Sgnl)"=w1575) -> ()  [unwired: 2 in, 2 out]
          }
          frame #1 {
            n971 = property on="Z Scan" class="Bool (strict)"("Val(Sgnl)"=TRUE ("Slew Ready 2")) -> ()  [unwired: 2 in, 2 out]
            n972 = property on="Scan Cancel" class="Bool"("DisabledEnum"=T2."Enabled" ("Disabled")) -> ()  [unwired: 2 in, 2 out]
            n973 = property on="Scan Go" class="Bool"("DisabledEnum"=T2."Enabled" ("Disabled")) -> ()  [unwired: 2 in, 2 out]
            n974 = property on="Z Scan Length SP steps" class="DigNum (strict)"("DisabledEnum"=T2."Disabled and Grayed Out" ("Disabled")) -> ()  [unwired: 2 in, 2 out]
            n975 = property on="Z Scan Velocity SP steps/sec" class="DigNum (strict)"("DisabledEnum"=T2."Disabled and Grayed Out" ("Disabled")) -> ()  [unwired: 2 in, 2 out]
          }
          frame #2 {
            n976 = property on="Z Go" class="Bool"("DisabledEnum"=T2."Disabled and Grayed Out" ("Disabled")) -> ()  [unwired: 2 in, 2 out]
          }
        }
      }
      event "R Scan OK": Mouse Up {
        n977 = event-data() -> ()  [unwired: 1 in, 7 out]
        n978 = flat-sequence {
          tunnel: [w1609] -> w1605
          tunnel: [w1624] -> w1604
          tunnel: w1601 -> [w1617]
          tunnel: w1600 -> [w1618]
          tunnel: w1605 -> [w1631]
          tunnel: w1604 -> [w1630]
          tunnel: [w1631] -> w1603
          tunnel: [w1630] -> w1602
          tunnel: [w1633] -> w1598
          tunnel: [w1634] -> w1599
          tunnel: w1603 -> [w1634]
          tunnel: w1602 -> [w1633]
          frame #0 {
            # "VELOCITY"
            n979 = property on="R Scan Velocity SP steps/sec" class="DigNum (strict)"() -> ("Value"=w1619:i32)  [unwired: 2 in, 2 out]
            n980 = property on="R steps/rev" class="DigNum (strict)"() -> ("Value"=w1607:u32)  [unwired: 2 in, 2 out]
            n981 = Divide(x=w1619, y=w1607) -> (x/y=w1621:dbl)
            n982 = Number To Fractional String(number=w1621) -> (F-format string=w1622:string)  [unwired: 3 in]
            n983 = call "Applied Send Command.vi"("error in (no error)"=w1618, "Extra"=w1622, "Command"=T1."Velocity Setting", "VISA resource name"=w1617) -> ("error out"=w1620:errorcluster, "VISA resource name out"=w1611:refnum<visa-resource-name>)  [unwired: 3 in, 1 out]
            n984 = call "Time Delay26"("error in (no error)"=w1620) -> ("error out"=w1610:errorcluster)  [unwired: 10 in]
            n985 = call "Applied Send Command.vi"("error in (no error)"=w1610, "Extra"="", "Command"=T1."Velocity Setting", "VISA resource name"=w1611) -> ("error out"=w1608:errorcluster, "read buffer"=w1614:string, "VISA resource name out"=w1609:refnum<visa-resource-name>)  [unwired: 3 in]
            n986 = call "Time Delay27"("error in (no error)"=w1608) -> ("error out"=w1624:errorcluster)  [unwired: 10 in]
            n987 = Fract/Exp String To Number(string=w1614, offset=3) -> (number=w1613:dbl)  [unwired: 2 in, 1 out]
            n988 = Multiply(x=w1613, y=w1607) -> (x*y=w1606:dbl)
            n989 = property on="R velocity PV step/sec" class="DigNum (strict)"("Val(Sgnl)"=w1606) -> ()  [unwired: 2 in, 2 out]
          }
          frame #1 {
            n990 = property on="R Scan" class="Bool (strict)"("Val(Sgnl)"=TRUE ("Slew Ready 2")) -> ()  [unwired: 2 in, 2 out]
            n991 = property on="Scan Cancel" class="Bool"("DisabledEnum"=T2."Enabled" ("Disabled")) -> ()  [unwired: 2 in, 2 out]
            n992 = property on="Scan Go" class="Bool"("DisabledEnum"=T2."Enabled" ("Disabled")) -> ()  [unwired: 2 in, 2 out]
            n993 = property on="R Scan Length SP steps" class="DigNum (strict)"("DisabledEnum"=T2."Disabled and Grayed Out" ("Disabled")) -> ()  [unwired: 2 in, 2 out]
            n994 = property on="R Scan Velocity SP steps/sec" class="DigNum (strict)"("DisabledEnum"=T2."Disabled and Grayed Out" ("Disabled")) -> ()  [unwired: 2 in, 2 out]
          }
          frame #2 {
            n995 = property on="R Go" class="Bool"("DisabledEnum"=T2."Disabled and Grayed Out" ("Disabled")) -> ()  [unwired: 2 in, 2 out]
          }
        }
      }
      event Application Instance Close? {
        n996 = event-data() -> ()  [unwired: 1 in, 4 out]
        n997 = event-data() -> ()  [unwired: 3 in, 1 out]
      }
      event "Stop": Mouse Down {
        n998 = event-data() -> ()  [unwired: 1 in, 7 out]
        n999 = flat-sequence {
          tunnel: [w1665] -> w1648
          tunnel: [w1664] -> w1647
          tunnel: w1646 -> [w1666]
          tunnel: w1645 -> [w1663]
          frame #0 {
            n1000 = call "Applied Send Command.vi"("error in (no error)"=w1663, "Command"=T1."Stop", "VISA resource name"=w1666) -> ("error out"=w1664:errorcluster, "VISA resource name out"=w1665:refnum<visa-resource-name>)  [unwired: 4 in, 1 out]
          }
        }
        n1001 = flat-sequence {
          tunnel: w1652 -> [w1669]
          tunnel: w1651 -> [w1668]
          tunnel: [w1670] -> w1650
          tunnel: [w1671] -> w1649
          frame #0 {
            n1002 = call "Applied Send Command.vi"("error in (no error)"=w1668, "Command"=T1."Stop", "VISA resource name"=w1669) -> ("error out"=w1671:errorcluster, "VISA resource name out"=w1670:refnum<visa-resource-name>)  [unwired: 4 in, 1 out]
          }
        }
        n1003 = flat-sequence {
          tunnel: [w1660] -> w1642
          tunnel: [w1661] -> w1641
          tunnel: w1644 -> [w1658]
          tunnel: w1643 -> [w1659]
          frame #0 {
            n1004 = call "Applied Send Command.vi"("error in (no error)"=w1659, "Command"=T1."Stop", "VISA resource name"=w1658) -> ("error out"=w1661:errorcluster, "VISA resource name out"=w1660:refnum<visa-resource-name>)  [unwired: 4 in, 1 out]
          }
        }
        n1005 = flat-sequence {
          tunnel: w1640 -> [w1653]
          tunnel: w1639 -> [w1654]
          tunnel: [w1656] -> w1638
          tunnel: [w1655] -> w1637
          frame #0 {
            n1006 = call "Applied Send Command.vi"("error in (no error)"=w1654, "Command"=T1."Stop", "VISA resource name"=w1653) -> ("error out"=w1655:errorcluster, "VISA resource name out"=w1656:refnum<visa-resource-name>)  [unwired: 4 in, 1 out]
          }
        }
      }
      event "Scan Cancel": Mouse Down {
        n1007 = event-data() -> ()  [unwired: 1 in, 7 out]
        n1008 = flat-sequence {
          tunnel: w1688 -> [w1726]
          tunnel: w1687 -> [w1725]
          tunnel: [w1728] -> w1690
          tunnel: [w1727] -> w1689
          tunnel: [w1736] -> w1685
          tunnel: [w1737] -> w1686
          tunnel: w1690 -> [w1737]
          tunnel: w1689 -> [w1736]
          frame #0 {
            n1009 = call "Applied Send Command.vi"("error in (no error)"=w1725, "Command"=T1."Stop", "VISA resource name"=w1726) -> ("error out"=w1727:errorcluster, "VISA resource name out"=w1728:refnum<visa-resource-name>)  [unwired: 4 in, 1 out]
          }
          frame #1 {
            n1010 = property on="X Scan" class="Bool (strict)"("Value"=FALSE ("Slew Ready")) -> ()  [unwired: 2 in, 2 out]
            n1011 = property on="X Scan set" class="Bool"("DisabledEnum"=T2."Enabled" ("Disabled")) -> ()  [unwired: 2 in, 2 out]
            n1012 = property on="X Scan Velocity SP steps/sec" class="DigNum (strict)"("DisabledEnum"=T2."Enabled" ("Disabled")) -> ()  [unwired: 2 in, 2 out]
            n1013 = property on="X Scan Length SP steps" class="DigNum (strict)"("DisabledEnum"=T2."Enabled" ("Disabled")) -> ()  [unwired: 2 in, 2 out]
            n1014 = property on="X Go" class="Bool"("DisabledEnum"=T2."Enabled" ("Disabled")) -> ()  [unwired: 2 in, 2 out]
            n1015 = property on="X Scan OK" class="Bool"("DisabledEnum"=T2."Enabled" ("Disabled")) -> ()  [unwired: 2 in, 2 out]
          }
        }
        n1016 = flat-sequence {
          tunnel: w1696 -> [w1739]
          tunnel: w1695 -> [w1738]
          tunnel: [w1741] -> w1692
          tunnel: [w1740] -> w1691
          tunnel: [w1749] -> w1697
          tunnel: [w1750] -> w1698
          tunnel: w1692 -> [w1750]
          tunnel: w1691 -> [w1749]
          frame #0 {
            n1017 = call "Applied Send Command.vi"("error in (no error)"=w1738, "Command"=T1."Stop", "VISA resource name"=w1739) -> ("error out"=w1740:errorcluster, "VISA resource name out"=w1741:refnum<visa-resource-name>)  [unwired: 4 in, 1 out]
          }
          frame #1 {
            n1018 = property on="Y Scan" class="Bool (strict)"("Value"=FALSE ("Slew Ready")) -> ()  [unwired: 2 in, 2 out]
            n1019 = property on="Y Go" class="Bool"("DisabledEnum"=T2."Enabled" ("Disabled")) -> ()  [unwired: 2 in, 2 out]
            n1020 = property on="Y Scan Velocity SP steps/sec" class="DigNum (strict)"("DisabledEnum"=T2."Enabled" ("Disabled")) -> ()  [unwired: 2 in, 2 out]
            n1021 = property on="Y Scan set" class="Bool"("DisabledEnum"=T2."Enabled" ("Disabled")) -> ()  [unwired: 2 in, 2 out]
            n1022 = property on="Y Scan OK" class="Bool"("DisabledEnum"=T2."Enabled" ("Disabled")) -> ()  [unwired: 2 in, 2 out]
            n1023 = property on="Y Scan Length SP steps" class="DigNum (strict)"("DisabledEnum"=T2."Enabled" ("Disabled")) -> ()  [unwired: 2 in, 2 out]
          }
        }
        n1024 = flat-sequence {
          tunnel: [w1715] -> w1684
          tunnel: [w1714] -> w1683
          tunnel: w1682 -> [w1713]
          tunnel: w1681 -> [w1712]
          tunnel: [w1723] -> w1679
          tunnel: [w1724] -> w1680
          tunnel: w1684 -> [w1724]
          tunnel: w1683 -> [w1723]
          frame #0 {
            n1025 = call "Applied Send Command.vi"("error in (no error)"=w1712, "Command"=T1."Stop", "VISA resource name"=w1713) -> ("error out"=w1714:errorcluster, "VISA resource name out"=w1715:refnum<visa-resource-name>)  [unwired: 4 in, 1 out]
          }
          frame #1 {
            n1026 = property on="Z Scan" class="Bool (strict)"("Value"=FALSE ("Slew Ready")) -> ()  [unwired: 2 in, 2 out]
            n1027 = property on="Z Scan set" class="Bool"("DisabledEnum"=T2."Enabled" ("Disabled")) -> ()  [unwired: 2 in, 2 out]
            n1028 = property on="Z Scan Velocity SP steps/sec" class="DigNum (strict)"("DisabledEnum"=T2."Enabled" ("Disabled")) -> ()  [unwired: 2 in, 2 out]
            n1029 = property on="Z Scan Length SP steps" class="DigNum (strict)"("DisabledEnum"=T2."Enabled" ("Disabled")) -> ()  [unwired: 2 in, 2 out]
            n1030 = property on="Z Go" class="Bool"("DisabledEnum"=T2."Enabled" ("Disabled")) -> ()  [unwired: 2 in, 2 out]
            n1031 = property on="Z Scan OK" class="Bool"("DisabledEnum"=T2."Enabled" ("Disabled")) -> ()  [unwired: 2 in, 2 out]
          }
        }
        n1032 = flat-sequence {
          tunnel: [w1702] -> w1678
          tunnel: [w1701] -> w1677
          tunnel: w1676 -> [w1699]
          tunnel: w1675 -> [w1700]
          tunnel: [w1710] -> w1673
          tunnel: [w1711] -> w1674
          tunnel: w1678 -> [w1711]
          tunnel: w1677 -> [w1710]
          frame #0 {
            n1033 = call "Applied Send Command.vi"("error in (no error)"=w1700, "Command"=T1."Stop", "VISA resource name"=w1699) -> ("error out"=w1701:errorcluster, "VISA resource name out"=w1702:refnum<visa-resource-name>)  [unwired: 4 in, 1 out]
          }
          frame #1 {
            n1034 = property on="R Scan" class="Bool (strict)"("Value"=FALSE ("Slew Ready")) -> ()  [unwired: 2 in, 2 out]
            n1035 = property on="R Scan Velocity SP steps/sec" class="DigNum (strict)"("DisabledEnum"=T2."Enabled" ("Disabled")) -> ()  [unwired: 2 in, 2 out]
            n1036 = property on="R Go" class="Bool"("DisabledEnum"=T2."Enabled" ("Disabled")) -> ()  [unwired: 2 in, 2 out]
            n1037 = property on="R Scan OK" class="Bool"("DisabledEnum"=T2."Enabled" ("Disabled")) -> ()  [unwired: 2 in, 2 out]
            n1038 = property on="R Scan Length SP steps" class="DigNum (strict)"("DisabledEnum"=T2."Enabled" ("Disabled")) -> ()  [unwired: 2 in, 2 out]
            n1039 = property on="R Scan set" class="Bool"("DisabledEnum"=T2."Enabled" ("Disabled")) -> ()  [unwired: 2 in, 2 out]
          }
        }
        n1040 = property on="Scan Go" class="Bool"("DisabledEnum"=T2."Disabled and Grayed Out" ("Disabled")) -> ()  [unwired: 2 in, 2 out]
        n1041 = property on="Scan Cancel" class="Bool"("DisabledEnum"=T2."Disabled and Grayed Out" ("Disabled")) -> ()  [unwired: 2 in, 2 out]
      }
      event "Scan Go": Mouse Up {
        n1042 = event-data() -> ()  [unwired: 1 in, 7 out]
        n1043 = flat-sequence {
          tunnel: w1786 -> [w1805]
          tunnel: w1785 -> [w1806]
          tunnel: w1784 -> [w1803]
          tunnel: w1783 -> [w1804]
          tunnel: w1782 -> [w1802]
          tunnel: w1781 -> [w1801]
          tunnel: w1780 -> [w1800]
          tunnel: w1779 -> [w1799]
          tunnel: [w1798] -> w1770
          tunnel: [w1797] -> w1768
          tunnel: [w1796] -> w1766
          tunnel: [w1795] -> w1764
          tunnel: [w1794] -> w1762
          tunnel: [w1793] -> w1760
          tunnel: [w1792] -> w1758
          tunnel: [w1791] -> w1756
          tunnel: [w1790] -> w1754
          tunnel: [w1789] -> w1753
          tunnel: [w1788] -> w1752
          tunnel: [w1787] -> w1751
          tunnel: w1770 -> [w1862]
          tunnel: [w1861] -> w1769
          tunnel: w1768 -> [w1860]
          tunnel: [w1859] -> w1767
          tunnel: w1766 -> [w1858]
          tunnel: [w1857] -> w1765
          tunnel: w1764 -> [w1856]
          tunnel: [w1855] -> w1763
          tunnel: w1762 -> [w1854]
          tunnel: [w1853] -> w1761
          tunnel: w1760 -> [w1851]
          tunnel: [w1852] -> w1759
          tunnel: w1758 -> [w1850]
          tunnel: [w1849] -> w1757
          tunnel: w1756 -> [w1848]
          tunnel: [w1847] -> w1755
          tunnel: w1754 -> [w1846]
          tunnel: w1753 -> [w1845]
          tunnel: w1752 -> [w1844]
          tunnel: w1751 -> [w1843]
          tunnel: [w1897] -> w1778
          tunnel: [w1896] -> w1777
          tunnel: [w1895] -> w1776
          tunnel: [w1894] -> w1775
          tunnel: [w1893] -> w1774
          tunnel: [w1892] -> w1773
          tunnel: [w1899] -> w1772
          tunnel: [w1898] -> w1771
          tunnel: w1769 -> [w1899]
          tunnel: w1767 -> [w1898]
          tunnel: w1765 -> [w1897]
          tunnel: w1763 -> [w1896]
          tunnel: w1761 -> [w1895]
          tunnel: w1759 -> [w1894]
          tunnel: w1757 -> [w1893]
          tunnel: w1755 -> [w1892]
          frame #0 {
            n1044 = property on="X Scan" class="Bool (strict)"() -> ("Value"=w1787:bool)  [unwired: 2 in, 2 out]
            n1045 = property on="Y Scan" class="Bool (strict)"() -> ("Value"=w1788:bool)  [unwired: 2 in, 2 out]
            n1046 = property on="Z Scan" class="Bool (strict)"() -> ("Value"=w1789:bool)  [unwired: 2 in, 2 out]
            n1047 = property on="R Scan" class="Bool (strict)"() -> ("Value"=w1790:bool)  [unwired: 2 in, 2 out]
            n1048 = case shown="True" w1787 {
              tunnel: w1806 -> [w1826 w1830]
              tunnel: [w1826 w1829] -> w1797
              tunnel: w1805 -> [w1825 w1828]
              tunnel: [w1825 w1827] -> w1798
              frame False {
              }
              frame True {
                n1049 = property on="X Scan Length SP steps" class="DigNum (strict)"() -> ("Value"=w1831:i32)  [unwired: 2 in, 2 out]
                n1050 = Number To Decimal String(number=w1831) -> (decimal integer string=w1832:string)  [unwired: 1 in]
                n1051 = call "Applied Send Command.vi"("error in (no error)"=w1830, "Extra"=w1832, "Command"=T1."Distance or Position", "VISA resource name"=w1828) -> ("error out"=w1829:errorcluster, "VISA resource name out"=w1827:refnum<visa-resource-name>)  [unwired: 3 in, 1 out]
              }
            }
            n1052 = case shown="True" w1788 {
              tunnel: w1803 -> [w1835 w1840]
              tunnel: w1804 -> [w1834 w1839]
              tunnel: [w1834 w1836] -> w1795
              tunnel: [w1835 w1837] -> w1796
              frame False {
              }
              frame True {
                n1053 = property on="Y Scan Length SP steps" class="DigNum (strict)"() -> ("Value"=w1838:i32)  [unwired: 2 in, 2 out]
                n1054 = Number To Decimal String(number=w1838) -> (decimal integer string=w1841:string)  [unwired: 1 in]
                n1055 = call "Applied Send Command.vi"("error in (no error)"=w1839, "Extra"=w1841, "Command"=T1."Distance or Position", "VISA resource name"=w1840) -> ("error out"=w1836:errorcluster, "VISA resource name out"=w1837:refnum<visa-resource-name>)  [unwired: 3 in, 1 out]
              }
            }
            n1056 = case shown="True" w1789 {
              tunnel: w1802 -> [w1817 w1821]
              tunnel: [w1817 w1820] -> w1794
              tunnel: [w1816 w1819] -> w1793
              tunnel: w1801 -> [w1816 w1818]
              frame False {
              }
              frame True {
                n1057 = property on="Z Scan Length SP steps" class="DigNum (strict)"() -> ("Value"=w1822:i32)  [unwired: 2 in, 2 out]
                n1058 = Number To Decimal String(number=w1822) -> (decimal integer string=w1823:string)  [unwired: 1 in]
                n1059 = call "Applied Send Command.vi"("error in (no error)"=w1818, "Extra"=w1823, "Command"=T1."Distance or Position", "VISA resource name"=w1821) -> ("error out"=w1819:errorcluster, "VISA resource name out"=w1820:refnum<visa-resource-name>)  [unwired: 3 in, 1 out]
              }
            }
            n1060 = case shown="True" w1790 {
              tunnel: w1800 -> [w1808 w1813]
              tunnel: [w1808 w1812] -> w1792
              tunnel: w1799 -> [w1807 w1811]
              tunnel: [w1807 w1810] -> w1791
              frame False {
              }
              frame True {
                n1061 = property on="R Scan Length SP steps" class="DigNum (strict)"() -> ("Value"=w1809:i32)  [unwired: 2 in, 2 out]
                n1062 = Number To Decimal String(number=w1809) -> (decimal integer string=w1814:string)  [unwired: 1 in]
                n1063 = call "Applied Send Command.vi"("error in (no error)"=w1811, "Extra"=w1814, "Command"=T1."Distance or Position", "VISA resource name"=w1813) -> ("error out"=w1810:errorcluster, "VISA resource name out"=w1812:refnum<visa-resource-name>)  [unwired: 3 in, 1 out]
              }
            }
          }
          frame #1 {
            n1064 = case shown="True" w1843 {
              tunnel: w1862 -> [w1885 w1889]
              tunnel: [w1885 w1888] -> w1861
              tunnel: w1860 -> [w1884 w1887]
              tunnel: [w1884 w1886] -> w1859
              frame False {
              }
              frame True {
                n1065 = call "Applied Send Command.vi"("error in (no error)"=w1887, "Command"=T1."Feed to Length", "VISA resource name"=w1889) -> ("error out"=w1886:errorcluster, "VISA resource name out"=w1888:refnum<visa-resource-name>)  [unwired: 4 in, 1 out]
              }
            }
            n1066 = case shown="True" w1844 {
              tunnel: w1858 -> [w1878 w1882]
              tunnel: [w1878 w1881] -> w1857
              tunnel: w1856 -> [w1877 w1880]
              tunnel: [w1877 w1879] -> w1855
              frame False {
              }
              frame True {
                n1067 = call "Applied Send Command.vi"("error in (no error)"=w1880, "Command"=T1."Feed to Length", "VISA resource name"=w1882) -> ("error out"=w1879:errorcluster, "VISA resource name out"=w1881:refnum<visa-resource-name>)  [unwired: 4 in, 1 out]
              }
            }
            n1068 = case shown="False" w1845 {
              tunnel: w1854 -> [w1871 w1875]
              tunnel: [w1871 w1874] -> w1853
              tunnel: [w1870 w1873] -> w1852
              tunnel: w1851 -> [w1870 w1872]
              frame False {
              }
              frame True {
                n1069 = call "Applied Send Command.vi"("error in (no error)"=w1872, "Command"=T1."Feed to Length", "VISA resource name"=w1875) -> ("error out"=w1873:errorcluster, "VISA resource name out"=w1874:refnum<visa-resource-name>)  [unwired: 4 in, 1 out]
              }
            }
            n1070 = case shown="False" w1846 {
              tunnel: w1850 -> [w1864 w1868]
              tunnel: [w1864 w1867] -> w1849
              tunnel: w1848 -> [w1863 w1866]
              tunnel: [w1863 w1865] -> w1847
              frame False {
              }
              frame True {
                n1071 = call "Applied Send Command.vi"("error in (no error)"=w1866, "Command"=T1."Feed to Length", "VISA resource name"=w1868) -> ("error out"=w1865:errorcluster, "VISA resource name out"=w1867:refnum<visa-resource-name>)  [unwired: 4 in, 1 out]
              }
            }
          }
          frame #2 {
            n1072 = call "Time Delay7"("Delay Time (s)"=0.1) -> ()  [unwired: 10 in, 1 out]
            n1073 = property on="R Scan" class="Bool (strict)"("Val(Sgnl)"=FALSE ("Slew Ready 2")) -> ()  [unwired: 2 in, 2 out]
            n1074 = property on="Z Scan" class="Bool (strict)"("Val(Sgnl)"=FALSE ("Slew Ready 2")) -> ()  [unwired: 2 in, 2 out]
            n1075 = property on="X Scan" class="Bool (strict)"("Val(Sgnl)"=FALSE ("Slew Ready 2")) -> ()  [unwired: 2 in, 2 out]
            n1076 = property on="Y Scan" class="Bool (strict)"("Val(Sgnl)"=FALSE ("Slew Ready 2")) -> ()  [unwired: 2 in, 2 out]
            n1077 = property on="Z Scan Velocity SP steps/sec" class="DigNum (strict)"("DisabledEnum"=T2."Enabled" ("Disabled")) -> ()  [unwired: 2 in, 2 out]
            n1078 = property on="X Scan Length SP steps" class="DigNum (strict)"("DisabledEnum"=T2."Enabled" ("Disabled")) -> ()  [unwired: 2 in, 2 out]
            n1079 = property on="Y Scan Selocity SP steps/sec" class="DigNum (strict)"("DisabledEnum"=T2."Enabled" ("Disabled")) -> ()  [unwired: 2 in, 2 out]
            n1080 = property on="Z Scan Length SP steps" class="DigNum (strict)"("DisabledEnum"=T2."Enabled" ("Disabled")) -> ()  [unwired: 2 in, 2 out]
            n1081 = property on="Y Scan Length SP steps" class="DigNum (strict)"("DisabledEnum"=T2."Enabled" ("Disabled")) -> ()  [unwired: 2 in, 2 out]
            n1082 = property on="X Scan Velocity SP steps/sec" class="DigNum (strict)"("DisabledEnum"=T2."Enabled" ("Disabled")) -> ()  [unwired: 2 in, 2 out]
            n1083 = property on="R Scan Velocity SP steps/sec" class="DigNum (strict)"("DisabledEnum"=T2."Enabled" ("Disabled")) -> ()  [unwired: 2 in, 2 out]
            n1084 = property on="R Scan Length SP steps" class="DigNum (strict)"("DisabledEnum"=T2."Enabled" ("Disabled")) -> ()  [unwired: 2 in, 2 out]
            n1085 = property on="Scan Go" class="Bool"("DisabledEnum"=T2."Disabled and Grayed Out" ("Disabled")) -> ()  [unwired: 2 in, 2 out]
            n1086 = property on="Scan Cancel" class="Bool"("DisabledEnum"=T2."Disabled and Grayed Out" ("Disabled")) -> ()  [unwired: 2 in, 2 out]
          }
        }
      }
      event "Reset": Mouse Down {
        n1087 = event-data() -> ()  [unwired: 1 in, 7 out]
        n1088 = flat-sequence {
          tunnel: [w1944] -> w1923
          tunnel: w1924 -> [w1946]
          tunnel: [w1945] -> w1922
          tunnel: w1925 -> [w1947]
          frame #0 {
            n1089 = property on="Reset X Motor Steps" class="DigNum (strict)"() -> ("Value"=w1950:i32)  [unwired: 2 in, 2 out]
            n1090 = Number To Decimal String(number=w1950) -> (decimal integer string=w1948:string)  [unwired: 1 in]
            n1091 = call "Applied Send Command.vi"("error in (no error)"=w1946, "Extra"=w1948, "Command"=T1."Set ABS Position", "VISA resource name"=w1947) -> ("error out"=w1945:errorcluster, "VISA resource name out"=w1944:refnum<visa-resource-name>)  [unwired: 3 in, 1 out]
          }
        }
        n1092 = flat-sequence {
          tunnel: w1929 -> [w1955]
          tunnel: w1928 -> [w1952]
          tunnel: [w1954] -> w1927
          tunnel: [w1953] -> w1926
          frame #0 {
            n1093 = property on="Reset Y Motor Steps" class="DigNum (strict)"() -> ("Value"=w1957:i32)  [unwired: 2 in, 2 out]
            n1094 = Number To Decimal String(number=w1957) -> (decimal integer string=w1956:string)  [unwired: 1 in]
            n1095 = call "Applied Send Command.vi"("error in (no error)"=w1952, "Extra"=w1956, "Command"=T1."Set ABS Position", "VISA resource name"=w1955) -> ("error out"=w1953:errorcluster, "VISA resource name out"=w1954:refnum<visa-resource-name>)  [unwired: 3 in, 1 out]
          }
        }
        n1096 = flat-sequence {
          tunnel: [w1935] -> w1917
          tunnel: [w1934] -> w1916
          tunnel: w1919 -> [w1933]
          tunnel: w1918 -> [w1932]
          frame #0 {
            n1097 = property on="Reset R Motor Steps" class="DigNum (strict)"() -> ("Value"=w1936:i32)  [unwired: 2 in, 2 out]
            n1098 = Number To Decimal String(number=w1936) -> (decimal integer string=w1931:string)  [unwired: 1 in]
            n1099 = call "Applied Send Command.vi"("error in (no error)"=w1932, "Extra"=w1931, "Command"=T1."Set ABS Position", "VISA resource name"=w1933) -> ("error out"=w1934:errorcluster, "VISA resource name out"=w1935:refnum<visa-resource-name>)  [unwired: 3 in, 1 out]
          }
        }
        n1100 = flat-sequence {
          tunnel: [w1942] -> w1915
          tunnel: [w1941] -> w1914
          tunnel: w1921 -> [w1939]
          tunnel: w1920 -> [w1940]
          frame #0 {
            n1101 = property on="Reset Z Motor Steps" class="DigNum (strict)"() -> ("Value"=w1943:i32)  [unwired: 2 in, 2 out]
            n1102 = Number To Decimal String(number=w1943) -> (decimal integer string=w1937:string)  [unwired: 1 in]
            n1103 = call "Applied Send Command.vi"("error in (no error)"=w1940, "Extra"=w1937, "Command"=T1."Set ABS Position", "VISA resource name"=w1939) -> ("error out"=w1941:errorcluster, "VISA resource name out"=w1942:refnum<visa-resource-name>)  [unwired: 3 in, 1 out]
          }
        }
      }
    }
    n1104 = case shown="True" "Delete Button" {
      tunnel: w378 -> [_ w403]
      frame False {
      }
      frame True {
        n1105 = property on="Preset positions" class="Ring (strict)"() -> ("Value"=w401:i32)  [unwired: 2 in, 2 out]
        n1106 = Delete From Array(array=w403, index=w401) -> (array with subset deleted=w402:string[])  [unwired: 1 in, 1 out]
        n1107 = property on="Presets" class="Arr (strict)"() -> ("Value"=w400:i32[][])  [unwired: 2 in, 2 out]
        n1108 = property on="Preset positions" class="Ring (strict)"("Strings []"=w402) -> ()  [unwired: 2 in, 2 out]
        n1109 = Delete From Array(array=w400, index (row)=w401) -> (array with subset deleted=w399:i32[][])  [unwired: 2 in, 1 out]
        n1110 = property on="Presets" class="Arr (strict)"("Val(Sgnl)"=w399) -> ()  [unwired: 2 in, 2 out]
      }
    }
    n1111 = case shown="True" "Set Button" {
      tunnel: "Preset positions" -> [_ w421]
      frame False {
      }
      frame True {
        n1112 = property on="Presets" class="Arr (strict)"() -> ("Value"=w418:i32[][])  [unwired: 2 in, 2 out]
        n1113 = Index Array(array=w418, index (row)=w421) -> (element=w420:i32[])  [unwired: 1 in]
        n1114 = Array To Cluster(array=w420) -> (cluster=w419:T4)
        n1115 = Unbundle(w419) -> ("Value[0]"=w417:i32, "Value[1]"=w416:i32, "Value[2]"=w415:i32, "Value[3]"=w414:i32)  [unwired: 5 out]
        n1116 = property on="X Step SP" class="DigNum (strict)"("Val(Sgnl)"=w417) -> ()  [unwired: 2 in, 2 out]
        n1117 = property on="Y Step SP" class="DigNum (strict)"("Val(Sgnl)"=w416) -> ()  [unwired: 2 in, 2 out]
        n1118 = property on="Z Step SP" class="DigNum (strict)"("Val(Sgnl)"=w415) -> ()  [unwired: 2 in, 2 out]
        n1119 = property on="R Step SP" class="DigNum (strict)"("Val(Sgnl)"=w414) -> ()  [unwired: 2 in, 2 out]
      }
    }
    n1120 = case shown="True" "Add Button" {
      tunnel: w378 -> [_ w413]
      frame False {
      }
      frame True {
        n1121 = property on="X Step PV" class="DigNum (strict)"() -> ("Value"=w408:i32)  [unwired: 2 in, 2 out]
        n1122 = property on="Y Step PV" class="DigNum (strict)"() -> ("Value"=w407:i32)  [unwired: 2 in, 2 out]
        n1123 = property on="Z Step PV" class="DigNum (strict)"() -> ("Value"=w406:i32)  [unwired: 2 in, 2 out]
        n1124 = property on="R Step PV" class="DigNum (strict)"() -> ("Value"=w405:i32)  [unwired: 2 in, 2 out]
        n1125 = Build Array(w408, w407, w406, w405) -> (w411:i32[])
        n1126 = Build Array (concatenate)(w413, "String") -> (w412:string[])
        n1127 = property on="Preset positions" class="Ring (strict)"("Strings []"=w412) -> ()  [unwired: 2 in, 2 out]
        n1128 = property on="Presets" class="Arr (strict)"() -> ("Value"=w410:i32[][])  [unwired: 2 in, 2 out]
        n1129 = Build Array (concatenate)(w410, w411) -> (w404:i32[][])
        n1130 = property on="Presets" class="Arr (strict)"("Val(Sgnl)"=w404) -> ()  [unwired: 2 in, 2 out]
      }
    }
  }
  n1131 = flat-sequence {
    tunnel: w71 -> [w1959]
    tunnel: w70 -> [w1958]
    tunnel: [w1970] -> w47
    frame #0 {
      # "GET CURRENT POSITION"
      n1132 = call "Applied Send Command.vi"("error in (no error)"=w1958, "Extra"="", "Command"=T1."Immediate Position?", "VISA resource name"=w1959) -> ("error out"=w1960:errorcluster, "read buffer"=w1965:string, "VISA resource name out"=w1961:refnum<visa-resource-name>)  [unwired: 3 in]
      n1133 = call "Applied Send Command.vi"("error in (no error)"=w1960, "Command"=T1."Stop & Kill Buffer", "VISA resource name"=w1961) -> ("error out"=w1967:errorcluster, "VISA resource name out"=w1968:refnum<visa-resource-name>)  [unwired: 4 in, 1 out]
      n1134 = Hexadecimal String To Number(string=w1965, offset=3) -> (number=w1962:u32)  [unwired: 1 in, 1 out]
      n1135 = VISA Close(VISA resource name=w1968, error in (no error)=w1967) -> ()  [unwired: 1 out]
      n1136 = To Long Integer(number=w1962) -> (32bit integer=w1970:i32)
    }
  }
  n1137 = flat-sequence {
    tunnel: w51 -> [w1973]
    tunnel: w50 -> [w1972]
    tunnel: [w1971] -> w46
    frame #0 {
      # "GET CURRENT POSITION"
      n1138 = call "Applied Send Command.vi"("error in (no error)"=w1972, "Extra"="", "Command"=T1."Immediate Position?", "VISA resource name"=w1973) -> ("error out"=w1974:errorcluster, "read buffer"=w1979:string, "VISA resource name out"=w1975:refnum<visa-resource-name>)  [unwired: 3 in]
      n1139 = call "Applied Send Command.vi"("error in (no error)"=w1974, "Command"=T1."Stop & Kill Buffer", "VISA resource name"=w1975) -> ("error out"=w1981:errorcluster, "VISA resource name out"=w1982:refnum<visa-resource-name>)  [unwired: 4 in, 1 out]
      n1140 = Hexadecimal String To Number(string=w1979, offset=3) -> (number=w1976:u32)  [unwired: 1 in, 1 out]
      n1141 = VISA Close(VISA resource name=w1982, error in (no error)=w1981) -> ()  [unwired: 1 out]
      n1142 = To Long Integer(number=w1976) -> (32bit integer=w1971:i32)
    }
  }
  n1143 = flat-sequence {
    tunnel: w53 -> [w1985]
    tunnel: w52 -> [w1984]
    tunnel: [w1986] -> w45
    frame #0 {
      # "GET CURRENT POSITION"
      n1144 = call "Applied Send Command.vi"("error in (no error)"=w1984, "Extra"="", "Command"=T1."Immediate Position?", "VISA resource name"=w1985) -> ("error out"=w1987:errorcluster, "read buffer"=w1992:string, "VISA resource name out"=w1988:refnum<visa-resource-name>)  [unwired: 3 in]
      n1145 = call "Applied Send Command.vi"("error in (no error)"=w1987, "Command"=T1."Stop & Kill Buffer", "VISA resource name"=w1988) -> ("error out"=w1994:errorcluster, "VISA resource name out"=w1995:refnum<visa-resource-name>)  [unwired: 4 in, 1 out]
      n1146 = Hexadecimal String To Number(string=w1992, offset=3) -> (number=w1989:u32)  [unwired: 1 in, 1 out]
      n1147 = VISA Close(VISA resource name=w1995, error in (no error)=w1994) -> ()  [unwired: 1 out]
      n1148 = To Long Integer(number=w1989) -> (32bit integer=w1986:i32)
    }
  }
  n1149 = case shown="False" FALSE {
    tunnel: w49 -> [_ w2000]
    tunnel: w48 -> [_ w1999]
    tunnel: [0 w1998] -> w44
    frame False {
    }
    frame True {
      n1150 = flat-sequence {
        tunnel: w2000 -> [w2002]
        tunnel: w1999 -> [w2001]
        tunnel: [w2003] -> w1998
        frame #0 {
          # "GET CURRENT POSITION"
          n1151 = call "Applied Send Command.vi"("error in (no error)"=w2001, "Extra"="", "Command"=T1."Immediate Position?", "VISA resource name"=w2002) -> ("error out"=w2004:errorcluster, "read buffer"=w2009:string, "VISA resource name out"=w2005:refnum<visa-resource-name>)  [unwired: 3 in]
          n1152 = call "Applied Send Command.vi"("error in (no error)"=w2004, "Command"=T1."Stop & Kill Buffer", "VISA resource name"=w2005) -> ("error out"=w2011:errorcluster, "VISA resource name out"=w2012:refnum<visa-resource-name>)  [unwired: 4 in, 1 out]
          n1153 = Hexadecimal String To Number(string=w2009, offset=3) -> (number=w2006:u32)  [unwired: 1 in, 1 out]
          n1154 = VISA Close(VISA resource name=w2012, error in (no error)=w2011) -> ()  [unwired: 1 out]
          n1155 = To Long Integer(number=w2006) -> (32bit integer=w2003:i32)
        }
      }
    }
  }
  n1156 = flat-sequence {
    tunnel: w47 -> [w2019]
    tunnel: w46 -> [w2018]
    tunnel: w45 -> [w2017]
    tunnel: w44 -> [w2016]
    frame #0 {
      n1157 = Build Array(w2019, w2018, w2017, w2016) -> (w2014:i32[])
      n1158 = call-poly <vilib>:"Write To Spreadsheet File.vi"("1D data"=w2014, "file path (dialog if empty)"=path "S:/LV codes/SCL2/POS.TXT") -> ()  [unwired: 6 in, 1 out]
    }
    frame #1 {
      n1159 = property on="Presets" class="Arr (strict)"() -> ("Value"=w2026:i32[][])  [unwired: 2 in, 2 out]
      n1160 = property on="Preset positions" class="Ring (strict)"() -> ("Strings []"=w2022:string[])  [unwired: 2 in, 2 out]
      n1161 = Number To Decimal String(number=w2026) -> (decimal integer string=w2020:string[][])  [unwired: 1 in]
      n1162 = Transpose 2D Array(2D array=w2020) -> (transposed array=w2021:string[][])
      n1163 = Build Array (concatenate)(w2022, w2021) -> (w2023:string[][])
      n1164 = Transpose 2D Array(2D array=w2023) -> (transposed array=w2024:string[][])
      n1165 = call-poly <vilib>:"Write To Spreadsheet File.vi"("2D data"=w2024, "file path (dialog if empty)"=path "S:/LV codes/SCL2/PRESET.TXT") -> ()  [unwired: 6 in, 1 out]
    }
  }
